vi "Q14070-Z060A.vi"() -> ()   [LabVIEW 2013]
uses:
  <vilib>/Utility/error.llb/whitespace.ctl
  <vilib>/Utility/file.llb/Read From Spreadsheet File (string).vi
  <vilib>/express/express arith-compare/Formula/XNode/ExpressFormulaBlockNode.xnode
  PCI8622_32.dll
  <vilib>/printing/EasyPrintingControls.llb/contents.ctl
  <vilib>/Utility/NIReport.llb/NI_ReportGenerationCore.lvlib
  <vilib>/printing/EasyPrintingControls.llb/report_type.ctl
  <vilib>/Utility/NIReport.llb/NI_report.lvclass
  <vilib>/printing/EasyPrinting.llb/Easy Print VI Panel or Documentation (path).vi
panel:
  in  "电动缸快速":dbl=15.0
  in  "电动缸慢速":dbl=1.0
  out "左轴向力数组大小":i32
  out "循环退出":bool
  in  "截取百分比":dbl=0.05
  in  "半行程":dbl=70.0
  in  "是否取消放行按钮":bool
  in  "齿条传动比":dbl=47.34 format="%#_13g"
  in  "机械间隙值":dbl=3.5
  out "最大轴向力标准(N)":dbl=200.0 caption="L+Lmax(mm)" format="%#.3f"
  out "右平均轴向力(N)":dbl caption="L+Lmax(mm)" format="%#.3f"
  out "左平均轴向力(N)":dbl caption="最大位移偏离Lmax(mm)" format="%#.3f"
  out "员工ID":string
  out "急停":bool
  out "报警":dbl
  out "报警提示":string
  out "DeviceHandle":u32
  in  "设定轴向力调整次数":dbl=6.0
  out "出支线工步号":u32
  in  "最小间隙(mm)":dbl=0.001 format="%#.3f"
  in  "测头气缸右移":bool
  in  "测头气缸左移":bool
  in  "轴向力已做次数":dbl
  out "全行程间隙及轴向力合格":bool
  out "轴向力启动":bool
  out "间隙启动":bool
  in  "夹头松开":bool
  in  "夹头夹紧":bool
  out "找帽扭矩":dbl=10.0 caption="压力传感器" format="%#.2f"
  out "error out":errorcluster
  out "型号数量":i32
  out "error out 4":errorcluster
  in  "设定间隙调整次数":dbl=6.0
  out "读取产品ID":string
  out "下工位备料":bool
  out "下工位测试":bool
  out "下工位自动":bool
  out "下工位备料H":bool
  out "下工位测试H":bool
  out "下工位自动H":bool
  out "FGCS":string
  out "KSJJ":string
  out "Z060ARFID":string
  out "轴向力Y":dbl[](array[numeric])
  out "轴向力X":dbl[](array[numeric])
  out "间隙X数组":dbl[](array[numeric])
  out "间隙Y数组":dbl[](array[numeric])
  out "error out 3":errorcluster caption="错误输出"
  out "rfid工步号":u32
  out "芯片ID":string="201209190001"
  out "rfid完成":bool
  out "rfid触发":bool
  out "本序已做":bool
  in  "回零完成":bool
  in  "电动缸回零":bool
  in  "已调试次数":dbl
  in  "需调整角度(度)":dbl
  in  "转向器中心":dbl
  out "扭矩到达":bool
  out "黄灯":bool
  out "红灯":bool
  in  "基准位移":dbl caption="压力传感器" format="%#.3f"
  out "上序不合格":bool
  out "单点间隙合格":bool
  out "上序合格":bool
  out "测头机构电机":u32
  out "复位":bool
  in  "型号选择":u16(ring)=1 items=["J709", "J728", "J706"]
  in  "联线按钮":bool
  in  "工步号":u32
  in  "产品ID":string="201209190001"
  out "间隙位移(mm)":dbl caption="压力传感器" format="%#.3f"
  out "齿条推拉力(N)":dbl format="%#.2f"
  out "齿条扭矩(Nm)":dbl format="%#.2f"
  out "通讯状态":bool
  out "员工姓名":string
  out "工步提示":string
  out "ADODB._Connection Out 2":refnum<k7>
  out "旋转齿条电机":u32
  out "电动缸电机":u32
  in  "停止":bool
  in  "参数加载":bool
  in  "选项卡控件":T1(tab)
  out "扭动曲线":cluster{"Y":dbl[], "Y":dbl[]}[](graph) caption="压球涨堵头1"
  out "中间位置间隙":dbl caption="间隙值L(mm)" format="%_2f"
  out "中间间隙标准(mm)":dbl=0.07 format="%#.3f"
  in  "找帽OK":bool
  out "全行程180°外间隙标准(mm)":dbl=0.1 format="%#.3f"
  out "右180°外全行程间隙":dbl caption="正向最大间隙L1(mm)" format="%_2f"
  out "左180°外全行程间隙":dbl caption="正向最大间隙L1(mm)" format="%_2f"
  out "右180°内全行程间隙":dbl caption="正向最大间隙L1(mm)" format="%_2f"
  out "左180°内全行程间隙":dbl caption="正向最大间隙L1(mm)" format="%_2f"
  out "全行程180°内间隙标准(mm)":dbl=0.07 format="%_1f"
  out "左全行程间隙":dbl caption="正向最大间隙L1(mm)" format="%#.3f"
  out "右全行程间隙":dbl caption="正向最大间隙L1(mm)" format="%#.3f"
  out "总圈数最大值":dbl format="%_3g"
  out "总圈数标准":dbl format="%_3g"
  out "总行程最大值":dbl
  out "总行程标准(mm)":dbl
  out "平均轴向力MAX(N)":dbl=200.0 caption="L+Lmax(mm)" format="%#.3f"
  out "力波动标准(N)":dbl=60.0 caption="L+Lmax(mm)" format="%#.3f"
  out "轴向力标准(N)":dbl=100.0 caption="L+Lmax(mm)" format="%#.3f"
  out "右最大轴向力(N)":dbl caption="L+Lmax(mm)" format="%#_5f"
  out "左轴向力波动(N)":dbl caption="最大位移偏离Lmax(mm)" format="%#_4f"
  out "左最大轴向力(N)":dbl caption="最大位移偏离Lmax(mm)" format="%#_5f"
  out "行程跳动曲线":cluster{"Y":dbl[], "Y":dbl[]}[](graph) caption="压球涨堵头1"
  out "右轴向力波动(N)":dbl format="%#_4f"
  out "总行程(mm)":dbl format="%#_5f"
  out "总圈数":dbl format="%.3g"
  in  "不合格品":bool
  in  "扭矩停止值":dbl=16.0
  in  "齿条右极限":dbl=-70.0 caption="压力传感器" format="%#.2f"
  in  "齿条左极限":dbl=-262.0 caption="压力传感器" format="%#.2f"
  in  "齿条移动速度":dbl=5.0 caption="压力传感器" format="%#.2f"
  in  "旋转伺服找帽转速":dbl=5.0 caption="压力传感器" format="%#.2f"
  in  "测量点扭矩":dbl=4.0 caption="压力传感器" format="%#.2f"
  in  "旋转伺服测量转速":dbl caption="压力传感器" format="%#.2f"
  in  "测头机构轴后退位":dbl=30.0 caption="压力传感器" format="%#.2f"
  in  "测头机构轴待检位":dbl caption="压力传感器" format="%#.2f"
  in  "测头机构轴检测位":dbl caption="压力传感器" format="%#.2f"
  in  "测头机构轴移动速度":dbl caption="压力传感器" format="%#.2f"
  out "点胶":bool
  in  "夹头松开":bool
  in  "夹头夹紧":bool
  in  "测头气缸右移":bool
  in  "测头气缸左移":bool
  in  "支线下降":bool
  in  "支线顶升":bool
  in  "出支线":bool
  in  "进支线":bool
  in  "主线下降":bool
  in  "主线顶升":bool
  in  "下阻挡器放行":bool
  in  "上阻挡器放行":bool
  out "夹头夹紧位":bool
  out "测头左位":bool
  out "测头右位":bool
  out "夹头松开":bool
  out "记号笔":bool
  in  "测头机构轴使能":bool
  in  "测头机构轴后退":bool
  in  "测头机构轴前进":bool
  in  "电动缸速度(mm/s)":dbl=10.0 format="%#.3f"
  out "电动缸位置(mm)":dbl=10000.0 format="%#.3f"
  in  "旋转伺服速度(°/s)":dbl=10.0 format="%#.3f"
  out "旋转伺服位置(°)":dbl=10000.0 format="%#.3f"
  in  "测头机构轴速度(mm/s)":dbl=10.0 format="%#.3f"
  out "测头机构轴位置(mm)":dbl=10000.0 format="%#.3f"
  in  "旋转齿条轴右转":bool
  in  "旋转齿条轴左转":bool
  in  "旋转齿条轴使能":bool
  in  "电动缸后退":bool
  in  "电动缸使能":bool
  in  "电动缸前进":bool
  in  "齿条扭矩比例偏移":dbl=1.0 format="%#.2f"
  in  "齿条扭矩零点偏移":dbl format="%#.2f"
  in  "齿条推拉力比例偏移":dbl=1.0 format="%#.2f"
  in  "齿条推拉力零点偏移":dbl format="%#.2f"
  in  "间隙位移比例偏移":dbl=1.0 format="%#.2f"
  in  "间隙位移零点偏移":dbl format="%#.2f"
  in  "传感器参数保存":bool
  in  "参数修改":bool
  in  "参数查询":bool
  in  "参数浏览表":string[][](table)
  # "芜湖机械转向器装配线"
  # "间隙及轴向力检测"
  # "Q14070机械转向器装配线"
  # "湖北唯思凌科装备制造有限公司 设计开发 (C)2015"
  # "≤"
  # "间隙测量判定值"
  # "间隙测量结果"
  # "≤"
  # "≤"
  # "≤"
  # "轴向力测量结果"
  # "轴向力测量标准"
  # "≤"
  # "≥"
  # "≤"
  # "≥"
  # "≤"
  # "≥"
  # "≤"
  # "不得大于20NM"
  # "传感器校验区"
  # "关于传感器校验：\n1、传感器校验需要由具备资质的单位或部门进行校验。\n2、具备权限的用户才能够修改传感器校验参数和试验参数。\n3、修改校验参数方法：先将比例偏移置为1，修改零点偏移，使零点值与校验的传感器一致；然后根据增幅调整比例偏移。"
  # "注意：\n具备权限的用户才能够修改传感器校验参数和试验参数！"
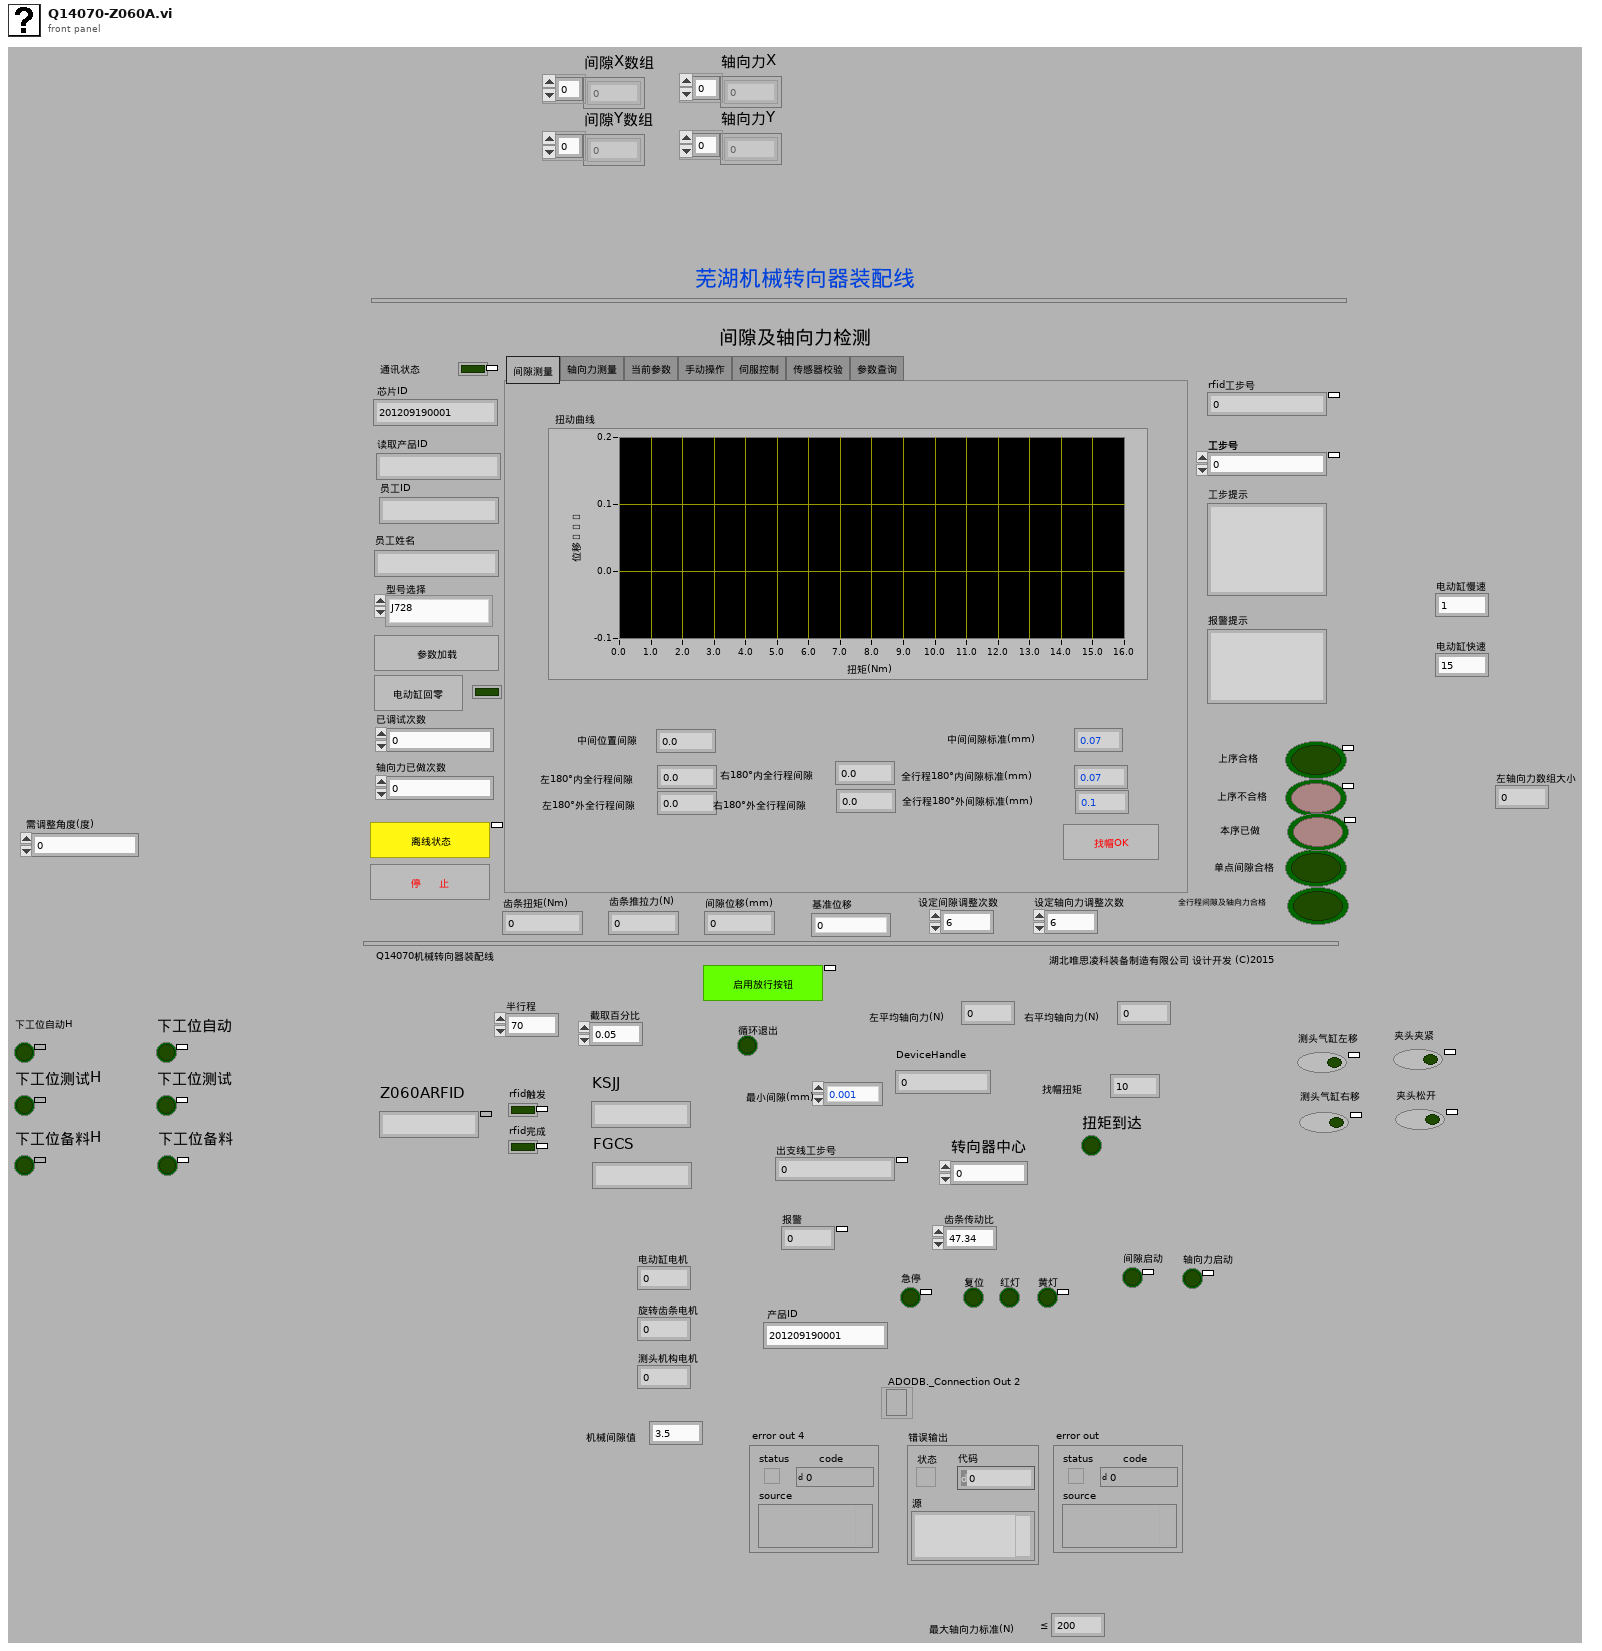
[diagram p1: front panel]
types:
  T1 = enum32{"间隙测量", "轴向力测量", "当前参数", "手动操作", "伺服控制", "传感器校验", "参数查询"}
  T2 = typedef "NI_ReportGenerationCore.lvlib/report_type.ctl" = u16
  T3 = typedef "NI_ReportGenerationCore.lvlib/contents.ctl" = u16
  T4 = typedef "imagedata.ctl" = cluster{"image type":i32, "image depth":i32, "image":u8[], "mask":u8[], "colors":u32[], "Rectangle":cluster{"left":i16, "top":i16, "right":i16, "bottom":i16}}
  T5 = enum8{"Enabled", "Disabled", "Disabled and Grayed Out"}
  T6 = typedef "whitespace.ctl" = u16
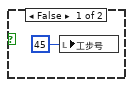
[diagram p2: hidden frame]
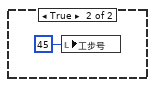
[diagram p3: hidden frame]
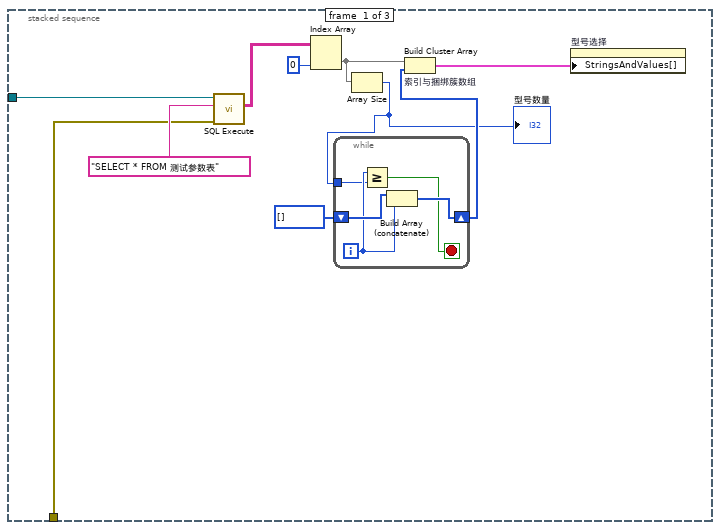
[diagram p6: hidden frame]
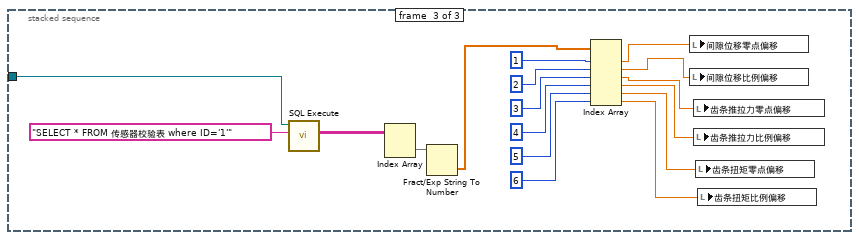
[diagram p7: hidden frame]
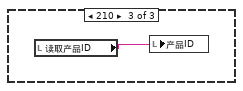
[diagram p9: hidden frame]
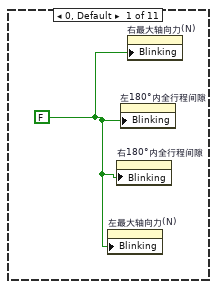
[diagram p10: hidden frame]
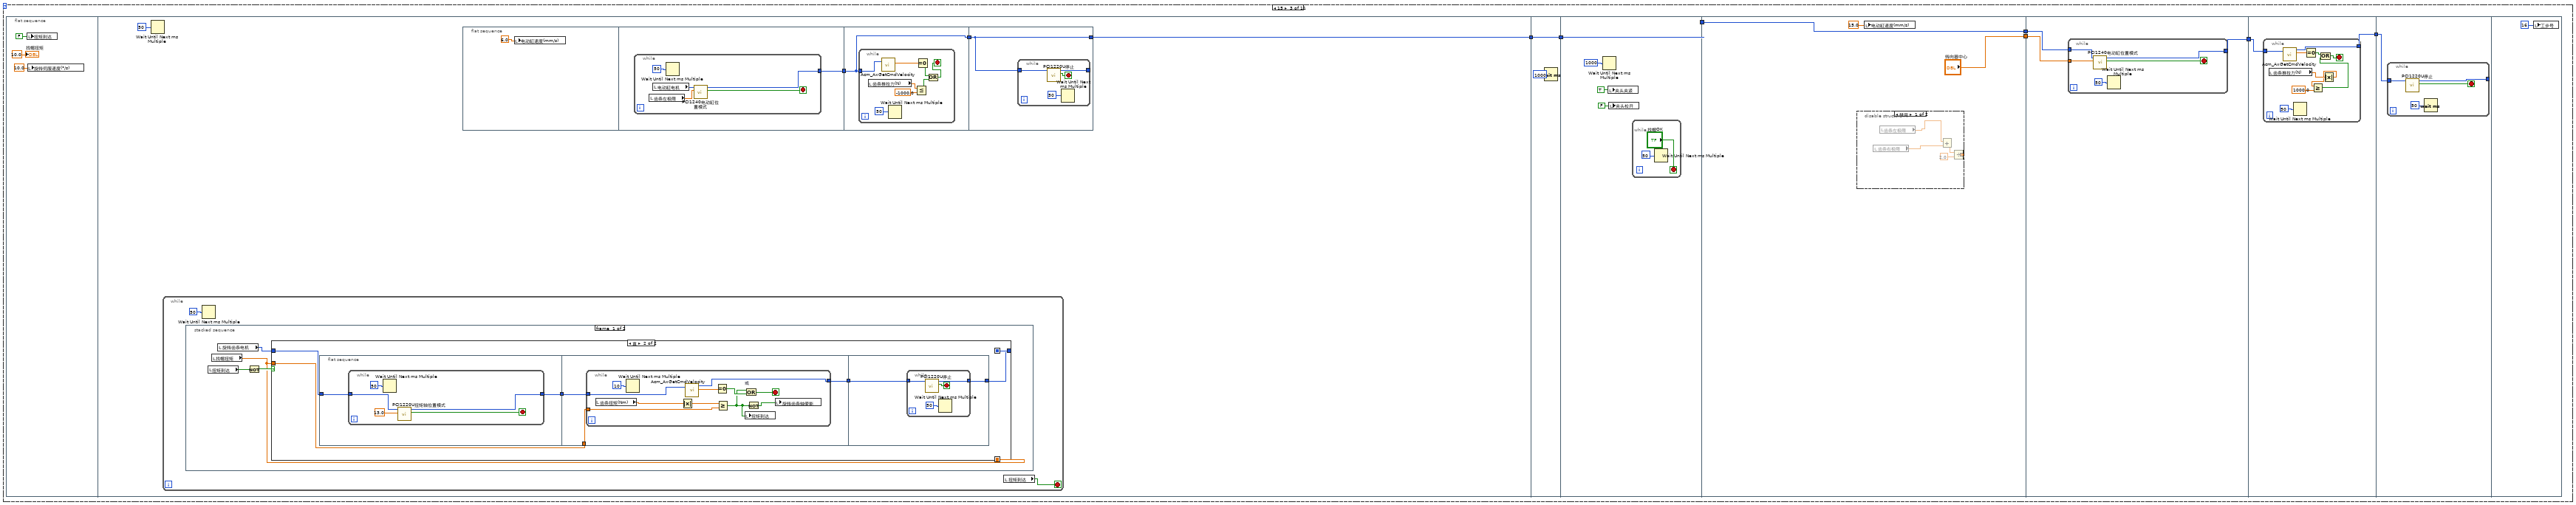
[diagram p11: hidden frame]
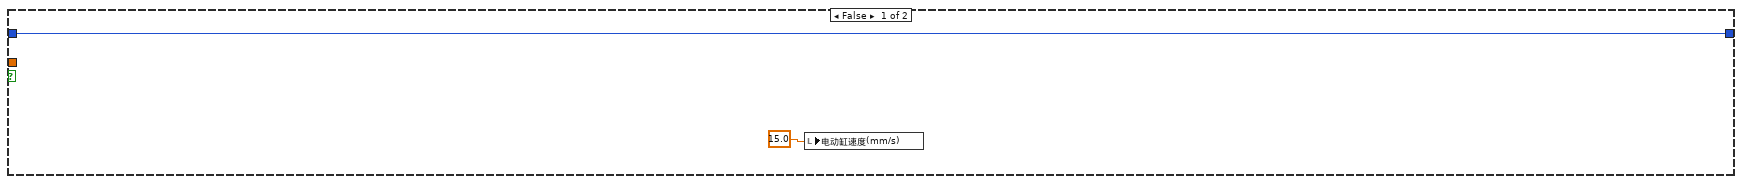
[diagram p12: hidden frame]
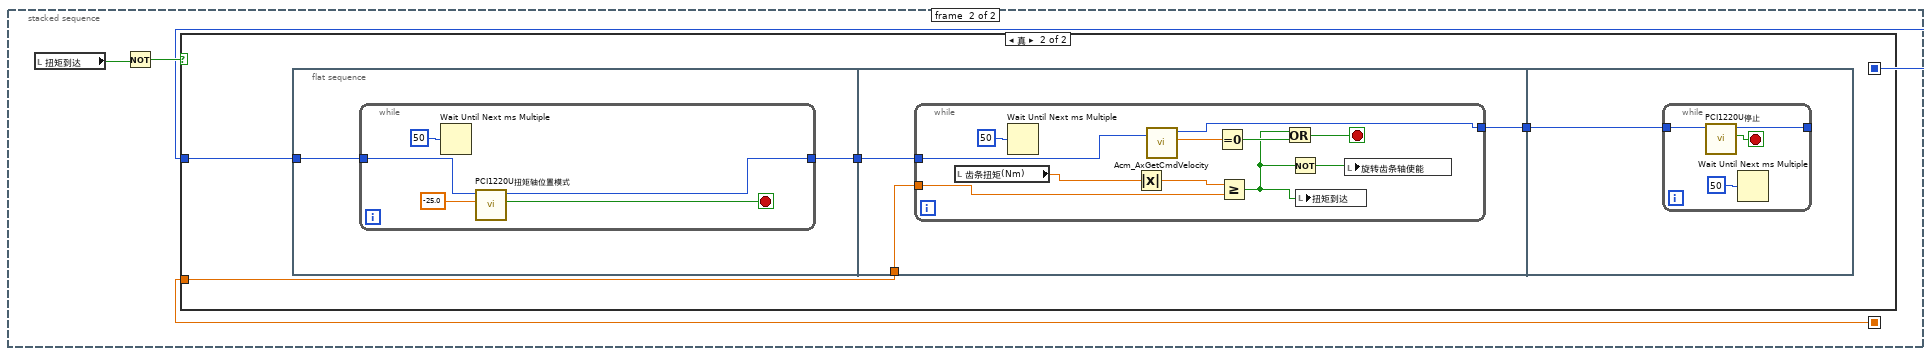
[diagram p13: hidden frame]
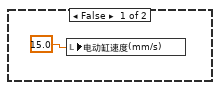
[diagram p14: hidden frame]
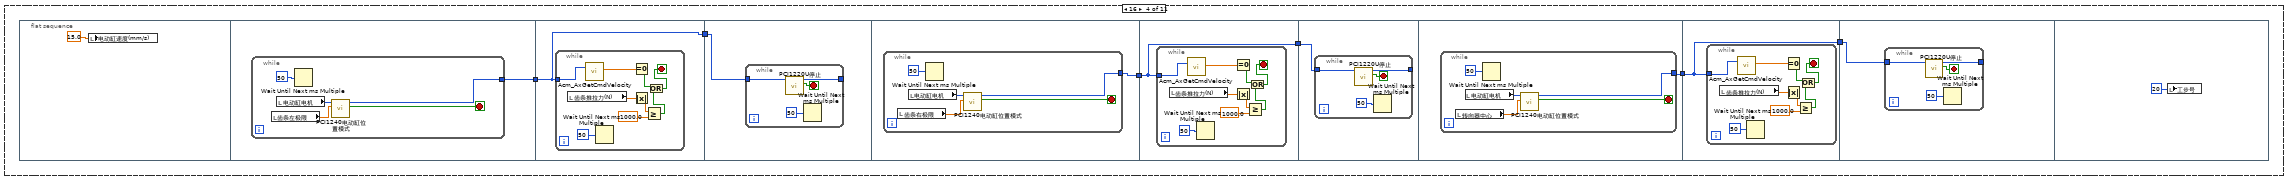
[diagram p16: hidden frame]
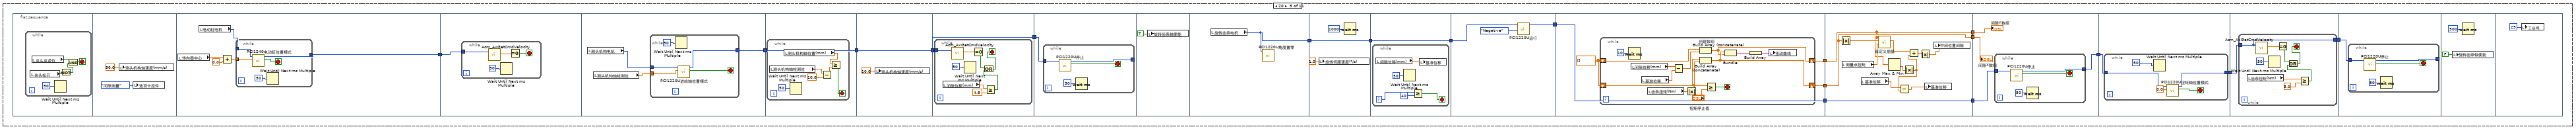
[diagram p17: hidden frame]
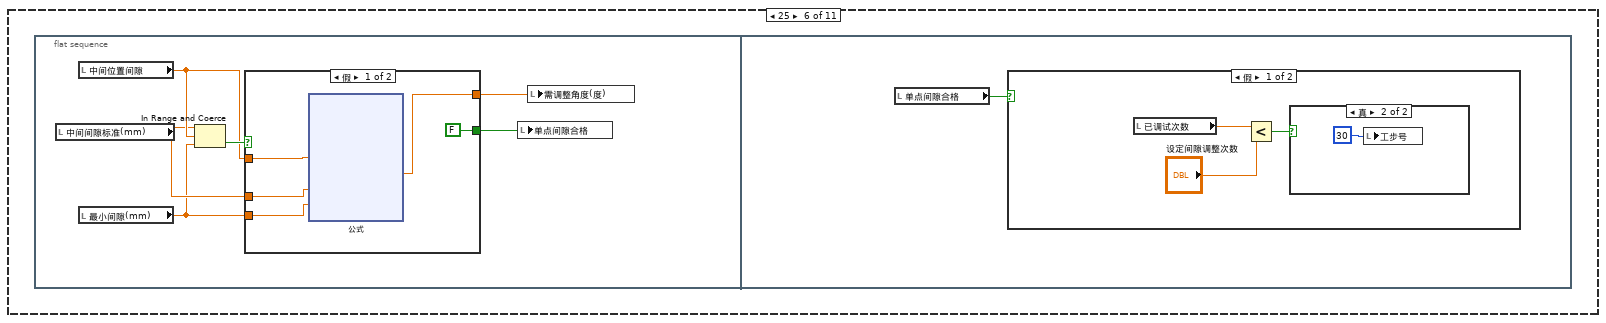
[diagram p18: hidden frame]
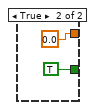
[diagram p19: hidden frame]
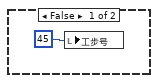
[diagram p20: hidden frame]
diagram:
  n1 = while {
    stop <- w133 stop-if-true
    n2 = local read "工步号"() -> (w131:u32)
    n3 = case shown="10" w131 {
      frame 0, Default {
        w134 = FALSE ("闪烁")
        n4 = property on="左最大轴向力(N)" class="DigNum (严格)"("Blinking"=w134) -> ()  [unwired: 2 in, 2 out]
        n5 = property on="右180°内全行程间隙" class="DigNum (严格)"("Blinking"=w134) -> ()  [unwired: 2 in, 2 out]
        n6 = property on="左180°内全行程间隙" class="DigNum (严格)"("Blinking"=w134) -> ()  [unwired: 2 in, 2 out]
        n7 = property on="右最大轴向力(N)" class="DigNum (严格)"("Blinking"=w134) -> ()  [unwired: 2 in, 2 out]
      }
      frame 10 {
        n8 = flat-sequence {
          frame #0 {
            w135 = FALSE ("单点间隙合格")
            w136 = 0.0 ("已调试次数")
            n9 = local write "电动缸速度(mm/s)"(10.0 ("电动缸速度(mm/s)")) -> ()
            n10 = local write "电动缸使能"(TRUE ("电动缸使能")) -> ()
            n11 = local write "旋转齿条轴使能"(TRUE ("旋转齿条轴使能")) -> ()
            n12 = local write "测头机构轴使能"(TRUE ("调整机构轴使能")) -> ()
            n13 = local write "旋转伺服速度(°/s)"(10.0 ("旋转齿条轴速度(°/s)")) -> ()
            n14 = local write "测头机构轴速度(mm/s)"(30.0 ("调整机构轴速度(mm/s)")) -> ()
            n15 = local write "已调试次数"(w136) -> ()
            n16 = local write "轴向力已做次数"(w136) -> ()
            n17 = property on="右180°外全行程间隙" class="DigNum (严格)"("Blinking"=w135) -> ()  [unwired: 2 in, 2 out]
            n18 = property on="左180°内全行程间隙" class="DigNum (严格)"("Blinking"=w135) -> ()  [unwired: 2 in, 2 out]
            n19 = property on="右180°内全行程间隙" class="DigNum (严格)"("Blinking"=w135) -> ()  [unwired: 2 in, 2 out]
            n20 = property on="左180°外全行程间隙" class="DigNum (严格)"("Blinking"=w135) -> ()  [unwired: 2 in, 2 out]
            n21 = property on="总行程(mm)" class="DigNum (严格)"("Blinking"=w135) -> ()  [unwired: 2 in, 2 out]
            n22 = local write "全行程间隙及轴向力合格"(w135) -> ()
            n23 = local write "单点间隙合格"(w135) -> ()
            n24 = local write "测头气缸右移"(TRUE ("测头气缸右移")) -> ()
            n25 = local write "测头气缸左移"(FALSE ("测头气缸左移")) -> ()
            n26 = property on="总圈数" class="DigNum (严格)"("Blinking"=w135) -> ()  [unwired: 2 in, 2 out]
            n27 = property on="左最大轴向力(N)" class="DigNum (严格)"("Blinking"=w135) -> ()  [unwired: 2 in, 2 out]
            n28 = property on="右最大轴向力(N)" class="DigNum (严格)"("Blinking"=w135) -> ()  [unwired: 2 in, 2 out]
            n29 = property on="右轴向力波动(N)" class="DigNum (严格)"("Blinking"=w135) -> ()  [unwired: 2 in, 2 out]
            n30 = property on="左轴向力波动(N)" class="DigNum (严格)"("Blinking"=w135) -> ()  [unwired: 2 in, 2 out]
          }
          frame #1 {
            n31 = while {
              stop <- w145 stop-if-true
              n32 = Wait Until Next ms Multiple(millisecond multiple=u32 50 ("毫秒倍数")) -> ()  [unwired: 1 out]
              n33 = local read "测头右位"() -> (w146:bool)
              n34 = local read "回零完成"() -> (w147:bool)
              n35 = And(x=w147, y=w146) -> (x .and. y?=w145:bool)
            }
          }
          frame #2 {
            n36 = Wait (ms)(milliseconds to wait=u32 1000 ("等待时间（毫秒）")) -> ()  [unwired: 1 out]
          }
          frame #3 {
            n37 = while {
              stop <- w153 stop-if-true
              n38 = local read "测头机构轴待检位"() -> (w150:dbl)
              n39 = local read "测头机构电机"() -> (w151:u32)
              n40 = call "PCI1220U进给轴位置模式.vi"("Distance"=w150, "AxisHandle IN"=w151) -> ("AbsSuccess"=w153:bool)  [unwired: 8 in, 1 out]
              n41 = Wait Until Next ms Multiple(millisecond multiple=u32 50 ("毫秒倍数")) -> ()  [unwired: 1 out]
            }
          }
          frame #4 {
            n42 = while {
              stop <- w156 stop-if-true
              n43 = local read "测头机构电机"() -> (w154:u32)
              n44 = Wait Until Next ms Multiple(millisecond multiple=u32 50 ("毫秒倍数")) -> ()  [unwired: 1 out]
              n45 = call <userlib>:"Acm_AxGetCmdVelocity.vi"("AxisHandle"=w154) -> ("Velocity"=w157:dbl)  [unwired: 1 in, 3 out]
              n46 = Equal To 0?(x=w157) -> (x = 0?=w156:bool)
            }
          }
          frame #5 {
            n47 = local write "工步号"(u32 15 ("工步号")) -> ()
          }
        }
      }
      frame 15 {
        n48 = flat-sequence {
          tunnel: [w170] -> w160
          tunnel: w160 -> [w271]
          tunnel: [w271] -> w159
          tunnel: w159 -> [w274]
          tunnel: [w274] -> w162
          tunnel: [w279] -> w165
          tunnel: ["转向器中心"] -> w164
          tunnel: w162 -> [w279]
          tunnel: w165 -> [w288]
          tunnel: w164 -> [w287]
          tunnel: [w286] -> w163
          tunnel: w163 -> [w295]
          tunnel: [w294] -> w161
          tunnel: w161 -> [w306]
          frame #0 {
            n49 = local write "扭矩到达"(FALSE ("扭矩到达")) -> ()
            n50 = local write "旋转伺服速度(°/s)"(10.0 ("旋转齿条轴速度(°/s)")) -> ()
            "找帽扭矩" <- 10.0 ("找帽扭矩")
          }
          frame #1 {
            n51 = Wait Until Next ms Multiple(millisecond multiple=u32 50 ("毫秒倍数")) -> ()  [unwired: 1 out]
            n52 = while {
              stop <- w173 stop-if-true
              n53 = stacked-sequence {
                seq-local: [w175 _] -> [_ w216]
                seq-local: [w179 _] -> [_ w215]
                frame #0 {
                  n54 = local read "扭矩到达"() -> (w177:bool)
                  n55 = local read "找帽扭矩"() -> (w175:dbl)
                  n56 = local read "旋转齿条电机"() -> (w176:u32)
                  n57 = Not(x=w177) -> (.not. x?=w178:bool)
                  n58 = case shown="真" w178 {
                    tunnel: [w181 w182] -> w179
                    tunnel: w176 -> [w181 w186]
                    tunnel: w175 -> [_ w184]
                    frame False {
                      n59 = local write "电动缸速度(mm/s)"(15.0 ("电动缸速度(mm/s)")) -> ()
                    }
                    frame True {
                      n60 = flat-sequence {
                        tunnel: w186 -> [w188]
                        tunnel: [w187] -> w185
                        tunnel: w185 -> [w196]
                        tunnel: w184 -> [w195]
                        tunnel: [w194] -> w183
                        tunnel: w183 -> [w209]
                        tunnel: [w208] -> w182
                        frame #0 {
                          n61 = while {
                            tunnel: [w192] -> w187
                            tunnel: w188 -> [w189]
                            stop <- w191 stop-if-true
                            n62 = Wait Until Next ms Multiple(millisecond multiple=u32 50 ("毫秒倍数")) -> ()  [unwired: 1 out]
                            n63 = call "PCI1220U扭矩轴位置模式.vi"("Distance"=13.0, "AxisHandle IN"=w189) -> ("AbsSuccess"=w191:bool, "AxisHandle OUT"=w192:u32)  [unwired: 8 in]
                          }
                        }
                        frame #1 {
                          n64 = while {
                            tunnel: w196 -> [w206]
                            tunnel: w195 -> [w201]
                            tunnel: [w200] -> w194
                            stop <- w202 stop-if-true
                            n65 = local read "齿条扭矩(Nm)"() -> (w199:dbl)
                            n66 = Wait Until Next ms Multiple(millisecond multiple=u32 10 ("毫秒倍数")) -> ()  [unwired: 1 out]
                            n67 = Absolute Value(x=w199) -> (abs(x)=w204:dbl)
                            n68 = call <userlib>:"Acm_AxGetCmdVelocity.vi"("AxisHandle"=w206) -> ("Velocity"=w205:dbl, "AxisHandle"=w200:u32)  [unwired: 1 in, 2 out]
                            n69 = Equal To 0?(x=w205) -> (x = 0?=w203:bool)
                            n70 = Greater Or Equal?(x=w204, y=w201) -> (x >= y?=w198:bool)
                            n71 = Or "或"(x=w198, y=w203) -> (x .or. y?=w202:bool)
                            n72 = local write "扭矩到达"(w198) -> ()
                            n73 = Not(x=w198) -> (.not. x?=w197:bool)
                            n74 = local write "旋转齿条轴使能"(w197) -> ()
                          }
                        }
                        frame #2 {
                          n75 = while {
                            tunnel: w209 -> [w213]
                            tunnel: [w210] -> w208
                            stop <- w212 stop-if-true
                            n76 = call "PCI1220U停止.vi"("AxisHandle IN"=w213) -> ("完成"=w212:bool, "AxisHandle OUT"=w210:u32)  [unwired: 9 in]
                            n77 = Wait Until Next ms Multiple(millisecond multiple=u32 50 ("毫秒倍数")) -> ()  [unwired: 1 out]
                          }
                        }
                      }
                    }
                  }
                }
                frame #1 {
                  n78 = local read "扭矩到达"() -> (w214:bool)
                  n79 = Not(x=w214) -> (.not. x?=w217:bool)
                  n80 = case shown="真" w217 {
                    tunnel: w215 -> [_ w222]
                    tunnel: w216 -> [_ w220]
                    frame False {
                      n81 = local write "电动缸速度(mm/s)"(15.0 ("电动缸速度(mm/s)")) -> ()
                    }
                    frame True {
                      n82 = flat-sequence {
                        tunnel: w222 -> [w223]
                        tunnel: [w224] -> w221
                        tunnel: w221 -> [w232]
                        tunnel: w220 -> [w231]
                        tunnel: [w230] -> w219
                        tunnel: w219 -> [w244]
                        frame #0 {
                          n83 = while {
                            tunnel: [w228] -> w224
                            tunnel: w223 -> [w225]
                            stop <- w227 stop-if-true
                            n84 = Wait Until Next ms Multiple(millisecond multiple=u32 50 ("毫秒倍数")) -> ()  [unwired: 1 out]
                            n85 = call "PCI1220U扭矩轴位置模式.vi"("Distance"=-25.0, "AxisHandle IN"=w225) -> ("AbsSuccess"=w227:bool, "AxisHandle OUT"=w228:u32)  [unwired: 8 in]
                          }
                        }
                        frame #1 {
                          n86 = while {
                            tunnel: w232 -> [w242]
                            tunnel: [w237] -> w230
                            tunnel: w231 -> [w236]
                            stop <- w238 stop-if-true
                            n87 = local read "齿条扭矩(Nm)"() -> (w235:dbl)
                            n88 = Wait Until Next ms Multiple(millisecond multiple=u32 50 ("毫秒倍数")) -> ()  [unwired: 1 out]
                            n89 = Absolute Value(x=w235) -> (abs(x)=w240:dbl)
                            n90 = call <userlib>:"Acm_AxGetCmdVelocity.vi"("AxisHandle"=w242) -> ("Velocity"=w241:dbl, "AxisHandle"=w237:u32)  [unwired: 1 in, 2 out]
                            n91 = Equal To 0?(x=w241) -> (x = 0?=w239:bool)
                            n92 = Greater Or Equal?(x=w240, y=w236) -> (x >= y?=w233:bool)
                            n93 = Or(x=w233, y=w239) -> (x .or. y?=w238:bool)
                            n94 = Not(x=w233) -> (.not. x?=w234:bool)
                            n95 = local write "扭矩到达"(w233) -> ()
                            n96 = local write "旋转齿条轴使能"(w234) -> ()
                          }
                        }
                        frame #2 {
                          n97 = while {
                            tunnel: w244 -> [w248]
                            tunnel: [w245] -> _
                            stop <- w247 stop-if-true
                            n98 = call "PCI1220U停止.vi"("AxisHandle IN"=w248) -> ("完成"=w247:bool, "AxisHandle OUT"=w245:u32)  [unwired: 9 in]
                            n99 = Wait Until Next ms Multiple(millisecond multiple=u32 50 ("毫秒倍数")) -> ()  [unwired: 1 out]
                          }
                        }
                      }
                    }
                  }
                }
              }
              n100 = Wait Until Next ms Multiple(millisecond multiple=u32 50 ("毫秒倍数")) -> ()  [unwired: 1 out]
              n101 = local read "扭矩到达"() -> (w173:bool)
            }
            n102 = flat-sequence {
              tunnel: [w250] -> w172
              tunnel: w172 -> [w256]
              tunnel: [w256] -> w169
              tunnel: [w265] -> w170
              tunnel: w169 -> [w265]
              frame #0 {
                n103 = local write "电动缸速度(mm/s)"(6.0 ("电动缸速度(mm/s)")) -> ()
              }
              frame #1 {
                n104 = while {
                  tunnel: [w254] -> w250
                  stop <- w253 stop-if-true
                  n105 = local read "齿条左极限"() -> (w251:dbl)
                  n106 = local read "电动缸电机"() -> (w255:u32)
                  n107 = Wait Until Next ms Multiple(millisecond multiple=u32 50 ("毫秒倍数")) -> ()  [unwired: 1 out]
                  n108 = call "PCI1240电动缸位置模式 .vi"("Distance"=w251, "AxisHandle IN"=w255) -> ("AbsSuccess"=w253:bool, "AxisHandle OUT"=w254:u32)  [unwired: 8 in]
                }
              }
              frame #2 {
                n109 = while {
                  tunnel: w256 -> [w263]
                  stop <- w260 stop-if-true
                  n110 = local read "齿条推拉力(N)"() -> (w259:dbl)
                  n111 = call <userlib>:"Acm_AxGetCmdVelocity.vi"("AxisHandle"=w263) -> ("Velocity"=w264:dbl)  [unwired: 1 in, 3 out]
                  n112 = Wait Until Next ms Multiple(millisecond multiple=u32 50 ("毫秒倍数")) -> ()  [unwired: 1 out]
                  n113 = Less Or Equal?(x=w259, y=-1000.0) -> (x <= y?=w257:bool)
                  n114 = Equal To 0?(x=w264) -> (x = 0?=w261:bool)
                  n115 = Or(x=w261, y=w257) -> (x .or. y?=w260:bool)
                }
              }
              frame #3 {
                n116 = while {
                  tunnel: w265 -> [w269]
                  tunnel: [w266] -> _
                  stop <- w268 stop-if-true
                  n117 = call "PCI1220U停止.vi"("AxisHandle IN"=w269) -> ("完成"=w268:bool, "AxisHandle OUT"=w266:u32)  [unwired: 9 in]
                  n118 = Wait Until Next ms Multiple(millisecond multiple=u32 50 ("毫秒倍数")) -> ()  [unwired: 1 out]
                }
              }
            }
          }
          frame #2 {
            n119 = Wait (ms)(milliseconds to wait=u32 1000 ("等待时间（毫秒）")) -> ()  [unwired: 1 out]
          }
          frame #3 {
            n120 = Wait Until Next ms Multiple(millisecond multiple=u32 1000 ("毫秒倍数")) -> ()  [unwired: 1 out]
            n121 = local write "夹头夹紧"(TRUE ("夹头夹紧")) -> ()
            n122 = local write "夹头松开"(FALSE ("夹头松开")) -> ()
            n123 = while {
              stop <- "找帽OK" stop-if-true
              n124 = Wait Until Next ms Multiple(millisecond multiple=u32 50 ("毫秒倍数")) -> ()  [unwired: 1 out]
            }
          }
          frame #4 {
            n125 = disable-structure shown="禁用" {
              disable-tunnel: [w283 _] -> _
              frame Disabled {
                n126 = local read "齿条右极限"() -> (w281:dbl)
                n127 = local read "齿条左极限"() -> (w282:dbl)
                n128 = Add(x=w282, y=w281) -> (x+y=w285:dbl)
                n129 = Divide(x=w285, y=2.0) -> (x/y=w283:dbl)
              }
              frame Enabled {
              }
            }
            n130 = local write "电动缸速度(mm/s)"(15.0 ("电动缸轴移动速度")) -> ()
          }
          frame #5 {
            n131 = while {
              tunnel: w288 -> [w293]
              tunnel: w287 -> [w292]
              tunnel: [w289] -> w286
              stop <- w291 stop-if-true
              n132 = call "PCI1240电动缸位置模式 .vi"("Distance"=w292, "AxisHandle IN"=w293) -> ("AbsSuccess"=w291:bool, "AxisHandle OUT"=w289:u32)  [unwired: 8 in]
              n133 = Wait Until Next ms Multiple(millisecond multiple=u32 50 ("毫秒倍数")) -> ()  [unwired: 1 out]
            }
          }
          frame #6 {
            n134 = while {
              tunnel: w295 -> [w305]
              tunnel: [w296] -> w294
              stop <- w297 stop-if-true
              n135 = local read "齿条推拉力(N)"() -> (w302:dbl)
              n136 = call <userlib>:"Acm_AxGetCmdVelocity.vi"("AxisHandle"=w305) -> ("Velocity"=w304:dbl, "AxisHandle"=w296:u32)  [unwired: 1 in, 2 out]
              n137 = Wait Until Next ms Multiple(millisecond multiple=u32 50 ("毫秒倍数")) -> ()  [unwired: 1 out]
              n138 = Equal To 0?(x=w304) -> (x = 0?=w299:bool)
              n139 = Absolute Value(x=w302) -> (abs(x)=w301:dbl)
              n140 = Greater Or Equal?(x=w301, y=1000.0) -> (x >= y?=w298:bool)
              n141 = Or(x=w299, y=w298) -> (x .or. y?=w297:bool)
            }
          }
          frame #7 {
            n142 = while {
              tunnel: w306 -> [w310]
              tunnel: [w309] -> _
              stop <- w308 stop-if-true
              n143 = call "PCI1220U停止.vi"("AxisHandle IN"=w310) -> ("完成"=w308:bool, "AxisHandle OUT"=w309:u32)  [unwired: 9 in]
              n144 = Wait (ms)(milliseconds to wait=u32 50 ("毫秒倍数")) -> ()  [unwired: 1 out]
            }
          }
          frame #8 {
            n145 = local write "工步号"(u32 16 ("工步号")) -> ()
          }
        }
      }
      frame 16 {
        n146 = flat-sequence {
          tunnel: [w319] -> w317
          tunnel: w317 -> [w325]
          tunnel: [w325] -> w316
          tunnel: w316 -> [w335]
          tunnel: [w340] -> w315
          tunnel: w315 -> [w346]
          tunnel: [w346] -> w314
          tunnel: w314 -> [w356]
          tunnel: [w361] -> w313
          tunnel: w313 -> [w367]
          tunnel: [w367] -> w312
          tunnel: w312 -> [w377]
          frame #0 {
            n147 = local write "电动缸速度(mm/s)"(15.0 ("电动缸速度(mm/s)")) -> ()
          }
          frame #1 {
            n148 = while {
              tunnel: [w323] -> w319
              stop <- w322 stop-if-true
              n149 = local read "齿条左极限"() -> (w320:dbl)
              n150 = local read "电动缸电机"() -> (w324:u32)
              n151 = Wait Until Next ms Multiple(millisecond multiple=u32 50 ("毫秒倍数")) -> ()  [unwired: 1 out]
              n152 = call "PCI1240电动缸位置模式 .vi"("Distance"=w320, "AxisHandle IN"=w324) -> ("AbsSuccess"=w322:bool, "AxisHandle OUT"=w323:u32)  [unwired: 8 in]
            }
          }
          frame #2 {
            n153 = while {
              tunnel: w325 -> [w333]
              stop <- w330 stop-if-true
              n154 = local read "齿条推拉力(N)"() -> (w329:dbl)
              n155 = call <userlib>:"Acm_AxGetCmdVelocity.vi"("AxisHandle"=w333) -> ("Velocity"=w334:dbl)  [unwired: 1 in, 3 out]
              n156 = Wait Until Next ms Multiple(millisecond multiple=u32 50 ("毫秒倍数")) -> ()  [unwired: 1 out]
              n157 = Equal To 0?(x=w334) -> (x = 0?=w331:bool)
              n158 = Absolute Value(x=w329) -> (abs(x)=w328:dbl)
              n159 = Greater Or Equal?(x=w328, y=1000.0) -> (x >= y?=w326:bool)
              n160 = Or(x=w331, y=w326) -> (x .or. y?=w330:bool)
            }
          }
          frame #3 {
            n161 = while {
              tunnel: w335 -> [w339]
              tunnel: [w336] -> _
              stop <- w338 stop-if-true
              n162 = call "PCI1220U停止.vi"("AxisHandle IN"=w339) -> ("完成"=w338:bool, "AxisHandle OUT"=w336:u32)  [unwired: 9 in]
              n163 = Wait Until Next ms Multiple(millisecond multiple=u32 50 ("毫秒倍数")) -> ()  [unwired: 1 out]
            }
          }
          frame #4 {
            n164 = while {
              tunnel: [w344] -> w340
              stop <- w343 stop-if-true
              n165 = local read "齿条右极限"() -> (w341:dbl)
              n166 = local read "电动缸电机"() -> (w345:u32)
              n167 = Wait Until Next ms Multiple(millisecond multiple=u32 50 ("毫秒倍数")) -> ()  [unwired: 1 out]
              n168 = call "PCI1240电动缸位置模式 .vi"("Distance"=w341, "AxisHandle IN"=w345) -> ("AbsSuccess"=w343:bool, "AxisHandle OUT"=w344:u32)  [unwired: 8 in]
            }
          }
          frame #5 {
            n169 = while {
              tunnel: w346 -> [w354]
              stop <- w351 stop-if-true
              n170 = local read "齿条推拉力(N)"() -> (w350:dbl)
              n171 = call <userlib>:"Acm_AxGetCmdVelocity.vi"("AxisHandle"=w354) -> ("Velocity"=w355:dbl)  [unwired: 1 in, 3 out]
              n172 = Wait Until Next ms Multiple(millisecond multiple=u32 50 ("毫秒倍数")) -> ()  [unwired: 1 out]
              n173 = Equal To 0?(x=w355) -> (x = 0?=w352:bool)
              n174 = Absolute Value(x=w350) -> (abs(x)=w349:dbl)
              n175 = Greater Or Equal?(x=w349, y=1000.0) -> (x >= y?=w347:bool)
              n176 = Or(x=w352, y=w347) -> (x .or. y?=w351:bool)
            }
          }
          frame #6 {
            n177 = while {
              tunnel: w356 -> [w360]
              tunnel: [w357] -> _
              stop <- w359 stop-if-true
              n178 = call "PCI1220U停止.vi"("AxisHandle IN"=w360) -> ("完成"=w359:bool, "AxisHandle OUT"=w357:u32)  [unwired: 9 in]
              n179 = Wait Until Next ms Multiple(millisecond multiple=u32 50 ("毫秒倍数")) -> ()  [unwired: 1 out]
            }
          }
          frame #7 {
            n180 = while {
              tunnel: [w365] -> w361
              stop <- w364 stop-if-true
              n181 = local read "转向器中心"() -> (w362:dbl)
              n182 = local read "电动缸电机"() -> (w366:u32)
              n183 = Wait Until Next ms Multiple(millisecond multiple=u32 50 ("毫秒倍数")) -> ()  [unwired: 1 out]
              n184 = call "PCI1240电动缸位置模式 .vi"("Distance"=w362, "AxisHandle IN"=w366) -> ("AbsSuccess"=w364:bool, "AxisHandle OUT"=w365:u32)  [unwired: 8 in]
            }
          }
          frame #8 {
            n185 = while {
              tunnel: w367 -> [w375]
              stop <- w372 stop-if-true
              n186 = local read "齿条推拉力(N)"() -> (w371:dbl)
              n187 = call <userlib>:"Acm_AxGetCmdVelocity.vi"("AxisHandle"=w375) -> ("Velocity"=w376:dbl)  [unwired: 1 in, 3 out]
              n188 = Wait Until Next ms Multiple(millisecond multiple=u32 50 ("毫秒倍数")) -> ()  [unwired: 1 out]
              n189 = Equal To 0?(x=w376) -> (x = 0?=w373:bool)
              n190 = Absolute Value(x=w371) -> (abs(x)=w370:dbl)
              n191 = Greater Or Equal?(x=w370, y=1000.0) -> (x >= y?=w368:bool)
              n192 = Or(x=w373, y=w368) -> (x .or. y?=w372:bool)
            }
          }
          frame #9 {
            n193 = while {
              tunnel: w377 -> [w381]
              tunnel: [w378] -> _
              stop <- w380 stop-if-true
              n194 = call "PCI1220U停止.vi"("AxisHandle IN"=w381) -> ("完成"=w380:bool, "AxisHandle OUT"=w378:u32)  [unwired: 9 in]
              n195 = Wait Until Next ms Multiple(millisecond multiple=u32 50 ("毫秒倍数")) -> ()  [unwired: 1 out]
            }
          }
          frame #10 {
            n196 = local write "工步号"(u32 20 ("工步号")) -> ()
          }
        }
      }
      frame 20 {
        n197 = flat-sequence {
          tunnel: [w412] -> w393
          tunnel: w393 -> [w418]
          tunnel: [w424] -> w385
          tunnel: w385 -> [w431]
          tunnel: [w431] -> w384
          tunnel: w384 -> [w439]
          tunnel: [w439] -> w383
          tunnel: w383 -> [w440]
          tunnel: [w440] -> w392
          tunnel: w392 -> [w449]
          tunnel: [w455] -> w390
          tunnel: [w457] -> w391
          tunnel: w390 -> [w457]
          tunnel: [w459] -> w386
          tunnel: w391 -> [w459]
          tunnel: w386 -> [w466]
          tunnel: [w465] -> w397
          tunnel: [w470] -> w396
          tunnel: [w469] -> w395
          tunnel: w397 -> [w468]
          tunnel: [w468] -> w394
          tunnel: [w497] -> w400
          tunnel: [w494] -> w399
          tunnel: w396 -> [w494]
          tunnel: [w493] -> w398
          tunnel: w395 -> [w493]
          tunnel: w394 -> [w497]
          tunnel: w400 -> [w501]
          tunnel: [w500] -> w389
          tunnel: w399 -> [w498]
          tunnel: w398 -> [w499]
          tunnel: w389 -> [w507]
          tunnel: [w506] -> w388
          tunnel: w388 -> [w514]
          tunnel: [w513] -> w387
          tunnel: w387 -> [w523]
          frame #0 {
            n198 = while {
              stop <- w403 stop-if-true
              n199 = local read "夹头松开"() -> (w404:bool)
              n200 = local read "夹头夹紧位"() -> (w402:bool)
              n201 = Wait Until Next ms Multiple(millisecond multiple=u32 50 ("毫秒倍数")) -> ()  [unwired: 1 out]
              n202 = Not(x=w404) -> (.not. x?=w401:bool)
              n203 = And(x=w402, y=w401) -> (x .and. y?=w403:bool)
            }
          }
          frame #1 {
            n204 = local write "测头机构轴速度(mm/s)"(30.0 ("测头机构轴速度(mm/s)")) -> ()
            n205 = local write "选项卡控件"(T1."间隙测量" ("选项卡控件")) -> ()
          }
          frame #2 {
            n206 = local read "转向器中心"() -> (w410:dbl)
            n207 = local read "电动缸电机"() -> (w411:u32)
            n208 = Add(x=w410, y=0.0) -> (x+y=w409:dbl)
            n209 = while {
              tunnel: w411 -> [w417]
              tunnel: w409 -> [w416]
              tunnel: [w413] -> w412
              stop <- w415 stop-if-true
              n210 = call "PCI1240电动缸位置模式 .vi"("Distance"=w416, "AxisHandle IN"=w417) -> ("AbsSuccess"=w415:bool, "AxisHandle OUT"=w413:u32)  [unwired: 8 in]
              n211 = Wait Until Next ms Multiple(millisecond multiple=u32 50 ("毫秒倍数")) -> ()  [unwired: 1 out]
            }
          }
          frame #3 {
            n212 = while {
              tunnel: w418 -> [w422]
              stop <- w420 stop-if-true
              n213 = call <userlib>:"Acm_AxGetCmdVelocity.vi"("AxisHandle"=w422) -> ("Velocity"=w421:dbl)  [unwired: 1 in, 3 out]
              n214 = Wait Until Next ms Multiple(millisecond multiple=u32 50 ("毫秒倍数")) -> ()  [unwired: 1 out]
              n215 = Equal To 0?(x=w421) -> (x = 0?=w420:bool)
            }
          }
          frame #4 {
            n216 = local read "测头机构电机"() -> (w425:u32)
            n217 = local read "测头机构轴检测位"() -> (w423:dbl)
            n218 = while {
              tunnel: w425 -> [w428]
              tunnel: w423 -> [w427]
              tunnel: [w426] -> w424
              stop <- w430 stop-if-true
              n219 = Wait Until Next ms Multiple(millisecond multiple=u32 50 ("毫秒倍数")) -> ()  [unwired: 1 out]
              n220 = call "PCI1220U进给轴位置模式.vi"("Distance"=w427, "AxisHandle IN"=w428) -> ("AbsSuccess"=w430:bool, "AxisHandle OUT"=w426:u32)  [unwired: 8 in]
            }
          }
          frame #5 {
            n221 = while {
              stop <- w432 stop-if-true
              n222 = local read "测头机构轴检测位"() -> (w436:dbl)
              n223 = local read "测头机构轴位置(mm)"() -> (w435:dbl)
              n224 = Wait Until Next ms Multiple(millisecond multiple=u32 50 ("毫秒倍数")) -> ()  [unwired: 1 out]
              n225 = Subtract(x=w436, y=10.0) -> (x-y=w433:dbl)
              n226 = Greater Or Equal?(x=w435, y=w433) -> (x >= y?=w432:bool)
            }
          }
          frame #6 {
            n227 = local write "测头机构轴速度(mm/s)"(10.0 ("测头机构轴速度(mm/s)")) -> ()
          }
          frame #7 {
            n228 = while {
              tunnel: w440 -> [w448]
              stop <- w442 stop-if-true
              n229 = local read "间隙位移(mm)"() -> (w445:dbl)
              n230 = call <userlib>:"Acm_AxGetCmdVelocity.vi"("AxisHandle"=w448) -> ("Velocity"=w447:dbl)  [unwired: 1 in, 3 out]
              n231 = Wait Until Next ms Multiple(millisecond multiple=u32 50 ("毫秒倍数")) -> ()  [unwired: 1 out]
              n232 = Equal To 0?(x=w447) -> (x = 0?=w443:bool)
              n233 = Greater Or Equal?(x=w445, y=4.5) -> (x >= y?=w441:bool)
              n234 = Or(x=w443, y=w441) -> (x .or. y?=w442:bool)
            }
          }
          frame #8 {
            n235 = while {
              tunnel: w449 -> [w453]
              tunnel: [w452] -> _
              stop <- w451 stop-if-true
              n236 = call "PCI1220U停止.vi"("AxisHandle IN"=w453) -> ("完成"=w451:bool, "AxisHandle OUT"=w452:u32)  [unwired: 9 in]
              n237 = Wait (ms)(milliseconds to wait=u32 50 ("毫秒倍数")) -> ()  [unwired: 1 out]
            }
          }
          frame #9 {
            n238 = local write "旋转齿条轴使能"(TRUE ("旋转齿条轴使能")) -> ()
          }
          frame #10 {
            n239 = local read "旋转齿条电机"() -> (w455:u32)
            n240 = call "PCI1220U角度置零.vi"("AxisHandle IN"=w455) -> ()  [unwired: 10 in, 1 out]
          }
          frame #11 {
            n241 = local write "旋转伺服速度(°/s)"(1.0 ("旋转齿条轴速度(°/s)")) -> ()
            n242 = Wait (ms)(milliseconds to wait=u32 1000 ("毫秒倍数")) -> ()  [unwired: 1 out]
          }
          frame #12 {
            n243 = while {
              i -> [w463]
              stop <- w460 stop-if-true
              n244 = local read "间隙位移(mm)"() -> (w464:dbl)
              n245 = Wait Until Next ms Multiple(millisecond multiple=u32 50 ("毫秒倍数")) -> ()  [unwired: 1 out]
              n246 = Greater Or Equal?(x=w463, y=40) -> (x >= y?=w460:bool)
              n247 = local write "基准位移"(w464) -> ()
            }
          }
          frame #13 {
            n248 = call "PCI1220U运行.vi"("方向"=enum32{"Negative", "Positive"}."Negative" ("Direction"), "AxisHandle IN"=w466) -> ("AxisHandle OUT"=w465:u32)  [unwired: 9 in]
          }
          frame #14 {
            w471 = dbl[] []
            n249 = while {
              shift-right: [w482] -> w470
              shift-left: w471 -> [w484]
              shift-right: [w481] -> w469
              shift-left: w471 -> [w483]
              stop <- w474 stop-if-true
              n250 = Wait (ms)(milliseconds to wait=u32 10 ("毫秒倍数")) -> ()  [unwired: 1 out]
              n251 = local read "间隙位移(mm)"() -> (w477:dbl)
              n252 = local read "基准位移"() -> (w475:dbl)
              n253 = local read "齿条扭矩(Nm)"() -> (w478:dbl)
              n254 = Subtract(x=w477, y=w475) -> (x-y=w476:dbl)
              n255 = Absolute Value(x=w478) -> (abs(x)=w473:dbl)
              n256 = Build Array (concatenate) "创建数组"(w483, w476) -> (w481:dbl[])
              n257 = Build Array (concatenate) ("创建数组")(w484, w473) -> (w482:dbl[])
              n258 = Greater Or Equal?(x=w473, y="扭矩停止值") -> (x >= y?=w474:bool)
              n259 = Bundle ("捆绑")(w482, w481) -> (w479:cluster{dbl[], dbl[]})  [unwired: 1 in]
              n260 = Build Array ("创建数组")(w479) -> (w480:cluster{dbl[], dbl[]}[])
              n261 = local write "扭动曲线"(w480) -> ()
            }
          }
          frame #15 {
            n262 = Absolute Value(x=w494) -> (abs(x)=w495:dbl[])
            n263 = local read "测量点扭矩"() -> (w496:dbl)
            n264 = local read "基准位移"() -> (w490:dbl)
            n265 = call "自定义插值.vi"("压力"=w496, "扭矩数组"=w495, "位移数组"=w493) -> ("扭矩值"=w491:dbl)  [unwired: 8 in]
            n266 = Array Max & Min(array=w493) -> (min value=w492:dbl)  [unwired: 3 out]
            n267 = Absolute Value(x=w492) -> (abs(x)=w489:dbl)
            n268 = Subtract(x=w490, y=w489) -> (x-y=w488:dbl)
            n269 = Add(x=w491, y=w489) -> (x+y=w487:dbl)
            n270 = Absolute Value(x=w487) -> (abs(x)=w486:dbl)
            n271 = local write "基准位移"(w488) -> ()
            n272 = local write "中间位置间隙"(w486) -> ()
          }
          frame #16 {
            n273 = while {
              tunnel: w501 -> [w505]
              tunnel: [w504] -> w500
              stop <- w503 stop-if-true
              n274 = call "PCI1220U停止.vi"("AxisHandle IN"=w505) -> ("完成"=w503:bool, "AxisHandle OUT"=w504:u32)  [unwired: 9 in]
              n275 = Wait (ms)(milliseconds to wait=u32 50 ("毫秒倍数")) -> ()  [unwired: 1 out]
            }
            "间隙Y数组" <- w499
            "间隙X数组" <- w498
          }
          frame #17 {
            n276 = while {
              tunnel: [w512] -> w506
              tunnel: w507 -> [w509]
              stop <- w511 stop-if-true
              n277 = Wait Until Next ms Multiple(millisecond multiple=u32 50 ("毫秒倍数")) -> ()  [unwired: 1 out]
              n278 = call "PCI1220U扭矩轴位置模式.vi"("Distance"=0.0, "AxisHandle IN"=w509) -> ("AbsSuccess"=w511:bool, "AxisHandle OUT"=w512:u32)  [unwired: 8 in]
            }
          }
          frame #18 {
            n279 = while {
              tunnel: w514 -> [w516]
              tunnel: [w516] -> w513
              stop <- w519 stop-if-true
              n280 = local read "齿条扭矩(Nm)"() -> (w515:dbl)
              n281 = call <userlib>:"Acm_AxGetCmdVelocity.vi"("AxisHandle"=w516) -> ("Velocity"=w522:dbl)  [unwired: 1 in, 3 out]
              n282 = Wait Until Next ms Multiple(millisecond multiple=u32 50 ("毫秒倍数")) -> ()  [unwired: 1 out]
              n283 = Equal To 0?(x=w522) -> (x = 0?=w520:bool)
              n284 = Greater Or Equal?(x=w515, y=3.0) -> (x >= y?=w517:bool)
              n285 = Or(x=w520, y=w517) -> (x .or. y?=w519:bool)
            }
          }
          frame #19 {
            n286 = while {
              tunnel: w523 -> [w527]
              tunnel: [w526] -> _
              stop <- w525 stop-if-true
              n287 = call "PCI1220U停止.vi"("AxisHandle IN"=w527) -> ("完成"=w525:bool, "AxisHandle OUT"=w526:u32)  [unwired: 9 in]
              n288 = Wait (ms)(milliseconds to wait=u32 50 ("毫秒倍数")) -> ()  [unwired: 1 out]
            }
          }
          frame #20 {
            n289 = local write "旋转齿条轴使能"(FALSE ("旋转齿条轴使能")) -> ()
            n290 = Wait (ms)(milliseconds to wait=u32 500 ("毫秒倍数")) -> ()  [unwired: 1 out]
          }
          frame #21 {
            n291 = local write "工步号"(u32 25 ("工步号")) -> ()
          }
        }
      }
      frame 25 {
        n292 = flat-sequence {
          frame #0 {
            n293 = local read "中间间隙标准(mm)"() -> (w532:dbl)
            n294 = local read "中间位置间隙"() -> (w533:dbl)
            n295 = local read "最小间隙(mm)"() -> (w531:dbl)
            n296 = In Range and Coerce(upper limit=w532, x=w533, lower limit=w531) -> (In Range?=w536:bool)  [unwired: 1 out]
            n297 = case shown="假" w536 {
              tunnel: [FALSE ("本序合格") TRUE ("本序合格")] -> w535
              tunnel: [w541 0.0 ("需调整角度(度)")] -> w534
              tunnel: w533 -> [w539 _]
              tunnel: w532 -> [w538 _]
              tunnel: w531 -> [w537 _]
              frame False {
                n298 = xnode "公式"("X"=w539, "Xmax"=w538, "Xmin"=w537) -> ("结果"=w541:dbl)  [unwired: 1 in, 1 out]
              }
              frame True {
              }
            }
            n299 = local write "单点间隙合格"(w535) -> ()
            n300 = local write "需调整角度(度)"(w534) -> ()
          }
          frame #1 {
            n301 = local read "单点间隙合格"() -> (w556:bool)
            n302 = case shown="假" w556 {
              frame False {
                n303 = local read "已调试次数"() -> (w559:dbl)
                n304 = Less?(x=w559, y="设定间隙调整次数") -> (x < y?=w558:bool)
                n305 = case shown="真" w558 {
                  frame False {
                    n306 = local write "工步号"(u32 45 ("变更工步号")) -> ()
                  }
                  frame True {
                    n307 = local write "工步号"(u32 30 ("变更工步号")) -> ()
                  }
                }
              }
              frame True {
                n308 = local write "工步号"(u32 40 ("变更工步号")) -> ()
              }
            }
          }
        }
      }
      frame 30 {
        # "人工调整"
        n309 = flat-sequence {
          tunnel: [w565] -> w563
          tunnel: w563 -> [w572]
          frame #0 {
            n310 = local write "测头机构轴速度(mm/s)"(30.0 ("测头机构轴速度(mm/s)")) -> ()
          }
          frame #1 {
            n311 = local read "测头机构电机"() -> (w566:u32)
            n312 = while {
              tunnel: w566 -> [w569]
              tunnel: [w568] -> w565
              stop <- w571 stop-if-true
              n313 = local read "测头机构轴待检位"() -> (w567:dbl)
              n314 = call "PCI1220U进给轴位置模式.vi"("Distance"=w567, "AxisHandle IN"=w569) -> ("AbsSuccess"=w571:bool, "AxisHandle OUT"=w568:u32)  [unwired: 8 in]
              n315 = Wait Until Next ms Multiple(millisecond multiple=u32 50 ("毫秒倍数")) -> ()  [unwired: 1 out]
            }
          }
          frame #2 {
            n316 = while {
              tunnel: w572 -> [w576]
              stop <- w574 stop-if-true
              n317 = call <userlib>:"Acm_AxGetCmdVelocity.vi"("AxisHandle"=w576) -> ("Velocity"=w575:dbl)  [unwired: 1 in, 3 out]
              n318 = Wait Until Next ms Multiple(millisecond multiple=u32 50 ("毫秒倍数")) -> ()  [unwired: 1 out]
              n319 = Equal To 0?(x=w575) -> (x = 0?=w574:bool)
            }
          }
          frame #3 {
            n320 = while {
              stop <- w578 stop-if-true
              n321 = local read "测头机构轴位置(mm)"() -> (w580:dbl)
              n322 = Wait Until Next ms Multiple(millisecond multiple=u32 50 ("毫秒倍数")) -> ()  [unwired: 1 out]
              n323 = Less Or Equal?(x=w580, y=35.0) -> (x <= y?=w578:bool)
            }
          }
          frame #4 {
            n324 = local write "测头气缸左移"(TRUE ("测头气缸左移")) -> ()
            n325 = local write "测头气缸右移"(FALSE ("测头气缸右移")) -> ()
          }
          frame #5 {
            n326 = while {
              stop <- w583 stop-if-true
              # "等待启动"
              n327 = local read "间隙启动"() -> (w583:bool)
              n328 = Wait Until Next ms Multiple(millisecond multiple=u32 50 ("毫秒倍数")) -> ()  [unwired: 1 out]
            }
          }
          frame #6 {
            n329 = local read "不合格品"() -> (w585:bool)
            n330 = case shown="假" w585 {
              frame False {
                n331 = flat-sequence {
                  frame #0 {
                    n332 = local read "已调试次数"() -> (w588:dbl)
                    n333 = local write "测头气缸左移"(FALSE ("测头气缸左移")) -> ()
                    n334 = local write "测头气缸右移"(TRUE ("测头气缸左移")) -> ()
                    n335 = Add(x=w588, y=1.0 ("已调试次数")) -> (x+y=w590:dbl)
                    n336 = local write "已调试次数"(w590) -> ()
                  }
                  frame #1 {
                    n337 = while {
                      stop <- w591 stop-if-true
                      n338 = Wait Until Next ms Multiple(millisecond multiple=u32 50 ("毫秒倍数")) -> ()  [unwired: 1 out]
                      n339 = local read "测头右位"() -> (w591:bool)
                    }
                  }
                  frame #2 {
                    n340 = local write "工步号"(u32 20 ("工步号")) -> ()
                  }
                }
              }
              frame True {
                n341 = local write "工步号"(u32 45 ("工步号")) -> ()
              }
            }
          }
        }
      }
      frame 40 {
      }
      frame 45 {
        # "测头退回"
        n342 = flat-sequence {
          tunnel: [w598] -> w595
          tunnel: w595 -> [w605]
          frame #0 {
            n343 = local write "测头机构轴速度(mm/s)"(30.0 ("测头机构轴速度(mm/s)")) -> ()
          }
          frame #1 {
            n344 = local read "测头机构轴后退位"() -> (w597:dbl)
            n345 = local read "测头机构电机"() -> (w599:u32)
            n346 = while {
              tunnel: w599 -> [w603]
              tunnel: w597 -> [w602]
              tunnel: [w601] -> w598
              stop <- w604 stop-if-true
              n347 = Wait Until Next ms Multiple(millisecond multiple=u32 50 ("毫秒倍数")) -> ()  [unwired: 1 out]
              n348 = call "PCI1220U进给轴位置模式.vi"("Distance"=w602, "AxisHandle IN"=w603) -> ("AbsSuccess"=w604:bool, "AxisHandle OUT"=w601:u32)  [unwired: 8 in]
            }
          }
          frame #2 {
            n349 = while {
              tunnel: w605 -> [w609]
              stop <- w607 stop-if-true
              n350 = call <userlib>:"Acm_AxGetCmdVelocity.vi"("AxisHandle"=w609) -> ("Velocity"=w608:dbl)  [unwired: 1 in, 3 out]
              n351 = Wait Until Next ms Multiple(millisecond multiple=u32 50 ("毫秒倍数")) -> ()  [unwired: 1 out]
              n352 = Equal To 0?(x=w608) -> (x = 0?=w607:bool)
            }
          }
          frame #3 {
            n353 = while {
              stop <- w610 stop-if-true
              n354 = local read "测头机构轴位置(mm)"() -> (w612:dbl)
              n355 = Wait Until Next ms Multiple(millisecond multiple=u32 50 ("毫秒倍数")) -> ()  [unwired: 1 out]
              n356 = Less Or Equal?(x=w612, y=35.0) -> (x <= y?=w610:bool)
            }
          }
          frame #4 {
            n357 = local write "测头气缸左移"(TRUE ("测头气缸左移")) -> ()
            n358 = local write "测头气缸右移"(FALSE ("测头气缸右移")) -> ()
          }
          frame #5 {
            n359 = Wait Until Next ms Multiple(millisecond multiple=u32 500 ("毫秒倍数")) -> ()  [unwired: 1 out]
          }
          frame #6 {
            n360 = local write "工步号"(u32 50 ("工步号")) -> ()
          }
        }
      }
      frame 50 {
        n361 = flat-sequence {
          tunnel: [w639] -> w628
          tunnel: w628 -> [w646]
          tunnel: [w645] -> w626
          tunnel: w626 -> [w657]
          tunnel: [w664] -> w620
          tunnel: [w668] -> w621
          tunnel: w620 -> [w668]
          tunnel: [w671] -> w623
          tunnel: w621 -> [w670]
          tunnel: w623 -> [w678]
          tunnel: [w677] -> w622
          tunnel: w622 -> [w680]
          tunnel: [w679] -> w618
          tunnel: [w685] -> w619
          tunnel: w618 -> [w685]
          tunnel: [w688] -> w627
          tunnel: w619 -> [w687]
          tunnel: w627 -> [w694]
          tunnel: [w695] -> w625
          tunnel: w625 -> [w704]
          tunnel: [w703] -> w624
          tunnel: w624 -> [w714]
          frame #0 {
            n362 = local write "旋转伺服速度(°/s)"(15.0 ("调整螺塞轴速度(°/s)")) -> ()
            n363 = local write "测头机构轴速度(mm/s)"(15.0 ("调整机构轴速度(mm/s)")) -> ()
            n364 = local write "电动缸速度(mm/s)"(15.0 ("电动缸速度(mm/s)")) -> ()
            n365 = local write "夹头松开"(TRUE ("夹头松开")) -> ()
            n366 = local write "夹头夹紧"(FALSE ("夹头夹紧")) -> ()
          }
          frame #1 {
            n367 = while {
              stop <- w634 stop-if-true
              n368 = local read "夹头夹紧位"() -> (w637:bool)
              n369 = local read "夹头松开"() -> (w635:bool)
              n370 = Wait Until Next ms Multiple(millisecond multiple=u32 50 ("毫秒倍数")) -> ()  [unwired: 1 out]
              n371 = Not(x=w637) -> (.not. x?=w636:bool)
              n372 = And(x=w636, y=w635) -> (x .and. y?=w634:bool)
            }
          }
          frame #2 {
            n373 = while {
              tunnel: [w642] -> w639
              stop <- w641 stop-if-true
              n374 = local read "电动缸电机"() -> (w643:u32)
              n375 = Wait Until Next ms Multiple(millisecond multiple=u32 50 ("毫秒倍数")) -> ()  [unwired: 1 out]
              n376 = local read "齿条右极限"() -> (w640:dbl)
              n377 = call "PCI1240电动缸位置模式 .vi"("Distance"=w640, "AxisHandle IN"=w643) -> ("AbsSuccess"=w641:bool, "AxisHandle OUT"=w642:u32)  [unwired: 8 in]
            }
          }
          frame #3 {
            n378 = while {
              tunnel: w646 -> [w655]
              tunnel: [w647] -> w645
              stop <- w648 stop-if-true
              n379 = local read "齿条推拉力(N)"() -> (w653:dbl)
              n380 = Wait Until Next ms Multiple(millisecond multiple=u32 50 ("毫秒倍数")) -> ()  [unwired: 1 out]
              n381 = call <userlib>:"Acm_AxGetCmdVelocity.vi"("AxisHandle"=w655) -> ("Velocity"=w656:dbl, "AxisHandle"=w647:u32)  [unwired: 1 in, 2 out]
              n382 = Equal To 0?(x=w656) -> (x = 0?=w650:bool)
              n383 = Absolute Value(x=w653) -> (abs(x)=w652:dbl)
              n384 = Greater Or Equal?(x=w652, y=1000.0) -> (x >= y?=w649:bool)
              n385 = Or(x=w650, y=w649) -> (x .or. y?=w648:bool)
            }
          }
          frame #4 {
            n386 = while {
              tunnel: w657 -> [w661]
              tunnel: [w660] -> _
              stop <- w659 stop-if-true
              n387 = call "PCI1220U停止.vi"("AxisHandle IN"=w661) -> ("完成"=w659:bool, "AxisHandle OUT"=w660:u32)  [unwired: 9 in]
              n388 = Wait (ms)(milliseconds to wait=u32 50 ("毫秒倍数")) -> ()  [unwired: 1 out]
            }
          }
          frame #5 {
            n389 = local write "旋转齿条轴使能"(TRUE ("旋转齿条轴使能")) -> ()
          }
          frame #6 {
            n390 = Wait Until Next ms Multiple(millisecond multiple=u32 500 ("毫秒倍数")) -> ()  [unwired: 1 out]
          }
          frame #7 {
            n391 = local read "旋转齿条电机"() -> (w665:u32)
            n392 = call <userlib>:"Acm_AxHome.vi"("DirMode"=u32 0, "HomeMode"=u32 11, "AxisHandle"=w665) -> ("AxisHandle"=w664:u32)  [unwired: 1 in, 2 out]
          }
          frame #8 {
            n393 = Wait Until Next ms Multiple(millisecond multiple=u32 100 ("毫秒倍数")) -> ()  [unwired: 1 out]
          }
          frame #9 {
            n394 = while {
              tunnel: w670 -> [w674]
              tunnel: [w673] -> w671
              stop <- w672 stop-if-true
              n395 = call <userlib>:"Acm_AxGetCmdVelocity.vi"("AxisHandle"=w674) -> ("Velocity"=w676:dbl, "AxisHandle"=w673:u32)  [unwired: 1 in, 2 out]
              n396 = Equal To 0?(x=w676) -> (x = 0?=w672:bool)
              n397 = Wait Until Next ms Multiple(millisecond multiple=u32 50 ("毫秒倍数")) -> ()  [unwired: 1 out]
            }
          }
          frame #10 {
            n398 = call "PCI1220U角度置零.vi"("AxisHandle IN"=w678) -> ("AxisHandle OUT"=w677:u32)  [unwired: 10 in]
          }
          frame #11 {
            n399 = while {
              tunnel: [w681] -> w679
              tunnel: w680 -> [w681]
              stop <- w684 stop-if-true
              n400 = Wait Until Next ms Multiple(millisecond multiple=u32 50 ("毫秒倍数")) -> ()  [unwired: 1 out]
              n401 = call "PCI1220U扭矩轴位置模式.vi"("Distance"=15.0, "AxisHandle IN"=w681) -> ("AbsSuccess"=w684:bool)  [unwired: 8 in, 1 out]
            }
          }
          frame #12 {
            n402 = Wait Until Next ms Multiple(millisecond multiple=u32 100 ("毫秒倍数")) -> ()  [unwired: 1 out]
          }
          frame #13 {
            n403 = while {
              tunnel: w687 -> [w691]
              tunnel: [w690] -> w688
              stop <- w689 stop-if-true
              n404 = call <userlib>:"Acm_AxGetCmdVelocity.vi"("AxisHandle"=w691) -> ("Velocity"=w693:dbl, "AxisHandle"=w690:u32)  [unwired: 1 in, 2 out]
              n405 = Equal To 0?(x=w693) -> (x = 0?=w689:bool)
              n406 = Wait Until Next ms Multiple(millisecond multiple=u32 50 ("毫秒倍数")) -> ()  [unwired: 1 out]
            }
          }
          frame #14 {
            n407 = call "PCI1220U角度置零.vi"("AxisHandle IN"=w694) -> ()  [unwired: 10 in, 1 out]
          }
          frame #15 {
            n408 = while {
              tunnel: [w700] -> w695
              stop <- w699 stop-if-true
              n409 = local read "电动缸电机"() -> (w701:u32)
              n410 = Wait Until Next ms Multiple(millisecond multiple=u32 50 ("毫秒倍数")) -> ()  [unwired: 1 out]
              n411 = local read "齿条右极限"() -> (w698:dbl)
              n412 = Add(x=w698, y=-10.0) -> (x+y=w696:dbl)
              n413 = call "PCI1240电动缸位置模式 .vi"("Distance"=w696, "AxisHandle IN"=w701) -> ("AbsSuccess"=w699:bool, "AxisHandle OUT"=w700:u32)  [unwired: 8 in]
            }
          }
          frame #16 {
            n414 = while {
              tunnel: w704 -> [w712]
              tunnel: [w710] -> w703
              stop <- w705 stop-if-true
              n415 = local read "齿条推拉力(N)"() -> (w709:dbl)
              n416 = Wait Until Next ms Multiple(millisecond multiple=u32 50 ("毫秒倍数")) -> ()  [unwired: 1 out]
              n417 = call <userlib>:"Acm_AxGetCmdVelocity.vi"("AxisHandle"=w712) -> ("Velocity"=w713:dbl, "AxisHandle"=w710:u32)  [unwired: 1 in, 2 out]
              n418 = Equal To 0?(x=w713) -> (x = 0?=w706:bool)
              n419 = Greater Or Equal?(x=w709, y=300.0) -> (x >= y?=w707:bool)
              n420 = Or(x=w706, y=w707) -> (x .or. y?=w705:bool)
            }
          }
          frame #17 {
            n421 = while {
              tunnel: w714 -> [w718]
              tunnel: [w717] -> _
              stop <- w716 stop-if-true
              n422 = call "PCI1220U停止.vi"("AxisHandle IN"=w718) -> ("完成"=w716:bool, "AxisHandle OUT"=w717:u32)  [unwired: 9 in]
              n423 = Wait (ms)(milliseconds to wait=u32 50 ("毫秒倍数")) -> ()  [unwired: 1 out]
            }
          }
          frame #18 {
            n424 = local write "工步号"(u32 100 ("工步号")) -> ()
          }
        }
      }
      frame 100 {
        n425 = flat-sequence {
          tunnel: [w753] -> w743
          tunnel: [w751] -> w742
          tunnel: [w745] -> w729
          tunnel: [w744] -> w727
          tunnel: w743 -> [w760]
          tunnel: w742 -> [w757]
          tunnel: ["F:\\报表存储\\" ("字符串")] -> w741
          tunnel: [w760] -> w730
          tunnel: w729 -> [w759]
          tunnel: [w759] -> w728
          tunnel: w727 -> [w758]
          tunnel: [w758] -> w726
          tunnel: [w757] -> w725
          tunnel: w741 -> [w771]
          tunnel: [w779] -> w740
          tunnel: [w776] -> w739
          tunnel: [w775] -> w738
          tunnel: [w774] -> w737
          tunnel: w730 -> [w770]
          tunnel: w728 -> [w769]
          tunnel: w726 -> [w768]
          tunnel: w725 -> [w762]
          tunnel: [w764] -> w724
          tunnel: w740 -> [w786]
          tunnel: [w787] -> w736
          tunnel: w739 -> [w787]
          tunnel: w738 -> [w785]
          tunnel: w737 -> [w784]
          tunnel: [w783] -> w735
          tunnel: [w782] -> w734
          tunnel: w724 -> [w781]
          tunnel: [w781] -> w723
          tunnel: [w794] -> w733
          tunnel: w736 -> [w794]
          tunnel: w735 -> [w793]
          tunnel: [w793] -> w732
          tunnel: [w792] -> w731
          tunnel: w734 -> [w792]
          tunnel: w723 -> [w790]
          tunnel: [w790] -> w722
          tunnel: w733 -> [w797]
          tunnel: w732 -> [w805]
          tunnel: w731 -> [w804]
          tunnel: w722 -> [w796]
          tunnel: [w796] -> w721
          tunnel: w721 -> [w813]
          tunnel: [w813] -> w720
          tunnel: w720 -> [w815]
          frame #0 {
            n426 = local read "产品ID"() -> (w752:string)
            n427 = Format Date/Time String(time format string (%c)="%Y%m%d" ("时间格式字符串(%c)")) -> (date/time string=w746:string)  [unwired: 2 in]
            n428 = String Subset(string=w746, offset (0)=4 ("偏移量(0)"), length (rest)=2 ("长度（剩余）")) -> (substring=w745:string)
            n429 = String Subset(string=w746, offset (0)=6 ("偏移量(0)"), length (rest)=2 ("长度（剩余）")) -> (substring=w744:string)
            n430 = call <vilib>:"Trim Whitespace.vi"("string"=w752) -> ("trimmed string"=w751:string)  [unwired: 1 in]
            n431 = String Subset(string=w746, offset (0)=0 ("偏移量(0)"), length (rest)=4 ("长度（剩余）")) -> (substring=w753:string)
          }
          frame #1 {
          }
          frame #2 {
            w763 = "\\" ("字符串")
            n432 = Concatenate Strings(w771, w770, w763, w769, w763, w768, w763, w762, w763) -> (w766:string)
            n433 = Concatenate Strings(w771, w770, w763, w769, w763, w768, w763, w762, w763) -> (w780:string)
            n434 = String To Path(string=w780) -> (path=w779:path)
            n435 = Concatenate Strings(w766, w762, "间隙曲线.JPG" ("字符串")) -> (w777:string)
            n436 = Concatenate Strings(w766, "轴向力曲线数组.txt" ("字符串")) -> (w774:string)
            n437 = Concatenate Strings(w766, "扭动曲线数组.txt" ("字符串")) -> (w775:string)
            n438 = Concatenate Strings(w766, w762, "轴向力曲线.JPG" ("字符串")) -> (w767:string)
            n439 = String To Path(string=w777) -> (path=w776:path)
            n440 = String To Path(string=w767) -> (path=w764:path)
          }
          frame #3 {
            n441 = call <vilib>:"Check if File or Folder Exists.vi"("path"=w786) -> ("file or folder exists?"=w788:bool)  [unwired: 8 in, 2 out]
            n442 = String To Path(string=w784) -> (path=w782:path)
            n443 = String To Path(string=w785) -> (path=w783:path)
            n444 = case shown="假" w788 {
              tunnel: w786 -> [w789 _]
              frame False {
                n445 = Create Folder(path (use dialog)=w789) -> ()  [unwired: 2 in, 3 out]
              }
              frame True {
              }
            }
          }
          frame #4 {
            n446 = local write "选项卡控件"(T1."间隙测量" ("选项卡控件")) -> ()
            n447 = Wait Until Next ms Multiple(millisecond multiple=u32 1000 ("毫秒倍数")) -> ()  [unwired: 1 out]
          }
          frame #5 {
            n448 = disable-structure shown="禁用" {
              disable-tunnel: w797 -> [w806 _]
              frame Disabled {
                w810 = T2 2 items=["快速打印", "标准报表", "HTML", "双字节", "Excel"] ("report type (Quick Print)")
                w809 = T3 1 items=["完整前面板", "前面板可见部分", "图标、说明、前面板和程序框图", "说明信息: 使用前面板", "说明信息: 作为子VI使用", "说明信息: 完整", "说明信息: 自定义"] ("contents (complete front panel)")
                n449 = Current VI's Path() -> (path=w808:path)
                n450 = call-poly <vilib>:"Easy Print VI Panel or Documentation.vi"("report type (Quick Print)"=w810, "contents (complete front panel)"=w809, "VI path"=w808) -> ("error out"=w812:errorcluster, "report out"=w811:refnum<class "NI_report.lvclass">)  [unwired: 1 in, 6 out]
                n451 = call-dynamic "Save Report to File.vi"("report in"=w811, "report file path"=w806, "error in (no error)"=w812) -> ("error out"=→"error out 3":errorcluster)  [unwired: 2 in, 10 out]
              }
              frame Enabled {
              }
            }
            n452 = local read "间隙Y数组"() -> (w802:dbl[])
            n453 = local read "间隙X数组"() -> (w803:dbl[])
            n454 = local read "轴向力Y"() -> (w800:dbl[])
            n455 = local read "轴向力X"() -> (w801:dbl[])
            n456 = call "导出曲线数组.vi"("file path (dialog if empty)"=w805, "数组 2"=w802, "数组"=w803) -> ()  [unwired: 9 in]
            n457 = call "导出曲线数组.vi"("file path (dialog if empty)"=w804, "数组 2"=w800, "数组"=w801) -> ()  [unwired: 9 in]
            n458 = control-ref of="本VI"() -> (w799:refnum<vi>)
            n459 = invoke class="VI" method="FP.Get Image"(reference=w799) -> ("image data"=w798:T4)  [unwired: 5 in, 5 out]
            n460 = call <vilib>:"Write JPEG File.vi"("image data"=w798, "path to JPEG file"=w797) -> ()  [unwired: 8 in, 2 out]
          }
          frame #6 {
            n461 = local write "选项卡控件"(T1."轴向力测量" ("选项卡控件")) -> ()
          }
          frame #7 {
            n462 = control-ref of="本VI"() -> (w816:refnum<vi>)
            n463 = invoke class="VI" method="FP.Get Image"(reference=w816) -> ("image data"=w817:T4)  [unwired: 5 in, 5 out]
            n464 = call <vilib>:"Write JPEG File.vi"("image data"=w817, "path to JPEG file"=w815) -> ()  [unwired: 8 in, 2 out]
          }
          frame #8 {
            n465 = local read "联线按钮"() -> (w818:bool)
            n466 = case shown="真" w818 {
              frame False {
              }
              frame True {
                n467 = flat-sequence {
                  tunnel: [w845] -> w819
                  tunnel: w819 -> [w860]
                  frame #0 {
                    w838 = i16 3 ("精度(6)")
                    n468 = local read "全行程间隙及轴向力合格"() -> (w840:bool)
                    n469 = local read "左180°外全行程间隙"() -> (w837:dbl)
                    n470 = local read "右180°内全行程间隙"() -> (w839:dbl)
                    n471 = local read "右180°外全行程间隙"() -> (w836:dbl)
                    n472 = local read "左最大轴向力(N)"() -> (w835:dbl)
                    n473 = local read "右最大轴向力(N)"() -> (w834:dbl)
                    n474 = local read "左轴向力波动(N)"() -> (w833:dbl)
                    n475 = local read "单点间隙合格"() -> (w841:bool)
                    n476 = local read "左180°内全行程间隙"() -> (w848:dbl)
                    n477 = local read "右轴向力波动(N)"() -> (w832:dbl)
                    n478 = local read "总行程(mm)"() -> (w831:dbl)
                    n479 = local read "总圈数"() -> (w830:dbl)
                    n480 = local read "员工ID"() -> (w820:string)
                    n481 = local read "中间位置间隙"() -> (w850:dbl)
                    n482 = local read "FGCS"() -> (w852:string)
                    n483 = And(x=w841, y=w840) -> (x .and. y?=w842:bool)
                    n484 = local read "KSJJ"() -> (w854:string)
                    n485 = local read "产品ID"() -> (w857:string)
                    n486 = Boolean To (0,1)(Boolean=w842) -> (0, 1=w856:i16)
                    n487 = Number To Fractional String(number=w831, precision (6)=w838) -> (F-format string=w822:string)  [unwired: 2 in]
                    n488 = Number To Fractional String(number=w833, precision (6)=w838) -> (F-format string=w824:string)  [unwired: 2 in]
                    n489 = Number To Fractional String(number=w832, precision (6)=w838) -> (F-format string=w823:string)  [unwired: 2 in]
                    n490 = Number To Fractional String(number=w839, precision (6)=w838) -> (F-format string=w829:string)  [unwired: 2 in]
                    n491 = Number To Fractional String(number=w837, precision (6)=w838) -> (F-format string=w828:string)  [unwired: 2 in]
                    n492 = Number To Fractional String(number=w830, precision (6)=w838) -> (F-format string=w821:string)  [unwired: 2 in]
                    n493 = Number To Fractional String(number=w848, precision (6)=w838) -> (F-format string=w846:string)  [unwired: 2 in]
                    n494 = Number To Fractional String(number=w834, precision (6)=w838) -> (F-format string=w825:string)  [unwired: 2 in]
                    n495 = Number To Fractional String(number=w836, precision (6)=w838) -> (F-format string=w827:string)  [unwired: 2 in]
                    n496 = Number To Fractional String(number=w835, precision (6)=w838) -> (F-format string=w826:string)  [unwired: 2 in]
                    n497 = Number To Fractional String(number=w850, precision (6)=i16 3 ("精度(6)")) -> (F-format string=w847:string)  [unwired: 2 in]
                    n498 = Format Date/Time String(time format string (%c)="%Y%m%d%H%M" ("时间格式字符串(%c)")) -> (date/time string=w853:string)  [unwired: 2 in]
                    n499 = Number To Decimal String(number=w856, width (-)=i16 1 ("宽度(-)")) -> (decimal integer string=w843:string)
                    n500 = Build Array(w857, w820, "1", w843, w854, w853, w852, "Q14070-Z060A", w847, w846, w829, w828, w827, w826, w825, w824, w823, w822, w821) -> (w845:string[])
                  }
                  frame #1 {
                    n501 = Wait (ms)(milliseconds to wait=u32 500 ("等待时间（毫秒）")) -> ()  [unwired: 1 out]
                    n502 = call "数据库更新.vi"("设备号"="06", "数据"=w860) -> ()  [unwired: 13 in, 1 out]
                  }
                  frame #2 {
                  }
                }
              }
            }
          }
          frame #9 {
            n503 = local write "产品ID"("") -> ()
            n504 = local write "工步号"(u32 0 ("工步号")) -> ()
          }
        }
      }
    }
    n505 = Wait (ms)(milliseconds to wait=u32 50 ("毫秒倍数")) -> ()  [unwired: 1 out]
    n506 = local read "停止"() -> (w133:bool)
  }
  n507 = flat-sequence {
    tunnel: [w867] -> w126
    tunnel: w126 -> [w869]
    tunnel: [w868] -> w125
    tunnel: w125 -> [w877]
    tunnel: [w877] -> w124
    tunnel: w124 -> [w889]
    tunnel: [w889] -> w123
    tunnel: w123 -> [w890]
    tunnel: [w891] -> w122
    tunnel: w122 -> [w899]
    tunnel: [w899] -> w121
    tunnel: w121 -> [w909]
    tunnel: [w909] -> w120
    tunnel: w120 -> [w917]
    tunnel: [w917] -> w119
    tunnel: w119 -> [w919]
    tunnel: [w920] -> w118
    tunnel: [w918] -> w117
    tunnel: w118 -> [w931]
    tunnel: w117 -> [w932]
    tunnel: [w932] -> w116
    tunnel: [w930] -> w115
    tunnel: [w929] -> w114
    tunnel: [w928] -> w113
    tunnel: w116 -> [w971]
    tunnel: [w971] -> w112
    tunnel: [w970] -> w111
    tunnel: w115 -> [w970]
    tunnel: [w969] -> w110
    tunnel: w114 -> [w969]
    tunnel: [w968] -> w109
    tunnel: w113 -> [w968]
    tunnel: w112 -> [w973]
    tunnel: [w972] -> w108
    tunnel: [w976] -> w107
    tunnel: w111 -> [w976]
    tunnel: [w975] -> w106
    tunnel: w110 -> [w975]
    tunnel: [w974] -> w105
    tunnel: w109 -> [w974]
    tunnel: [w991] -> w8
    tunnel: [w990] -> w7
    tunnel: [w989] -> w5
    tunnel: w108 -> [w984]
    tunnel: w107 -> [w988]
    tunnel: w106 -> [w987]
    tunnel: w105 -> [w986]
    tunnel: [w984] -> w6
    tunnel: [w1044] -> w104
    tunnel: [w1028] -> w103
    tunnel: [w1026] -> w102
    tunnel: [w1042] -> w101
    tunnel: [w1041] -> w100
    tunnel: [w1040] -> w99
    tunnel: [w1039] -> w98
    tunnel: [w1032] -> w97
    tunnel: [w1031] -> w96
    tunnel: w5 -> [w1042]
    tunnel: w6 -> [w1043]
    tunnel: w7 -> [w1028]
    tunnel: w8 -> [w1044]
    tunnel: w104 -> [w1067]
    tunnel: [w1067] -> w95
    tunnel: w103 -> [w1066]
    tunnel: [w1066] -> w94
    tunnel: w102 -> [w1065]
    tunnel: [w1065] -> w93
    tunnel: [w1051] -> w92
    tunnel: [w1064] -> w91
    tunnel: w101 -> [w1064]
    tunnel: w100 -> [w1061]
    tunnel: w99 -> [w1063]
    tunnel: w98 -> [w1062]
    tunnel: [w1055] -> w90
    tunnel: [w1054] -> w89
    tunnel: w97 -> [w1053]
    tunnel: [w1053] -> w88
    tunnel: [w1052] -> w87
    tunnel: w96 -> [w1052]
    tunnel: w95 -> [w1083]
    tunnel: w94 -> [w1082]
    tunnel: w93 -> [w1074]
    tunnel: w92 -> [w1078]
    tunnel: w91 -> [w1081]
    tunnel: w90 -> [w1085]
    tunnel: [w1085] -> w86
    tunnel: w89 -> [w1084]
    tunnel: [w1084] -> w85
    tunnel: [w1080] -> w84
    tunnel: [w1079] -> w83
    tunnel: [w1077] -> w82
    tunnel: w88 -> [w1076]
    tunnel: [w1076] -> w81
    tunnel: [w1075] -> w80
    tunnel: w87 -> [w1075]
    tunnel: [w1074] -> w2
    tunnel: w86 -> [w1129]
    tunnel: [w1129] -> w79
    tunnel: w85 -> [w1128]
    tunnel: [w1128] -> w78
    tunnel: [w1122] -> w77
    tunnel: [w1127] -> w76
    tunnel: w84 -> [w1127]
    tunnel: [w1126] -> w75
    tunnel: w83 -> [w1126]
    tunnel: [w1125] -> w74
    tunnel: w82 -> [w1125]
    tunnel: w81 -> [w1124]
    tunnel: [w1124] -> w73
    tunnel: [w1123] -> w72
    tunnel: w80 -> [w1123]
    tunnel: w2 -> [w1122]
    tunnel: w79 -> [w1138]
    tunnel: [w1138] -> w71
    tunnel: w78 -> [w1137]
    tunnel: [w1137] -> w70
    tunnel: w77 -> [w1130]
    tunnel: [w1136] -> w69
    tunnel: w76 -> [w1136]
    tunnel: [w1135] -> w68
    tunnel: w75 -> [w1135]
    tunnel: [w1130] -> w67
    tunnel: [w1131] -> w66
    tunnel: [w1134] -> w65
    tunnel: w74 -> [w1134]
    tunnel: w73 -> [w1133]
    tunnel: [w1133] -> w64
    tunnel: [w1132] -> w63
    tunnel: w72 -> [w1132]
    tunnel: [w1156] -> w62
    tunnel: [w1155] -> w61
    tunnel: [w1154] -> w60
    tunnel: w71 -> [w1153]
    tunnel: w70 -> [w1152]
    tunnel: [w1153] -> w59
    tunnel: [w1152] -> w58
    tunnel: w69 -> [w1151]
    tunnel: w68 -> [w1150]
    tunnel: w67 -> [w1145]
    tunnel: w66 -> [w1149]
    tunnel: w65 -> [w1148]
    tunnel: w64 -> [w1147]
    tunnel: [w1147] -> w57
    tunnel: [w1146] -> w56
    tunnel: w63 -> [w1146]
    tunnel: [w1145] -> w1
    tunnel: w62 -> [w1198]
    tunnel: w61 -> [w1204]
    tunnel: [w1204] -> w55
    tunnel: [w1192] -> w54
    tunnel: w60 -> [w1203]
    tunnel: [w1203] -> w53
    tunnel: [w1200] -> w52
    tunnel: [w1199] -> w51
    tunnel: [w1198] -> w50
    tunnel: w59 -> [w1197]
    tunnel: w58 -> [w1196]
    tunnel: [w1197] -> w49
    tunnel: [w1196] -> w48
    tunnel: w57 -> [w1195]
    tunnel: [w1195] -> w47
    tunnel: [w1194] -> w46
    tunnel: w56 -> [w1194]
    tunnel: [w1193] -> w3
    tunnel: w1 -> [w1192]
    tunnel: w55 -> [w1213]
    tunnel: [w1256] -> w45
    tunnel: w54 -> [w1256]
    tunnel: w53 -> [w1255]
    tunnel: [w1254] -> w44
    tunnel: w52 -> [w1253]
    tunnel: w51 -> [w1252]
    tunnel: w50 -> [w1236]
    tunnel: [w1244] -> w43
    tunnel: [w1243] -> w42
    tunnel: [w1242] -> w41
    tunnel: w49 -> [w1242]
    tunnel: [w1241] -> w40
    tunnel: w48 -> [w1241]
    tunnel: [w1240] -> w39
    tunnel: [w1239] -> w38
    tunnel: [w1223] -> w37
    tunnel: [w1224] -> w36
    tunnel: [w1222] -> w35
    tunnel: [w1221] -> w34
    tunnel: w47 -> [w1219]
    tunnel: [w1219] -> w33
    tunnel: [w1218] -> w32
    tunnel: w46 -> [w1218]
    tunnel: [w1212] -> w4
    tunnel: w3 -> [w1211]
    tunnel: w45 -> [w1281]
    tunnel: [w1281] -> w31
    tunnel: [w1278] -> w30
    tunnel: w44 -> [w1280]
    tunnel: [w1277] -> w29
    tunnel: w43 -> [w1276]
    tunnel: [w1265] -> w28
    tunnel: [w1274] -> w27
    tunnel: w42 -> [w1273]
    tunnel: [w1269] -> w26
    tunnel: w41 -> [w1269]
    tunnel: [w1268] -> w25
    tunnel: w40 -> [w1268]
    tunnel: [w1267] -> w24
    tunnel: w39 -> [w1267]
    tunnel: [w1266] -> w23
    tunnel: w38 -> [w1266]
    tunnel: [w1264] -> w22
    tunnel: w37 -> [w1264]
    tunnel: [w1263] -> w21
    tunnel: w36 -> [w1263]
    tunnel: w35 -> [w1262]
    tunnel: [w1262] -> w20
    tunnel: w34 -> [w1261]
    tunnel: [w1261] -> w19
    tunnel: w33 -> [w1260]
    tunnel: [w1260] -> w18
    tunnel: [w1259] -> w17
    tunnel: w32 -> [w1259]
    tunnel: w4 -> [w1258]
    tunnel: w31 -> [w1298]
    tunnel: [w1298] -> w16
    tunnel: w30 -> [w1297]
    tunnel: [w1297] -> w15
    tunnel: w29 -> [w1296]
    tunnel: [w1296] -> w14
    tunnel: w28 -> [w1292]
    tunnel: w27 -> [w1288]
    tunnel: w26 -> [w1291]
    tunnel: w25 -> [w1290]
    tunnel: w24 -> [w1294]
    tunnel: w23 -> [w1293]
    tunnel: w22 -> [w1287]
    tunnel: w21 -> [w1286]
    tunnel: w20 -> [w1285]
    tunnel: w19 -> [w1284]
    tunnel: w18 -> [w1283]
    tunnel: w17 -> [w1282]
    tunnel: w16 -> [w1302]
    tunnel: [w1301] -> w13
    tunnel: w15 -> [w1300]
    tunnel: [w1299] -> w12
    tunnel: w14 -> [w1299]
    tunnel: w13 -> [w1309]
    tunnel: [w1309] -> w11
    tunnel: [w1308] -> w10
    tunnel: w12 -> [w1308]
    tunnel: w11 -> [w1316]
    tunnel: [w1315] -> w9
    tunnel: w10 -> [w1314]
    tunnel: w9 -> [w1322]
    frame #0 {
      n508 = local write "电动缸速度(mm/s)"("电动缸快速") -> ()
      n509 = local write "已调试次数"(0.0 ("已调试次数")) -> ()
      n510 = local write "选项卡控件"(T1."轴向力测量" ("选项卡控件")) -> ()
      n511 = local read "电动缸电机"() -> (w867:u32)
    }
    frame #1 {
      n512 = while {
        tunnel: [w870] -> _
        tunnel: [w876] -> w868
        tunnel: w869 -> [w870]
        stop <- w871 stop-if-true
        n513 = local read "齿条左极限"() -> (w874:dbl)
        n514 = Wait (ms)(milliseconds to wait=u32 50 ("毫秒倍数")) -> ()  [unwired: 1 out]
        n515 = local read "循环退出"() -> (w873:bool)
        n516 = call "PCI1240电动缸位置模式 .vi"("Distance"=w874, "AxisHandle IN"=w870) -> ("AbsSuccess"=w872:bool, "AxisHandle OUT"=w876:u32)  [unwired: 8 in]
        n517 = Compound Arithmetic op=OR(w872, w873) -> (w871:bool)
      }
    }
    frame #2 {
      n518 = while {
        tunnel: w877 -> [w886]
        stop <- w879 stop-if-true
        n519 = local read "齿条推拉力(N)"() -> (w883:dbl)
        n520 = Wait (ms)(milliseconds to wait=u32 50 ("毫秒倍数")) -> ()  [unwired: 1 out]
        n521 = call <userlib>:"Acm_AxGetCmdVelocity.vi"("AxisHandle"=w886) -> ("Velocity"=w885:dbl)  [unwired: 1 in, 3 out]
        n522 = local read "循环退出"() -> (w878:bool)
        n523 = Less Or Equal?(x=w883, y=-500.0) -> (x <= y?=w880:bool)
        n524 = Equal To 0?(x=w885) -> (x = 0?=w881:bool)
        n525 = Compound Arithmetic op=OR(w881, w880, w878) -> (w879:bool)
      }
    }
    frame #3 {
      n526 = local read "电动缸慢速"() -> (w887:dbl)
      n527 = local write "电动缸速度(mm/s)"(w887) -> ()
      n528 = Wait (ms)(milliseconds to wait=100 ("毫秒倍数")) -> ()  [unwired: 1 out]
    }
    frame #4 {
      n529 = while {
        tunnel: [w898] -> w891
        tunnel: w890 -> [w897]
        stop <- w892 stop-if-true
        n530 = Wait (ms)(milliseconds to wait=u32 50 ("毫秒倍数")) -> ()  [unwired: 1 out]
        n531 = local read "循环退出"() -> (w894:bool)
        n532 = call "PCI1240电动缸位置模式 .vi"("Distance"=118.0, "AxisHandle IN"=w897) -> ("AbsSuccess"=w893:bool, "AxisHandle OUT"=w898:u32)  [unwired: 8 in]
        n533 = Compound Arithmetic op=OR(w893, w894) -> (w892:bool)
      }
    }
    frame #5 {
      n534 = while {
        tunnel: w899 -> [w908]
        stop <- w901 stop-if-true
        n535 = local read "齿条推拉力(N)"() -> (w905:dbl)
        n536 = Wait (ms)(milliseconds to wait=u32 50 ("毫秒倍数")) -> ()  [unwired: 1 out]
        n537 = call <userlib>:"Acm_AxGetCmdVelocity.vi"("AxisHandle"=w908) -> ("Velocity"=w907:dbl)  [unwired: 1 in, 3 out]
        n538 = local read "循环退出"() -> (w900:bool)
        n539 = Less Or Equal?(x=w905, y=-500.0) -> (x <= y?=w902:bool)
        n540 = Equal To 0?(x=w907) -> (x = 0?=w903:bool)
        n541 = Compound Arithmetic op=OR(w903, w902, w900) -> (w901:bool)
      }
    }
    frame #6 {
      n542 = while {
        tunnel: w909 -> [w914]
        stop <- w910 stop-if-true
        n543 = call "PCI1220U停止.vi"("AxisHandle IN"=w914) -> ("完成"=w911:bool)  [unwired: 9 in, 1 out]
        n544 = local read "循环退出"() -> (w912:bool)
        n545 = Wait (ms)(milliseconds to wait=u32 50 ("毫秒倍数")) -> ()  [unwired: 1 out]
        n546 = Compound Arithmetic op=OR(w911, w912) -> (w910:bool)
      }
    }
    frame #7 {
      n547 = local read "电动缸快速"() -> (w915:dbl)
      n548 = Wait (ms)(milliseconds to wait=u32 100 ("毫秒倍数")) -> ()  [unwired: 1 out]
      n549 = local write "电动缸速度(mm/s)"(w915) -> ()
    }
    frame #8 {
      n550 = while {
        tunnel: w919 -> [w927]
        tunnel: [w925] -> w918
        stop <- w921 stop-if-true
        n551 = local read "齿条右极限"() -> (w924:dbl)
        n552 = Wait (ms)(milliseconds to wait=u32 50 ("毫秒倍数")) -> ()  [unwired: 1 out]
        n553 = local read "循环退出"() -> (w923:bool)
        n554 = call "PCI1240电动缸位置模式 .vi"("Distance"=w924, "AxisHandle IN"=w927) -> ("AbsSuccess"=w922:bool, "AxisHandle OUT"=w925:u32)  [unwired: 8 in]
        n555 = Compound Arithmetic op=OR(w922, w923) -> (w921:bool)
      }
      n556 = local read "转向器中心"() -> (w920:dbl)
    }
    frame #9 {
      w933 = dbl[] []
      n557 = while {
        shift-right: [w956] -> w929
        shift-left: w933 -> [w965]
        shift-right: [w963] -> w930
        shift-left: w933 -> [w964]
        tunnel: w932 -> [w960]
        tunnel: w931 -> [w959]
        shift-right: [w955] -> w928
        shift-left: w933 -> [w957]
        stop <- w949 stop-if-true
        n558 = local read "中间位置间隙"() -> (w946:dbl)
        n559 = local read "基准位移"() -> (w961:dbl)
        n560 = local read "间隙位移(mm)"() -> (w945:dbl)
        n561 = local read "电动缸位置(mm)"() -> (w935:dbl)
        n562 = call <userlib>:"Acm_AxGetCmdVelocity.vi"("AxisHandle"=w960) -> ("Velocity"=w954:dbl)  [unwired: 1 in, 3 out]
        n563 = local read "齿条推拉力(N)"() -> (w952:dbl)
        n564 = Subtract(x=w945, y=w961) -> (x-y=w948:dbl)
        n565 = Less Or Equal?(x=w945, y=0.0) -> (x <= y?=w944:bool)
        n566 = Greater Or Equal?(x=w945, y=4.0) -> (x >= y?=w943:bool)
        n567 = Subtract(x=w935, y=w959) -> (x-y=w939:dbl)
        n568 = Add(x=w948, y=w946) -> (x+y=w947:dbl)
        n569 = Multiply(x=w939, y=1.0) -> (x*y=w937:dbl)
        n570 = Build Array (concatenate) ("创建数组")(w964, w947) -> (w963:dbl[])
        n571 = Build Array (concatenate) ("创建数组")(w965, w937) -> (w956:dbl[])
        n572 = Or(x=w943, y=w944) -> (x .or. y?=w942:bool)
        n573 = Build Array (concatenate) ("创建数组")(w957, w952) -> (w955:dbl[])
        n574 = Greater Or Equal?(x=w952, y=500.0) -> (x >= y?=w950:bool)
        n575 = Equal To 0?(x=w954) -> (x = 0?=w951:bool)
        n576 = local read "循环退出"() -> (w934:bool)
        n577 = property on="间隙位移(mm)" class="DigNum (严格)"("Blinking"=w942) -> ()  [unwired: 2 in, 2 out]
        n578 = Bundle ("捆绑")(w956, w963) -> (w936:cluster{dbl[], dbl[]})  [unwired: 1 in]
        n579 = Compound Arithmetic op=OR(w951, w950, w934) -> (w949:bool)
        n580 = Bundle ("捆绑")(w956, w955) -> (w958:cluster{dbl[], dbl[]})  [unwired: 1 in]
        n581 = Build Array ("创建数组")(w936, w958) -> (w962:cluster{dbl[], dbl[]}[])
        n582 = local write "行程跳动曲线"(w962) -> ()
        n583 = Wait (ms)(milliseconds to wait=u32 50 ("毫秒倍数")) -> ()  [unwired: 1 out]
      }
    }
    frame #10 {
      n584 = local read "电动缸慢速"() -> (w967:dbl)
      n585 = local write "电动缸速度(mm/s)"(w967) -> ()
    }
    frame #11 {
      n586 = while {
        tunnel: w973 -> [w982]
        tunnel: [w981] -> w972
        stop <- w977 stop-if-true
        n587 = Wait Until Next ms Multiple(millisecond multiple=u32 50 ("毫秒倍数")) -> ()  [unwired: 1 out]
        n588 = local read "循环退出"() -> (w979:bool)
        n589 = call "PCI1240电动缸位置模式 .vi"("Distance"=-50.0, "AxisHandle IN"=w982) -> ("AbsSuccess"=w978:bool, "AxisHandle OUT"=w981:u32)  [unwired: 8 in]
        n590 = Compound Arithmetic op=OR(w978, w979) -> (w977:bool)
      }
    }
    frame #12 {
      n591 = local read "转向器中心"() -> (w985:dbl)
      n592 = while {
        shift-right: [w1014] -> w990
        shift-left: w987 -> [w1023]
        shift-right: [w1021] -> w991
        shift-left: w988 -> [w1022]
        tunnel: w984 -> [w1018]
        tunnel: w985 -> [w1017]
        shift-right: [w1013] -> w989
        shift-left: w986 -> [w1015]
        stop <- w1007 stop-if-true
        n593 = local read "中间位置间隙"() -> (w1004:dbl)
        n594 = local read "基准位移"() -> (w1019:dbl)
        n595 = local read "间隙位移(mm)"() -> (w1003:dbl)
        n596 = call <userlib>:"Acm_AxGetCmdVelocity.vi"("AxisHandle"=w1018) -> ("Velocity"=w1012:dbl)  [unwired: 1 in, 3 out]
        n597 = local read "电动缸位置(mm)"() -> (w993:dbl)
        n598 = Wait (ms)(milliseconds to wait=u32 50 ("毫秒倍数")) -> ()  [unwired: 1 out]
        n599 = local read "齿条推拉力(N)"() -> (w1010:dbl)
        n600 = Subtract(x=w1003, y=w1019) -> (x-y=w1006:dbl)
        n601 = Less Or Equal?(x=w1003, y=0.0) -> (x <= y?=w1002:bool)
        n602 = Greater Or Equal?(x=w1003, y=4.0) -> (x >= y?=w1001:bool)
        n603 = Subtract(x=w993, y=w1017) -> (x-y=w997:dbl)
        n604 = Add(x=w1006, y=w1004) -> (x+y=w1005:dbl)
        n605 = Multiply(x=w997, y=1.0) -> (x*y=w995:dbl)
        n606 = Build Array (concatenate) ("创建数组")(w1022, w1005) -> (w1021:dbl[])
        n607 = Build Array (concatenate) ("创建数组")(w1023, w995) -> (w1014:dbl[])
        n608 = Build Array (concatenate) ("创建数组")(w1015, w1010) -> (w1013:dbl[])
        n609 = Greater Or Equal?(x=w1010, y=500.0) -> (x >= y?=w1008:bool)
        n610 = local read "循环退出"() -> (w992:bool)
        n611 = Or(x=w1001, y=w1002) -> (x .or. y?=w1000:bool)
        n612 = Equal To 0?(x=w1012) -> (x = 0?=w1009:bool)
        n613 = property on="间隙位移(mm)" class="DigNum (严格)"("Blinking"=w1000) -> ()  [unwired: 2 in, 2 out]
        n614 = Bundle ("捆绑")(w1014, w1021) -> (w994:cluster{dbl[], dbl[]})  [unwired: 1 in]
        n615 = Compound Arithmetic op=OR(w1009, w1008, w992) -> (w1007:bool)
        n616 = Bundle ("捆绑")(w1014, w1013) -> (w1016:cluster{dbl[], dbl[]})  [unwired: 1 in]
        n617 = Build Array ("创建数组")(w994, w1016) -> (w1020:cluster{dbl[], dbl[]}[])
        n618 = local write "行程跳动曲线"(w1020) -> ()
      }
    }
    frame #13 {
      n619 = call "间隙计算.vi"("扭矩数组"=w1044) -> ("峰值间隙1"=w1036:dbl, "峰值间隙2"=w1035:dbl)  [unwired: 6 in, 3 out]
      n620 = call "功能计算_何 截取位移左.vi"("位移数组"=w1028, "拉压力数组"=w1042, "半行程"="半行程", "截取百分比"="截取百分比") -> ("峰值扭矩"=w1041:dbl, "平均扭矩"=w1040:dbl, "扭差"=w1039:dbl)  [unwired: 12 in, 1 out]
      "左最大轴向力(N)" <- w1041
      "左轴向力波动(N)" <- w1039
      "左平均轴向力(N)" <- w1040
      n621 = while {
        tunnel: w1043 -> [w1050]
        tunnel: [w1049] -> w1026
        stop <- w1045 stop-if-true
        n622 = local read "循环退出"() -> (w1047:bool)
        n623 = call "PCI1220U停止.vi"("AxisHandle IN"=w1050) -> ("完成"=w1046:bool, "AxisHandle OUT"=w1049:u32)  [unwired: 9 in]
        n624 = Wait (ms)(milliseconds to wait=u32 50 ("毫秒倍数")) -> ()  [unwired: 1 out]
        n625 = Compound Arithmetic op=OR(w1046, w1047) -> (w1045:bool)
      }
      n626 = Array Size(array=w1028) -> (size(s)=→"左轴向力数组大小":i32)
      n627 = local read "全行程180°外间隙标准(mm)"() -> (w1033:dbl)
      n628 = local read "全行程180°内间隙标准(mm)"() -> (w1034:dbl)
      n629 = local write "左180°内全行程间隙"(w1036) -> ()
      n630 = local write "左180°外全行程间隙"(w1035) -> ()
      n631 = local read "电动缸快速"() -> (w1025:dbl)
      n632 = Less?(x=w1035, y=w1033) -> (x < y?=w1037:bool)
      n633 = Less?(x=w1036, y=w1034) -> (x < y?=w1038:bool)
      n634 = Not(x=w1037) -> (.not. x?=w1031:bool)
      n635 = local write "电动缸速度(mm/s)"(w1025) -> ()
      n636 = Not(x=w1038) -> (.not. x?=w1032:bool)
      n637 = property on="左180°外全行程间隙" class="DigNum (严格)"("Blinking"=w1031) -> ()  [unwired: 2 in, 2 out]
      n638 = property on="左180°内全行程间隙" class="DigNum (严格)"("Blinking"=w1032) -> ()  [unwired: 2 in, 2 out]
    }
    frame #14 {
      n639 = local read "最大轴向力标准(N)"() -> (w1059:dbl)
      n640 = while {
        tunnel: w1065 -> [w1073]
        stop <- w1068 stop-if-true
        n641 = local read "齿条左极限"() -> (w1071:dbl)
        n642 = Wait Until Next ms Multiple(millisecond multiple=u32 50 ("毫秒倍数")) -> ()  [unwired: 1 out]
        n643 = local read "循环退出"() -> (w1070:bool)
        n644 = call "PCI1240电动缸位置模式 .vi"("Distance"=w1071, "AxisHandle IN"=w1073) -> ("AbsSuccess"=w1069:bool)  [unwired: 8 in, 1 out]
        n645 = Compound Arithmetic op=OR(w1069, w1070) -> (w1068:bool)
      }
      n646 = local read "轴向力标准(N)"() -> (w1058:dbl)
      n647 = local read "平均轴向力MAX(N)"() -> (w1057:dbl)
      n648 = local read "力波动标准(N)"() -> (w1056:dbl)
      n649 = call "判断.vi"("y 3"=w1056, "y 2-2"=w1057, "y 2-1"=w1058, "y"=w1059, "x 3"=w1062, "x 2"=w1063, "x"=w1061) -> ("非x? 3"=w1054:bool, "非x? 2"=w1060:bool, "非x?"=w1055:bool)  [unwired: 2 in]
      n650 = property on="左最大轴向力(N)" class="DigNum (严格)"("Blinking"=w1055) -> ()  [unwired: 2 in, 2 out]
      n651 = property on="左轴向力波动(N)" class="DigNum (严格)"("Blinking"=w1054) -> ()  [unwired: 2 in, 2 out]
      n652 = property on="左平均轴向力(N)" class="DigNum (严格)"("Blinking"=w1060) -> ()  [unwired: 2 in, 2 out]
      n653 = local read "转向器中心"() -> (w1051:dbl)
    }
    frame #15 {
      n654 = while {
        shift-right: [w1091] -> w1079
        shift-left: w1082 -> [w1119]
        shift-right: [w1117] -> w1080
        shift-left: w1083 -> [w1118]
        tunnel: w1074 -> [w1114]
        tunnel: w1078 -> [w1113]
        shift-right: [w1110] -> w1077
        shift-left: w1081 -> [w1111]
        stop <- w1105 stop-if-true
        n655 = local read "电动缸位置(mm)"() -> (w1087:dbl)
        n656 = call <userlib>:"Acm_AxGetCmdVelocity.vi"("AxisHandle"=w1114) -> ("Velocity"=w1103:dbl)  [unwired: 1 in, 3 out]
        n657 = local read "间隙位移(mm)"() -> (w1097:dbl)
        n658 = local read "基准位移"() -> (w1115:dbl)
        n659 = Wait (ms)(milliseconds to wait=u32 50 ("毫秒倍数")) -> ()  [unwired: 1 out]
        n660 = local read "中间位置间隙"() -> (w1102:dbl)
        n661 = local read "齿条推拉力(N)"() -> (w1109:dbl)
        n662 = Subtract(x=w1097, y=w1115) -> (x-y=w1116:dbl)
        n663 = local read "循环退出"() -> (w1086:bool)
        n664 = Subtract(x=w1087, y=2.7) -> (x-y=w1088:dbl)
        n665 = Subtract(x=w1088, y=w1113) -> (x-y=w1095:dbl)
        n666 = Add(x=w1116, y=w1102) -> (x+y=w1104:dbl)
        n667 = Less Or Equal?(x=w1109, y=-500.0) -> (x <= y?=w1106:bool)
        n668 = Equal To 0?(x=w1103) -> (x = 0?=w1107:bool)
        n669 = Multiply(x=w1095, y=1.0) -> (x*y=w1093:dbl)
        n670 = Build Array (concatenate) ("创建数组")(w1119, w1093) -> (w1091:dbl[])
        n671 = Build Array (concatenate) ("创建数组")(w1111, w1109) -> (w1110:dbl[])
        n672 = Build Array (concatenate) ("创建数组")(w1118, w1104) -> (w1117:dbl[])
        n673 = Compound Arithmetic op=OR(w1107, w1106, w1086) -> (w1105:bool)
        n674 = Bundle ("捆绑")(w1091, w1117) -> (w1092:cluster{dbl[], dbl[]})  [unwired: 1 in]
        n675 = Bundle ("捆绑")(w1091, w1110) -> (w1112:cluster{dbl[], dbl[]})  [unwired: 1 in]
        n676 = Build Array ("创建数组")(w1092, w1112) -> (w1090:cluster{dbl[], dbl[]}[])
        n677 = Less Or Equal?(x=w1097, y=0.0) -> (x <= y?=w1101:bool)
        n678 = Greater Or Equal?(x=w1097, y=4.0) -> (x >= y?=w1100:bool)
        n679 = Or(x=w1100, y=w1101) -> (x .or. y?=w1096:bool)
        n680 = local write "行程跳动曲线"(w1090) -> ()
        n681 = property on="间隙位移(mm)" class="DigNum (严格)"("Blinking"=w1096) -> ()  [unwired: 2 in, 2 out]
      }
    }
    frame #16 {
      n682 = local read "电动缸慢速"() -> (w1121:dbl)
      n683 = local write "电动缸速度(mm/s)"(w1121) -> ()
    }
    frame #17 {
      n684 = while {
        tunnel: w1130 -> [w1144]
        stop <- w1139 stop-if-true
        n685 = Wait Until Next ms Multiple(millisecond multiple=u32 50 ("毫秒倍数")) -> ()  [unwired: 1 out]
        n686 = call "PCI1240电动缸位置模式 .vi"("Distance"=130.0, "AxisHandle IN"=w1144) -> ("AbsSuccess"=w1140:bool)  [unwired: 8 in, 1 out]
        n687 = local read "循环退出"() -> (w1141:bool)
        n688 = Compound Arithmetic op=OR(w1140, w1141) -> (w1139:bool)
      }
      n689 = local read "转向器中心"() -> (w1131:dbl)
    }
    frame #18 {
      n690 = while {
        shift-right: [w1162] -> w1155
        shift-left: w1150 -> [w1190]
        shift-right: [w1188] -> w1156
        shift-left: w1151 -> [w1189]
        tunnel: w1145 -> [w1185]
        tunnel: w1149 -> [w1184]
        shift-right: [w1181] -> w1154
        shift-left: w1148 -> [w1182]
        stop <- w1176 stop-if-true
        n691 = local read "电动缸位置(mm)"() -> (w1158:dbl)
        n692 = call <userlib>:"Acm_AxGetCmdVelocity.vi"("AxisHandle"=w1185) -> ("Velocity"=w1174:dbl)  [unwired: 1 in, 3 out]
        n693 = local read "间隙位移(mm)"() -> (w1168:dbl)
        n694 = local read "基准位移"() -> (w1186:dbl)
        n695 = Wait (ms)(milliseconds to wait=u32 50 ("毫秒倍数")) -> ()  [unwired: 1 out]
        n696 = local read "中间位置间隙"() -> (w1173:dbl)
        n697 = local read "齿条推拉力(N)"() -> (w1180:dbl)
        n698 = local read "循环退出"() -> (w1157:bool)
        n699 = Subtract(x=w1168, y=w1186) -> (x-y=w1187:dbl)
        n700 = Subtract(x=w1158, y=2.7) -> (x-y=w1159:dbl)
        n701 = Subtract(x=w1159, y=w1184) -> (x-y=w1166:dbl)
        n702 = Add(x=w1187, y=w1173) -> (x+y=w1175:dbl)
        n703 = Multiply(x=w1166, y=1.0) -> (x*y=w1164:dbl)
        n704 = Less Or Equal?(x=w1180, y=-500.0) -> (x <= y?=w1177:bool)
        n705 = Build Array (concatenate) ("创建数组")(w1190, w1164) -> (w1162:dbl[])
        n706 = Build Array (concatenate) ("创建数组")(w1182, w1180) -> (w1181:dbl[])
        n707 = Equal To 0?(x=w1174) -> (x = 0?=w1178:bool)
        n708 = Build Array (concatenate) ("创建数组")(w1189, w1175) -> (w1188:dbl[])
        n709 = Bundle ("捆绑")(w1162, w1181) -> (w1183:cluster{dbl[], dbl[]})  [unwired: 1 in]
        n710 = Compound Arithmetic op=OR(w1178, w1177, w1157) -> (w1176:bool)
        n711 = Bundle ("捆绑")(w1162, w1188) -> (w1163:cluster{dbl[], dbl[]})  [unwired: 1 in]
        n712 = Build Array ("创建数组")(w1163, w1183) -> (w1161:cluster{dbl[], dbl[]}[])
        n713 = Less Or Equal?(x=w1168, y=0.0) -> (x <= y?=w1172:bool)
        n714 = Greater Or Equal?(x=w1168, y=4.0) -> (x >= y?=w1171:bool)
        n715 = Or(x=w1171, y=w1172) -> (x .or. y?=w1167:bool)
        n716 = local write "行程跳动曲线"(w1161) -> ()
        n717 = property on="间隙位移(mm)" class="DigNum (严格)"("Blinking"=w1167) -> ()  [unwired: 2 in, 2 out]
      }
    }
    frame #19 {
      n718 = while {
        tunnel: w1192 -> [w1210]
        tunnel: [w1209] -> _
        stop <- w1205 stop-if-true
        n719 = call "PCI1220U停止.vi"("AxisHandle IN"=w1210) -> ("完成"=w1206:bool, "AxisHandle OUT"=w1209:u32)  [unwired: 9 in]
        n720 = Wait (ms)(milliseconds to wait=u32 50 ("毫秒倍数")) -> ()  [unwired: 1 out]
        n721 = local read "循环退出"() -> (w1207:bool)
        n722 = Compound Arithmetic op=OR(w1206, w1207) -> (w1205:bool)
      }
      n723 = Array Max & Min(array=w1198) -> (max value=w1202:dbl, min value=w1201:dbl)  [unwired: 2 out]
      n724 = local read "左轴向力数组大小"() -> (w1193:i32)
      n725 = Absolute Value(x=w1202) -> (abs(x)=w1200:dbl)
      n726 = Absolute Value(x=w1201) -> (abs(x)=w1199:dbl)
      n727 = local write "右全行程间隙"(w1199) -> ()
      n728 = local write "左全行程间隙"(w1200) -> ()
    }
    frame #20 {
      (unwired) 46.996 ("y")
      n729 = local read "半行程"() -> (w1216:dbl)
      n730 = local read "全行程180°外间隙标准(mm)"() -> (w1251:dbl)
      n731 = Split 1D Array(array=w1213, index=w1211) -> (second subarray=w1214:dbl[])  [unwired: 1 out]
      n732 = local read "截取百分比"() -> (w1215:dbl)
      n733 = Split 1D Array(array=w1255, index=w1211) -> (second subarray=w1217:dbl[])  [unwired: 1 out]
      n734 = local read "全行程180°外间隙标准(mm)"() -> (w1233:dbl)
      n735 = local read "全行程180°内间隙标准(mm)"() -> (w1234:dbl)
      n736 = Array Max & Min(array=w1213) -> (max value=w1247:dbl, min value=w1246:dbl)  [unwired: 2 out]
      n737 = local read "总行程标准(mm)"() -> (w1228:dbl)
      n738 = call "功能计算_何 截取位移右.vi"("位移数组"=w1214, "拉压力数组"=w1217, "半行程"=w1216, "截取百分比"=w1215) -> ("峰值扭矩"=w1244:dbl, "平均扭矩"=w1254:dbl, "扭差"=w1243:dbl)  [unwired: 12 in, 1 out]
      n739 = Split 1D Array(array=w1236, index=w1211) -> (second subarray=w1235:dbl[])  [unwired: 1 out]
      n740 = Subtract(x=w1247, y=w1246) -> (x-y=w1238:dbl)
      n741 = Subtract(x=w1238, y="机械间隙值") -> (x-y=w1220:dbl)
      n742 = local write "总行程(mm)"(w1220) -> ()
      n743 = local write "右最大轴向力(N)"(w1244) -> ()
      n744 = Greater?(x=w1253, y=w1251) -> (0:w1240:bool)
      n745 = call "间隙计算.vi"("扭矩数组"=w1235) -> ("峰值间隙1"=w1250:dbl, "峰值间隙2"=w1249:dbl)  [unwired: 6 in, 3 out]
      n746 = Greater?(x=w1252, y=w1251) -> (0:w1239:bool)
      n747 = local write "右轴向力波动(N)"(w1243) -> ()
      n748 = local write "右平均轴向力(N)"(w1254) -> ()
      n749 = local read "总行程最大值"() -> (w1229:dbl)
      n750 = In Range and Coerce "判定范围并强制转换"(upper limit=w1229, x=w1220, lower limit=w1228) -> (In Range?=w1226:bool)  [unwired: 1 out]
      n751 = Less?(x=w1249, y=w1233) -> (x < y?=w1227:bool)
      n752 = Less?(x=w1250, y=w1234) -> (x < y?=w1248:bool)
      n753 = local write "右180°外全行程间隙"(w1249) -> ()
      n754 = local read "总圈数最大值"() -> (w1230:dbl)
      n755 = local write "右180°内全行程间隙"(w1250) -> ()
      n756 = property on="左全行程间隙" class="DigNum (严格)"("Blinking"=w1240) -> ()  [unwired: 2 in, 2 out]
      n757 = property on="右全行程间隙" class="DigNum (严格)"("Blinking"=w1239) -> ()  [unwired: 2 in, 2 out]
      n758 = Divide(x=w1220, y="齿条传动比") -> (x/y=w1232:dbl)
      n759 = Not(x=w1248) -> (.not. x?=w1222:bool)
      n760 = Not(x=w1227) -> (.not. x?=w1221:bool)
      n761 = property on="右180°外全行程间隙" class="DigNum (严格)"("Blinking"=w1221) -> ()  [unwired: 2 in, 2 out]
      n762 = local read "总圈数标准"() -> (w1231:dbl)
      n763 = In Range and Coerce(upper limit=w1230, x=w1232, lower limit=w1231) -> (In Range?=w1225:bool)  [unwired: 1 out]
      n764 = Not(x=w1226) -> (.not. x?=w1224:bool)
      n765 = local read "最大轴向力标准(N)"() -> (w1212:dbl)
      n766 = local write "总圈数"(w1232) -> ()
      n767 = Not(x=w1225) -> (.not. x?=w1223:bool)
      n768 = property on="总行程(mm)" class="DigNum (严格)"("Blinking"=w1224) -> ()  [unwired: 2 in, 2 out]
      n769 = property on="右180°内全行程间隙" class="DigNum (严格)"("Blinking"=w1222) -> ()  [unwired: 2 in, 2 out]
      n770 = property on="总圈数" class="DigNum (严格)"("Blinking"=w1223) -> ()  [unwired: 2 in, 2 out]
      "轴向力X" <- w1213
      "轴向力Y" <- w1255
    }
    frame #21 {
      n771 = local read "电动缸快速"() -> (w1257:dbl)
      n772 = local read "转向器中心"() -> (w1277:dbl)
      n773 = local read "平均轴向力MAX(N)"() -> (w1271:dbl)
      n774 = local read "轴向力标准(N)"() -> (w1272:dbl)
      n775 = local read "力波动标准(N)"() -> (w1270:dbl)
      n776 = call "判断.vi"("y 3"=w1270, "y 2-2"=w1271, "y 2-1"=w1272, "y"=w1258, "x 3"=w1273, "x 2"=w1280, "x"=w1276) -> ("非x? 3"=w1274:bool, "非x? 2"=w1275:bool, "非x?"=w1265:bool)  [unwired: 2 in]
      n777 = local write "电动缸速度(mm/s)"(w1257) -> ()
      n778 = property on="右最大轴向力(N)" class="DigNum (严格)"("Blinking"=w1265) -> ()  [unwired: 2 in, 2 out]
      n779 = property on="右平均轴向力(N)" class="DigNum (严格)"("Blinking"=w1275) -> ()  [unwired: 2 in, 2 out]
      n780 = Add(x=w1277, y=-10.0) -> (x+y=w1278:dbl)
    }
    frame #22 {
      n781 = Compound Arithmetic op=OR(w1287, w1294, w1293, w1292, w1285, w1284, w1288, w1291, w1290, w1286, w1283, w1282) -> (w1289:bool)
      n782 = property on="右轴向力波动(N)" class="DigNum (严格)"("Blinking"=w1288) -> ()  [unwired: 2 in, 2 out]
      n783 = Not(x=w1289) -> (.not. x?=w1295:bool)
      n784 = local write "全行程间隙及轴向力合格"(w1295) -> ()
    }
    frame #23 {
      n785 = while {
        tunnel: w1302 -> [w1306]
        tunnel: [w1304] -> w1301
        tunnel: w1300 -> [w1303]
        stop <- w1305 stop-if-true
        n786 = call "PCI1240电动缸位置模式 .vi"("Distance"=w1303, "AxisHandle IN"=w1306) -> ("AbsSuccess"=w1305:bool, "AxisHandle OUT"=w1304:u32)  [unwired: 8 in]
        n787 = Wait (ms)(milliseconds to wait=u32 50 ("毫秒倍数")) -> ()  [unwired: 1 out]
      }
    }
    frame #24 {
      n788 = while {
        tunnel: w1309 -> [w1313]
        stop <- w1311 stop-if-true
        n789 = call <userlib>:"Acm_AxGetCmdVelocity.vi"("AxisHandle"=w1313) -> ("Velocity"=w1312:dbl)  [unwired: 1 in, 3 out]
        n790 = Wait Until Next ms Multiple(millisecond multiple=u32 50 ("毫秒倍数")) -> ()  [unwired: 1 out]
        n791 = Equal To 0?(x=w1312) -> (x = 0?=w1311:bool)
      }
    }
    frame #25 {
      n792 = while {
        tunnel: w1316 -> [w1320]
        tunnel: [w1318] -> w1315
        tunnel: w1314 -> [w1317]
        stop <- w1319 stop-if-true
        n793 = call "PCI1240电动缸位置模式 .vi"("Distance"=w1317, "AxisHandle IN"=w1320) -> ("AbsSuccess"=w1319:bool, "AxisHandle OUT"=w1318:u32)  [unwired: 8 in]
        n794 = Wait (ms)(milliseconds to wait=u32 50 ("毫秒倍数")) -> ()  [unwired: 1 out]
      }
    }
    frame #26 {
      n795 = while {
        tunnel: w1322 -> [w1326]
        stop <- w1324 stop-if-true
        n796 = call <userlib>:"Acm_AxGetCmdVelocity.vi"("AxisHandle"=w1326) -> ("Velocity"=w1325:dbl)  [unwired: 1 in, 3 out]
        n797 = Wait Until Next ms Multiple(millisecond multiple=u32 50 ("毫秒倍数")) -> ()  [unwired: 1 out]
        n798 = Equal To 0?(x=w1325) -> (x = 0?=w1324:bool)
      }
    }
    frame #27 {
      n799 = local read "轴向力已做次数"() -> (w1329:dbl)
      n800 = Add(x=w1329, y=1.0) -> (x+y=w1327:dbl)
      n801 = local write "轴向力已做次数"(w1327) -> ()
    }
    frame #28 {
      n802 = local read "全行程间隙及轴向力合格"() -> (w1330:bool)
      n803 = case shown="假" w1330 {
        frame False {
          n804 = Less?(x="轴向力已做次数", y="设定轴向力调整次数") -> (x < y?=w1332:bool)
          n805 = case shown="真" w1332 {
            frame False {
              n806 = local write "工步号"(u32 45 ("工步号")) -> ()
            }
            frame True {
              n807 = local write "工步号"(u32 30 ("工步号")) -> ()
            }
          }
        }
        frame True {
          n808 = local write "工步号"(u32 45 ("工步号")) -> ()
        }
      }
    }
  }
  n809 = while {
    stop <- w1337 stop-if-true
    n810 = event shown="[3] \"参数查询\": 值改变" {
      selector: _ -> [_ _ _ _ _ _ _]
      dyn-events: _ -> [_ _ _ _ _ _ _]
      timeout: 500 -> [_ _ _ _ _ _ _]
      event Timeout {
        n811 = event-data() -> ()  [unwired: 3 out]
      }
      event "停止": Value Change {
        n812 = event-data() -> ()  [unwired: 6 out]
        n813 = flat-sequence {
          frame #0 {
            n814 = Wait (ms)(milliseconds to wait=u32 1000 ("毫秒倍数")) -> ()  [unwired: 1 out]
          }
          frame #1 {
            n815 = Quit LabVIEW(quit? (T)=TRUE ("停止？(T)")) -> ()
          }
        }
      }
      event "参数修改": Value Change {
        n816 = event-data() -> ()  [unwired: 6 out]
        n817 = while {
          i -> [w1389]
          stop <- w1388 stop-if-true
          n818 = local read "型号数量"() -> (w1390:i32)
          n819 = local read "参数浏览表"() -> (w1391:string[][])
          n820 = Greater Or Equal?(x=w1389, y=w1390) -> (x >= y?=w1388:bool)
          n821 = Wait Until Next ms Multiple(millisecond multiple=u32 50 ("毫秒倍数")) -> ()  [unwired: 1 out]
          n822 = Index Array(array=w1391, index (col)=w1389) -> (element=w1376:string[])  [unwired: 1 in]
          n823 = Index Array(array=w1376, index #1=0 ("索引"), index #2=2 ("索引"), index #3=3 ("索引"), index #4=4 ("索引"), index #5=5 ("索引"), index #6=6 ("索引"), index #7=7 ("索引"), index #8=8 ("索引"), index #9=9 ("索引"), index #10=10 ("索引"), index #11=11 ("索引"), index #12=12 ("索引"), index #13=13 ("索引"), index #14=14 ("索引"), index #15=15 ("索引"), index #16=16 ("索引"), index #17=17 ("索引"), index #18=18 ("索引"), index #19=19 ("索引"), index #20=20 ("索引")) -> (element #1=w1343:string, element #2=w1372:string, element #3=w1371:string, element #4=w1370:string, element #5=w1369:string, element #6=w1368:string, element #7=w1367:string, element #8=w1366:string, element #9=w1365:string, element #10=w1364:string, element #11=w1363:string, element #12=w1358:string, element #13=w1357:string, element #14=w1356:string, element #15=w1355:string, element #16=w1354:string, element #17=w1349:string, element #18=w1348:string, element #19=w1347:string, element #20=w1342:string)
          n824 = call "创建文本"("测头机构轴移动速度"=w1372, "测头机构轴检测位"=w1371, "测头机构轴待检位"=w1370, "测头机构轴后退位"=w1369, "齿条移动速度"=w1368, "齿条左极限"=w1367, "齿条右极限"=w1366, "旋转齿条轴找帽转速"=w1365, "旋转齿条轴测量转速"=w1364, "测量点扭矩"=w1363, "总行程最大值"=w1357, "总行程最小值"=w1358, "最大轴向力"=w1356, "轴向力波动"=w1355, "平均轴向力最小值"=w1354, "平均轴向力最大值"=w1349, "总圈数最小值"=w1348, "总圈数最大值"=w1347, "中间位置"=w1342, "产品型号"=w1343) -> ("Result"=w1362:string)  [unwired: 6 in, 1 out]
          n825 = local read "ADODB._Connection Out 2"() -> (w1361:refnum<k7>)
          n826 = call "SQL Execute.vi"("Command Text"=w1362, "ADODB._Connection In"=w1361) -> ("error out"=w1374:errorcluster, "ADODB._Connection Out"=w1375:refnum<k7>)  [unwired: 6 in, 2 out]
          n827 = call "ADO Connection Close.vi"("error in (no error)"=w1374, "ADODB._Connection In"=w1375) -> ("error out"=→"error out":errorcluster)  [unwired: 8 in, 1 out]
        }
      }
      event "参数查询": Value Change {
        n828 = event-data() -> ()  [unwired: 6 out]
        n829 = flat-sequence {
          tunnel: [w1404] -> w1397
          tunnel: [w1403] -> w1396
          tunnel: [w1402] -> w1393
          tunnel: w1397 -> [w1408]
          tunnel: w1396 -> [w1410]
          tunnel: [w1410] -> w1395
          tunnel: [w1409] -> w1394
          tunnel: w1393 -> [w1409]
          tunnel: w1395 -> [_]
          tunnel: w1394 -> [_]
          frame #0 {
            n830 = call-poly <vilib>:"Read From Spreadsheet File.vi"("file path (dialog if empty)"=path "D:/Q14070-Z060人机界面/参数/参数项.txt") -> ("first row"=w1398:string[])  [unwired: 6 in, 4 out]
            n831 = property on="参数浏览表" class="Tbl (严格)"("Row Headers[]"=w1398) -> ()  [unwired: 2 in, 2 out]
          }
          frame #1 {
            n832 = local read "ADODB._Connection Out 2"() -> (w1401:refnum<k7>)
            n833 = call "SQL Execute.vi"("Command Text"="SELECT * FROM 测试参数表;", "ADODB._Connection In"=w1401) -> ("error out"=w1402:errorcluster, "Data"=w1406:string[][], "ADODB._Connection Out"=w1403:refnum<k7>)  [unwired: 6 in, 1 out]
            n834 = Transpose 2D Array(2D array=w1406) -> (transposed array=w1404:string[][])
            n835 = Index Array(array=w1404, index (row)=0 ("索引 (行)")) -> (element=w1405:string[])  [unwired: 1 in]
            n836 = property on="参数浏览表" class="Tbl (严格)"("Column Headers[]"=w1405) -> ()  [unwired: 2 in, 2 out]
          }
          frame #2 {
            n837 = local write "参数浏览表"(w1408) -> ()
          }
          frame #3 {
          }
        }
      }
      event "传感器参数保存": Value Change {
        n838 = event-data() -> ()  [unwired: 6 out]
        n839 = flat-sequence {
          tunnel: [w1436] -> w1433
          tunnel: [w1435] -> w1432
          tunnel: [w1434] -> w1431
          tunnel: [w1442] -> w1430
          tunnel: w1433 -> [w1442]
          tunnel: [w1441] -> w1429
          tunnel: w1432 -> [w1441]
          tunnel: [w1440] -> w1428
          tunnel: w1431 -> [w1440]
          tunnel: [w1439] -> w1427
          tunnel: [w1438] -> w1426
          tunnel: [w1437] -> w1425
          tunnel: [w1443] -> w1424
          tunnel: [w1449] -> w1423
          tunnel: w1430 -> [w1449]
          tunnel: [w1448] -> w1422
          tunnel: w1429 -> [w1448]
          tunnel: w1428 -> [w1447]
          tunnel: [w1447] -> w1421
          tunnel: [w1446] -> w1420
          tunnel: w1427 -> [w1446]
          tunnel: [w1445] -> w1419
          tunnel: w1426 -> [w1445]
          tunnel: [w1444] -> w1418
          tunnel: w1425 -> [w1444]
          tunnel: w1424 -> [w1468]
          tunnel: [w1468] -> w1417
          tunnel: w1423 -> [w1467]
          tunnel: w1422 -> [w1460]
          tunnel: w1421 -> [w1459]
          tunnel: w1420 -> [w1453]
          tunnel: w1419 -> [w1452]
          tunnel: w1418 -> [w1458]
          tunnel: [w1457] -> w1416
          tunnel: [w1456] -> w1415
          tunnel: [w1455] -> w1414
          tunnel: [w1451] -> w1413
          tunnel: [w1450] -> w1412
          tunnel: [w1454] -> w1411
          tunnel: w1417 -> [w1476]
          tunnel: w1416 -> [w1475]
          tunnel: w1415 -> [w1474]
          tunnel: w1414 -> [w1473]
          tunnel: w1413 -> [w1472]
          tunnel: w1412 -> [w1471]
          tunnel: w1411 -> [w1470]
          frame #0 {
            n840 = local read "齿条推拉力零点偏移"() -> (w1435:dbl)
            n841 = local read "间隙位移零点偏移"() -> (w1436:dbl)
            n842 = local read "齿条扭矩零点偏移"() -> (w1434:dbl)
          }
          frame #1 {
            n843 = local read "齿条推拉力比例偏移"() -> (w1438:dbl)
            n844 = local read "间隙位移比例偏移"() -> (w1439:dbl)
            n845 = local read "齿条扭矩比例偏移"() -> (w1437:dbl)
          }
          frame #2 {
            n846 = local read "ADODB._Connection Out 2"() -> (w1443:refnum<k7>)
          }
          frame #3 {
            n847 = Number To Fractional String(number=w1467, precision (6)=i16 2 ("精度(6)")) -> (F-format string=w1457:string)  [unwired: 2 in]
            n848 = Number To Fractional String(number=w1459, precision (6)=i16 2 ("精度(6)")) -> (F-format string=w1455:string)  [unwired: 2 in]
            n849 = Number To Fractional String(number=w1458, precision (6)=i16 2 ("精度(6)")) -> (F-format string=w1454:string)  [unwired: 2 in]
            n850 = Number To Fractional String(number=w1460, precision (6)=i16 2 ("精度(6)")) -> (F-format string=w1456:string)  [unwired: 2 in]
            n851 = Number To Fractional String(number=w1453, precision (6)=i16 2 ("精度(6)")) -> (F-format string=w1451:string)  [unwired: 2 in]
            n852 = Number To Fractional String(number=w1452, precision (6)=i16 2 ("精度(6)")) -> (F-format string=w1450:string)  [unwired: 2 in]
          }
          frame #4 {
            n853 = call "创建文本3"("4"=w1472, "6"=w1470, "1"=w1475, "2"=w1474, "3"=w1473, "5"=w1471) -> ("Result"=w1477:string)  [unwired: 8 in, 1 out]
            n854 = call "SQL Execute.vi"("Command Text"=w1477, "ADODB._Connection In"=w1476) -> ("error out"=→"error out 4":errorcluster)  [unwired: 6 in, 3 out]
          }
        }
      }
      event "产品ID": Value Change {
        n855 = event-data() -> ()  [unwired: 7 out]
        n856 = Format Date/Time String(time format string (%c)="%Y%m%d%H%M" ("时间格式字符串(%c)")) -> (date/time string=w1478:string)  [unwired: 2 in]
        n857 = local write "KSJJ"(w1478) -> ()
      }
      event "电动缸回零": Mouse Down {
        n858 = event-data() -> ()  [unwired: 6 out]
        n859 = stacked-sequence {
          frame #0 {
            n860 = flat-sequence {
              tunnel: [w1498] -> w1487
              tunnel: [w1491] -> w1484
              tunnel: w1487 -> [w1501]
              tunnel: [w1501] -> w1486
              tunnel: [w1499] -> w1485
              tunnel: w1484 -> [w1499]
              tunnel: w1486 -> [w1503]
              tunnel: [w1503] -> w1488
              tunnel: w1485 -> [w1502]
              tunnel: [w1502] -> w1483
              tunnel: w1488 -> [w1514]
              tunnel: w1483 -> [w1513]
              tunnel: [w1512] -> w1482
              tunnel: w1482 -> [w1516]
              tunnel: [w1515] -> w1481
              tunnel: w1481 -> [w1524]
              frame #0 {
                n861 = local write "电动缸速度(mm/s)"(15.0 ("电动缸速度(mm/s)")) -> ()
                n862 = local write "测头机构轴速度(mm/s)"(10.0 ("电动缸速度(mm/s)")) -> ()
              }
              frame #1 {
                n863 = local read "测头机构电机"() -> (w1495:u32)
                n864 = local read "电动缸电机"() -> (w1492:u32)
                n865 = call <userlib>:"Acm_AxHome.vi"("DirMode"=u32 0, "HomeMode"=u32 11, "AxisHandle"=w1495) -> ("AxisHandle"=w1498:u32)  [unwired: 1 in, 2 out]
                n866 = call <userlib>:"Acm_AxHome.vi"("DirMode"=u32 1, "HomeMode"=u32 11, "AxisHandle"=w1492) -> ("AxisHandle"=w1491:u32)  [unwired: 1 in, 2 out]
              }
              frame #2 {
                n867 = Wait Until Next ms Multiple(millisecond multiple=u32 100 ("毫秒倍数")) -> ()  [unwired: 1 out]
              }
              frame #3 {
                n868 = while {
                  tunnel: w1503 -> [w1511]
                  stop <- w1509 stop-if-true
                  n869 = call <userlib>:"Acm_AxGetCmdVelocity.vi"("AxisHandle"=w1511) -> ("Velocity"=w1510:dbl)  [unwired: 1 in, 3 out]
                  n870 = Wait Until Next ms Multiple(millisecond multiple=u32 50 ("毫秒倍数")) -> ()  [unwired: 1 out]
                  n871 = Equal To 0?(x=w1510) -> (x = 0?=w1509:bool)
                }
                n872 = while {
                  tunnel: w1502 -> [w1507]
                  stop <- w1505 stop-if-true
                  n873 = call <userlib>:"Acm_AxGetCmdVelocity.vi"("AxisHandle"=w1507) -> ("Velocity"=w1506:dbl)  [unwired: 1 in, 3 out]
                  n874 = Wait Until Next ms Multiple(millisecond multiple=u32 50 ("毫秒倍数")) -> ()  [unwired: 1 out]
                  n875 = Equal To 0?(x=w1506) -> (x = 0?=w1505:bool)
                }
              }
              frame #4 {
                n876 = call "PCI1220U角度置零.vi"("AxisHandle IN"=w1514) -> ()  [unwired: 10 in, 1 out]
                n877 = call "PCI1220U角度置零.vi"("AxisHandle IN"=w1513) -> ("AxisHandle OUT"=w1512:u32)  [unwired: 10 in]
              }
              frame #5 {
                n878 = while {
                  tunnel: [w1522] -> w1515
                  tunnel: w1516 -> [w1517]
                  stop <- w1521 stop-if-true
                  n879 = Wait Until Next ms Multiple(millisecond multiple=u32 50 ("毫秒倍数")) -> ()  [unwired: 1 out]
                  n880 = local read "齿条右极限"() -> (w1520:dbl)
                  n881 = Add(x=w1520, y=-10.0) -> (x+y=w1518:dbl)
                  n882 = call "PCI1240电动缸位置模式 .vi"("Distance"=w1518, "AxisHandle IN"=w1517) -> ("AbsSuccess"=w1521:bool, "AxisHandle OUT"=w1522:u32)  [unwired: 8 in]
                }
              }
              frame #6 {
                n883 = while {
                  tunnel: w1524 -> [w1528]
                  stop <- w1526 stop-if-true
                  n884 = call <userlib>:"Acm_AxGetCmdVelocity.vi"("AxisHandle"=w1528) -> ("Velocity"=w1527:dbl)  [unwired: 1 in, 3 out]
                  n885 = Wait Until Next ms Multiple(millisecond multiple=u32 50 ("毫秒倍数")) -> ()  [unwired: 1 out]
                  n886 = Equal To 0?(x=w1527) -> (x = 0?=w1526:bool)
                }
              }
            }
          }
          frame #1 {
            n887 = flat-sequence {
              tunnel: [w1540] -> w1535
              tunnel: w1535 -> [w1542]
              tunnel: [w1542] -> w1534
              tunnel: w1534 -> [w1543]
              tunnel: [w1543] -> w1533
              tunnel: w1533 -> [w1549]
              tunnel: [w1548] -> w1530
              tunnel: w1530 -> [w1551]
              tunnel: [w1551] -> w1529
              tunnel: w1529 -> [w1553]
              tunnel: [w1552] -> w1532
              tunnel: w1532 -> [w1559]
              tunnel: [w1559] -> w1531
              tunnel: w1531 -> [w1564]
              frame #0 {
                n888 = local write "旋转伺服速度(°/s)"(5.0 ("电动缸速度(mm/s)")) -> ()
              }
              frame #1 {
                n889 = local read "旋转齿条电机"() -> (w1537:u32)
                n890 = call <userlib>:"Acm_AxHome.vi"("DirMode"=u32 0, "HomeMode"=u32 11, "AxisHandle"=w1537) -> ("AxisHandle"=w1540:u32)  [unwired: 1 in, 2 out]
              }
              frame #2 {
                n891 = Wait Until Next ms Multiple(millisecond multiple=u32 100 ("毫秒倍数")) -> ()  [unwired: 1 out]
              }
              frame #3 {
                n892 = while {
                  tunnel: w1543 -> [w1547]
                  stop <- w1545 stop-if-true
                  n893 = call <userlib>:"Acm_AxGetCmdVelocity.vi"("AxisHandle"=w1547) -> ("Velocity"=w1546:dbl)  [unwired: 1 in, 3 out]
                  n894 = Wait Until Next ms Multiple(millisecond multiple=u32 50 ("毫秒倍数")) -> ()  [unwired: 1 out]
                  n895 = Equal To 0?(x=w1546) -> (x = 0?=w1545:bool)
                }
              }
              frame #4 {
                n896 = call "PCI1220U角度置零.vi"("AxisHandle IN"=w1549) -> ("AxisHandle OUT"=w1548:u32)  [unwired: 10 in]
              }
              frame #5 {
                n897 = Wait (ms)(milliseconds to wait=u32 100 ("等待时间（毫秒）")) -> ()  [unwired: 1 out]
              }
              frame #6 {
                n898 = while {
                  tunnel: [w1557] -> w1552
                  tunnel: w1553 -> [w1554]
                  stop <- w1556 stop-if-true
                  n899 = Wait Until Next ms Multiple(millisecond multiple=u32 50 ("毫秒倍数")) -> ()  [unwired: 1 out]
                  n900 = call "PCI1220U扭矩轴位置模式.vi"("Distance"=15.0, "AxisHandle IN"=w1554) -> ("AbsSuccess"=w1556:bool, "AxisHandle OUT"=w1557:u32)  [unwired: 8 in]
                }
              }
              frame #7 {
                n901 = while {
                  tunnel: w1559 -> [w1562]
                  stop <- w1560 stop-if-true
                  n902 = call <userlib>:"Acm_AxGetCmdVelocity.vi"("AxisHandle"=w1562) -> ("Velocity"=w1563:dbl)  [unwired: 1 in, 3 out]
                  n903 = Wait Until Next ms Multiple(millisecond multiple=u32 50 ("毫秒倍数")) -> ()  [unwired: 1 out]
                  n904 = Equal To 0?(x=w1563) -> (x = 0?=w1560:bool)
                }
              }
              frame #8 {
                n905 = call "PCI1220U角度置零.vi"("AxisHandle IN"=w1564) -> ()  [unwired: 10 in, 1 out]
              }
            }
          }
          frame #2 {
            n906 = flat-sequence {
              frame #0 {
                n907 = while {
                  stop <- w1568 stop-if-true
                  n908 = local read "电动缸回零"() -> (w1569:bool)
                  n909 = local write "回零完成"(TRUE ("回零完成")) -> ()
                  n910 = local write "电动缸回零"(FALSE ("电动缸回零")) -> ()
                  n911 = Wait Until Next ms Multiple(millisecond multiple=u32 50 ("毫秒倍数")) -> ()  [unwired: 1 out]
                  n912 = Not(x=w1569) -> (.not. x?=w1568:bool)
                }
              }
            }
          }
        }
        n913 = Wait Until Next ms Multiple(millisecond multiple=u32 50 ("毫秒倍数")) -> ()  [unwired: 1 out]
      }
    }
    n914 = Wait (ms)(milliseconds to wait=u32 50 ("毫秒倍数")) -> ()  [unwired: 1 out]
    n915 = local read "停止"() -> (w1337:bool)
  }
  n916 = call "PCI1240电动缸位置模式 .vi"() -> ()  [unwired: 10 in, 2 out]
  n917 = while {
    stop <- w1571 stop-if-true
    n918 = stacked-sequence {
      frame #0 {
        n919 = flat-sequence {
          frame #0 {
          }
          frame #1 {
            n920 = First Call?() -> (First Call?: T/F=w1572:bool)
            n921 = case shown="真" w1572 {
              frame False {
              }
              frame True {
                n922 = call "员工管理测试程序.vi"() -> ("员工姓名"=w1574:string, "员工ID"=w1573:string)  [unwired: 10 in]
                n923 = local write "员工ID"(w1573) -> ()
                n924 = local write "员工姓名"(w1574) -> ()
              }
            }
          }
          frame #2 {
          }
          frame #3 {
          }
          frame #4 {
          }
          frame #5 {
          }
          frame #6 {
          }
        }
      }
      frame #1 {
        n925 = flat-sequence {
          frame #0 {
            n926 = property on="型号选择" class="Ring (严格)"() -> ("RingText.Text"=w1578:string)  [unwired: 2 in, 2 out]
            n927 = case shown="\"J706\"" w1578 {
              frame "J706" {
                w1579 = FALSE ("可见")
                w1580 = TRUE ("可见")
                n928 = property on="左180°内全行程间隙" class="DigNum (严格)"("Visible"=w1580) -> ()  [unwired: 2 in, 2 out]
                n929 = property on="左180°外全行程间隙" class="DigNum (严格)"("Visible"=w1580) -> ()  [unwired: 2 in, 2 out]
                n930 = property on="右180°外全行程间隙" class="DigNum (严格)"("Visible"=w1580) -> ()  [unwired: 2 in, 2 out]
                n931 = property on="右180°内全行程间隙" class="DigNum (严格)"("Visible"=w1580) -> ()  [unwired: 2 in, 2 out]
                n932 = property on="左全行程间隙" class="DigNum (严格)"("Visible"=w1579) -> ()  [unwired: 2 in, 2 out]
                n933 = property on="右全行程间隙" class="DigNum (严格)"("Visible"=w1579) -> ()  [unwired: 2 in, 2 out]
              }
              frame "J728" {
                w1581 = FALSE ("可见")
                w1582 = TRUE ("可见")
                n934 = property on="左180°内全行程间隙" class="DigNum (严格)"("Visible"=w1582) -> ()  [unwired: 2 in, 2 out]
                n935 = property on="左180°外全行程间隙" class="DigNum (严格)"("Visible"=w1582) -> ()  [unwired: 2 in, 2 out]
                n936 = property on="右180°外全行程间隙" class="DigNum (严格)"("Visible"=w1582) -> ()  [unwired: 2 in, 2 out]
                n937 = property on="右180°内全行程间隙" class="DigNum (严格)"("Visible"=w1582) -> ()  [unwired: 2 in, 2 out]
                n938 = property on="左全行程间隙" class="DigNum (严格)"("Visible"=w1581) -> ()  [unwired: 2 in, 2 out]
                n939 = property on="右全行程间隙" class="DigNum (严格)"("Visible"=w1581) -> ()  [unwired: 2 in, 2 out]
              }
              frame "J709", Default {
                w1583 = TRUE ("可见")
                w1584 = FALSE ("可见")
                n940 = property on="左180°内全行程间隙" class="DigNum (严格)"("Visible"=w1584) -> ()  [unwired: 2 in, 2 out]
                n941 = property on="左180°外全行程间隙" class="DigNum (严格)"("Visible"=w1584) -> ()  [unwired: 2 in, 2 out]
                n942 = property on="右180°外全行程间隙" class="DigNum (严格)"("Visible"=w1584) -> ()  [unwired: 2 in, 2 out]
                n943 = property on="右180°内全行程间隙" class="DigNum (严格)"("Visible"=w1584) -> ()  [unwired: 2 in, 2 out]
                n944 = property on="左全行程间隙" class="DigNum (严格)"("Visible"=w1583) -> ()  [unwired: 2 in, 2 out]
                n945 = property on="右全行程间隙" class="DigNum (严格)"("Visible"=w1583) -> ()  [unwired: 2 in, 2 out]
              }
            }
          }
          frame #1 {
            (unwired) string[] ["I急停按钮", "I自动旋钮", "I启动按钮", "I备用按钮", "I复位按钮", "I上阻挡器放行", "I下阻挡器放行", "I进支线按钮"] ("I0说明")
            (unwired) string[] ["I出支线按钮", "I主线顶升按钮", "I主线下降按钮", "I支线顶升按钮", "I支线下降按钮", "I气压报警", "未使用", "未使用"] ("I0说明")
            n946 = local read "间隙位移(mm)"() -> (w1587:dbl)
            n947 = Greater Or Equal?(x=w1587, y=7.0) -> (x >= y?=w1585:bool)
            n948 = case shown="真" w1585 {
              frame False {
              }
              frame True {
                n949 = local write "测头机构轴使能"(FALSE ("测头机构轴使能")) -> ()
              }
            }
          }
          frame #2 {
            (unwired) string[] ["I电动缸SRDY", "I电动缸ZSPD", "I电动缸ALRM", "I间隙进给SRDY", "I间隙进给ZSPD", "I间隙进给ALRM", "I间隙旋转SRPD", "I间隙旋转ZSPD"] ("I0说明")
            n950 = local read "测头机构轴位置(mm)"() -> (w1591:dbl)
            n951 = Greater Or Equal?(x=w1591, y=90.0) -> (x >= y?=w1589:bool)
            n952 = case shown="假" w1589 {
              frame False {
                w1592 = T5."Enabled" ("禁用")
                n953 = property on="测头气缸左移" class="Bool (严格)"("DisabledEnum"=w1592) -> ()  [unwired: 2 in, 2 out]
                n954 = property on="测头气缸右移" class="Bool (严格)"("DisabledEnum"=w1592) -> ()  [unwired: 2 in, 2 out]
                n955 = property on="测头气缸左移" class="Bool"("DisabledEnum"=w1592) -> ()  [unwired: 2 in, 2 out]
                n956 = property on="测头气缸右移" class="Bool"("DisabledEnum"=w1592) -> ()  [unwired: 2 in, 2 out]
              }
              frame True {
                w1593 = T5."Disabled" ("禁用")
                w1594 = FALSE ("测头气缸右移")
                n957 = local write "测头气缸右移"(w1594) -> ()
                n958 = local write "测头气缸左移"(w1594) -> ()
                n959 = property on="测头气缸左移" class="Bool (严格)"("DisabledEnum"=w1593) -> ()  [unwired: 2 in, 2 out]
                n960 = property on="测头气缸右移" class="Bool (严格)"("DisabledEnum"=w1593) -> ()  [unwired: 2 in, 2 out]
                n961 = property on="测头气缸左移" class="Bool"("DisabledEnum"=w1593) -> ()  [unwired: 2 in, 2 out]
                n962 = property on="测头气缸右移" class="Bool"("DisabledEnum"=w1593) -> ()  [unwired: 2 in, 2 out]
              }
            }
          }
          frame #3 {
            (unwired) string[] ["I间隙旋转ALRM", "I扭矩旋转SRPD", "I扭矩旋转ZSPD", "I扭矩旋转ALRM", "I拧紧机合格", "I拧紧机不合格", "I拧紧机报警", "未使用"] ("I0说明")
          }
        }
        n963 = local read "急停"() -> (w1577:bool)
        n964 = local read "复位"() -> (w1576:bool)
        n965 = Compound Arithmetic op=OR(invert w1577, w1576) -> (→"循环退出":bool)
      }
      frame #2 {
        n966 = flat-sequence {
          frame #0 {
            (unwired) string[] ["I自制气缸进位", "I自制气缸原位", "I上工位检测", "I本工位检测", "I下工位检测", "I主线顶升上位", "I主线顶升下位", "I支线顶升上位"] ("I0说明")
          }
          frame #1 {
            (unwired) string[] ["I支线顶升下位", "I支线进到位", "I支线退到位", "I位移气缸原位", "I位移气缸进位", "I拧紧机在位", "I电动缸原位", "I电动缸进位"] ("I0说明")
          }
          frame #2 {
            (unwired) string[] ["未使用", "未使用", "未使用", "未使用", "未使用", "未使用", "未使用", "未使用"] ("I0说明")
          }
          frame #3 {
            (unwired) string[] ["未使用", "未使用", "未使用", "未使用", "未使用", "未使用", "未使用", "未使用"] ("I0说明")
          }
        }
        n967 = local read "下工位测试H"() -> (w1596:bool)
        n968 = local read "下工位备料H"() -> (w1595:bool)
        n969 = local read "下工位自动H"() -> (w1597:bool)
        n970 = local write "下工位备料"(w1595) -> ()
        n971 = local write "下工位测试"(w1596) -> ()
        n972 = local write "下工位自动"(w1597) -> ()
      }
      frame #3 {
        n973 = local read "工步号"() -> (w1601:u32)
        n974 = local read "报警"() -> (w1599:dbl)
        n975 = case shown="50" w1601 {
          tunnel: [w1612 "请取胶瓶" ("工步描述") "请取扳手加力" ("工步描述") "灵敏度测试中" ("工步描述") "有油刚度测试中" ("工步描述") "点击启动按钮进行测试" ("工步描述") "电动缸前进找中" ("工步描述") "气缸右移" ("工步描述") "电动缸前进找中" ("工步描述") "找中结束开始测间隙" ("工步描述") "力特性试验中" ("工步描述") "轴向力测试中" ("工步描述") "探头气缸左移，电动缸后退" ("工步描述") "等待放行" ("工步描述") "电动缸回零" ("工步描述") "力特性试验完成" ("工步描述") "套好输出轴把手，按启动按钮，做回正力试验" ("工步描述") "回正力试验中" ("工步描述") "试验完成，将把手拉回，取下油管，按顶升按钮" ("工步描述") "拆下锁紧螺母和输入轴万向节，按顶升按钮" ("工步描述")] -> w1600
          frame 0, Default {
            n976 = local read "联线按钮"() -> (w1611:bool)
            n977 = case shown="假" w1611 {
              tunnel: ["等待工件" ("工步描述") "等待扫描条码" ("工步描述")] -> w1612
              frame False {
              }
              frame True {
              }
            }
          }
          frame 1 {
          }
          frame 2 {
          }
          frame 3 {
          }
          frame 4 {
          }
          frame 6 {
          }
          frame 7 {
          }
          frame 10 {
          }
          frame 15 {
          }
          frame 20 {
          }
          frame 30 {
          }
          frame 40 {
          }
          frame 45 {
          }
          frame 100 {
          }
          frame 50 {
          }
          frame 55 {
          }
          frame 60 {
          }
          frame 70 {
          }
          frame 80 {
          }
          frame 56 {
          }
        }
        "工步提示" <- w1600
        n978 = case shown="9" w1599 {
          tunnel: [_ "探头气缸不在原位" "操作步骤错误请取胶瓶" "操作步骤错误请加力" "急停被按下" "气压报警" "电动缸伺服报警" "旋转伺服报警" "测头伺服报警" "操作步骤错误请点标后放行"] -> w1598
          frame 0, Default {
          }
          frame 1 {
          }
          frame 2 {
          }
          frame 3 {
          }
          frame 4 {
          }
          frame 5 {
          }
          frame 6 {
          }
          frame 7 {
          }
          frame 8 {
          }
          frame 9 {
          }
        }
        n979 = local write "报警提示"(w1598) -> ()
      }
      frame #4 {
        n980 = local read "急停"() -> (w1634:bool)
        n981 = local read "红灯"() -> (w1636:bool)
        n982 = local read "复位"() -> (w1637:bool)
        n983 = local read "复位"() -> (w1639:bool)
        n984 = local read "红灯"() -> (w1638:bool)
        n985 = case shown="真" w1634 {
          frame False {
            "红灯" <- TRUE ("红灯")
          }
          frame True {
            n986 = local write "红灯"(FALSE ("红灯")) -> ()
          }
        }
        n987 = Or(x=w1636, y=w1637) -> (x .or. y?=w1635:bool)
        n988 = case shown="真" w1635 {
          frame False {
          }
          frame True {
            n989 = local write "回零完成"(FALSE ("夹头夹紧控制")) -> ()
          }
        }
        n990 = local read "停止"() -> (w1641:bool)
        n991 = Compound Arithmetic op=OR(w1639, w1641, w1638) -> (w1640:bool)
        n992 = case shown="真" w1640 {
          frame False {
          }
          frame True {
            n993 = local read "测头机构电机"() -> (w1645:u32)
            n994 = local read "旋转齿条电机"() -> (w1646:u32)
            n995 = local read "电动缸电机"() -> (w1647:u32)
            n996 = call "PCI1220U停止.vi"("AxisHandle IN"=w1646) -> ()  [unwired: 9 in, 2 out]
            n997 = call "PCI1220U停止.vi"("AxisHandle IN"=w1647) -> ()  [unwired: 9 in, 2 out]
            n998 = call "PCI1220U停止.vi"("AxisHandle IN"=w1645) -> ()  [unwired: 9 in, 2 out]
          }
        }
      }
      frame #5 {
        n999 = local read "齿条扭矩(Nm)"() -> (w1650:dbl)
        n1000 = local read "黄灯"() -> (w1648:bool)
        n1001 = local read "旋转齿条轴左转"() -> (w1656:bool)
        n1002 = Absolute Value(x=w1650) -> (abs(x)=w1655:dbl)
        n1003 = local read "旋转齿条轴右转"() -> (w1651:bool)
        n1004 = Not(x=w1656) -> (.not. x?=w1652:bool)
        n1005 = Less?(x=w1655, y=20.0) -> (x < y?=w1653:bool)
        n1006 = Compound Arithmetic op=AND(w1651, w1652, w1653, w1648) -> (w1649:bool)
        n1007 = case shown="真" w1649 {
          frame False {
          }
          frame True {
            n1008 = flat-sequence {
              tunnel: [w1660] -> w1658
              tunnel: w1658 -> [w1662]
              tunnel: [w1662] -> w1657
              tunnel: w1657 -> [w1673]
              frame #0 {
                n1009 = local read "旋转齿条电机"() -> (w1659:u32)
                n1010 = call "PCI1220U运行.vi"("方向"=enum32{"Negative", "Positive"}."Negative" ("Direction"), "AxisHandle IN"=w1659) -> ("AxisHandle OUT"=w1660:u32)  [unwired: 9 in]
              }
              frame #1 {
                n1011 = while {
                  stop <- w1666 stop-if-true
                  n1012 = Wait (ms)(milliseconds to wait=u32 50 ("毫秒倍数")) -> ()  [unwired: 1 out]
                  n1013 = local read "齿条扭矩(Nm)"() -> (w1671:dbl)
                  n1014 = local read "旋转齿条轴右转"() -> (w1668:bool)
                  n1015 = local read "红灯"() -> (w1663:bool)
                  n1016 = local read "复位"() -> (w1664:bool)
                  n1017 = Absolute Value(x=w1671) -> (abs(x)=w1670:dbl)
                  n1018 = Not(x=w1668) -> (.not. x?=w1665:bool)
                  n1019 = Greater?(x=w1670, y=10.0) -> (0:w1667:bool)
                  n1020 = Compound Arithmetic op=OR(w1667, w1665, w1664, w1663) -> (w1666:bool)
                }
              }
              frame #2 {
                n1021 = call "PCI1220U停止.vi"("AxisHandle IN"=w1673) -> ()  [unwired: 9 in, 2 out]
              }
            }
          }
        }
      }
      frame #6 {
        n1022 = local read "齿条扭矩(Nm)"() -> (w1678:dbl)
        n1023 = local read "旋转齿条轴右转"() -> (w1682:bool)
        n1024 = Absolute Value(x=w1678) -> (abs(x)=w1677:dbl)
        n1025 = local read "旋转齿条轴左转"() -> (w1680:bool)
        n1026 = local read "黄灯"() -> (w1674:bool)
        n1027 = Not(x=w1682) -> (.not. x?=w1679:bool)
        n1028 = Less?(x=w1677, y=20.0) -> (x < y?=w1675:bool)
        n1029 = Compound Arithmetic op=AND(w1680, w1679, w1675, w1674) -> (w1681:bool)
        n1030 = case shown="真" w1681 {
          frame False {
          }
          frame True {
            n1031 = flat-sequence {
              tunnel: [w1686] -> w1684
              tunnel: w1684 -> [w1688]
              tunnel: [w1688] -> w1683
              tunnel: w1683 -> [w1699]
              frame #0 {
                n1032 = local read "旋转齿条电机"() -> (w1685:u32)
                n1033 = call "PCI1220U运行.vi"("方向"=enum32{"Negative", "Positive"}."Positive" ("Direction"), "AxisHandle IN"=w1685) -> ("AxisHandle OUT"=w1686:u32)  [unwired: 9 in]
              }
              frame #1 {
                n1034 = while {
                  stop <- w1691 stop-if-true
                  n1035 = Wait (ms)(milliseconds to wait=u32 50 ("毫秒倍数")) -> ()  [unwired: 1 out]
                  n1036 = local read "齿条扭矩(Nm)"() -> (w1697:dbl)
                  n1037 = local read "旋转齿条轴左转"() -> (w1694:bool)
                  n1038 = local read "红灯"() -> (w1689:bool)
                  n1039 = local read "复位"() -> (w1690:bool)
                  n1040 = Absolute Value(x=w1697) -> (abs(x)=w1696:dbl)
                  n1041 = Not(x=w1694) -> (.not. x?=w1692:bool)
                  n1042 = Greater?(x=w1696, y=10.0) -> (0:w1693:bool)
                  n1043 = Compound Arithmetic op=OR(w1690, w1689, w1693, w1692) -> (w1691:bool)
                }
              }
              frame #2 {
                n1044 = call "PCI1220U停止.vi"("AxisHandle IN"=w1699) -> ()  [unwired: 9 in, 2 out]
              }
            }
          }
        }
      }
      frame #7 {
        n1045 = local read "齿条推拉力(N)"() -> (w1704:dbl)
        n1046 = local read "电动缸前进"() -> (w1701:bool)
        n1047 = local read "电动缸后退"() -> (w1700:bool)
        n1048 = Absolute Value(x=w1704) -> (abs(x)=w1708:dbl)
        n1049 = local read "黄灯"() -> (w1702:bool)
        n1050 = Not(x=w1700) -> (.not. x?=w1705:bool)
        n1051 = Less?(x=w1708, y=1000.0) -> (x < y?=w1706:bool)
        n1052 = Compound Arithmetic op=AND(w1701, w1705, w1702, w1706) -> (w1703:bool)
        n1053 = case shown="真" w1703 {
          frame False {
          }
          frame True {
            n1054 = flat-sequence {
              tunnel: [w1712] -> w1710
              tunnel: w1710 -> [w1714]
              tunnel: [w1714] -> w1709
              tunnel: w1709 -> [w1725]
              frame #0 {
                n1055 = local read "电动缸电机"() -> (w1711:u32)
                n1056 = call "PCI1220U运行.vi"("方向"=enum32{"Negative", "Positive"}."Positive" ("Direction"), "AxisHandle IN"=w1711) -> ("AxisHandle OUT"=w1712:u32)  [unwired: 9 in]
              }
              frame #1 {
                n1057 = while {
                  stop <- w1722 stop-if-true
                  n1058 = local read "电动缸前进"() -> (w1719:bool)
                  n1059 = local read "齿条推拉力(N)"() -> (w1716:dbl)
                  n1060 = Wait (ms)(milliseconds to wait=u32 50 ("毫秒倍数")) -> ()  [unwired: 1 out]
                  n1061 = Absolute Value(x=w1716) -> (abs(x)=w1718:dbl)
                  n1062 = local read "红灯"() -> (w1720:bool)
                  n1063 = local read "复位"() -> (w1721:bool)
                  n1064 = Greater?(x=w1718, y=1000.0) -> (0:w1715:bool)
                  n1065 = Not(x=w1719) -> (.not. x?=w1723:bool)
                  n1066 = Compound Arithmetic op=OR(w1721, w1720, w1723, w1715) -> (w1722:bool)
                }
              }
              frame #2 {
                n1067 = call "PCI1220U停止.vi"("AxisHandle IN"=w1725) -> ()  [unwired: 9 in, 2 out]
              }
            }
          }
        }
      }
      frame #8 {
        n1068 = local read "电动缸前进"() -> (w1726:bool)
        n1069 = local read "齿条推拉力(N)"() -> (w1730:dbl)
        n1070 = local read "电动缸后退"() -> (w1727:bool)
        n1071 = Absolute Value(x=w1730) -> (abs(x)=w1734:dbl)
        n1072 = local read "黄灯"() -> (w1728:bool)
        n1073 = Not(x=w1726) -> (.not. x?=w1731:bool)
        n1074 = Less?(x=w1734, y=1000.0) -> (x < y?=w1732:bool)
        n1075 = Compound Arithmetic op=AND(w1727, w1731, w1728, w1732) -> (w1729:bool)
        n1076 = case shown="真" w1729 {
          frame False {
          }
          frame True {
            n1077 = flat-sequence {
              tunnel: [w1738] -> w1736
              tunnel: w1736 -> [w1740]
              tunnel: [w1740] -> w1735
              tunnel: w1735 -> [w1751]
              frame #0 {
                n1078 = local read "电动缸电机"() -> (w1737:u32)
                n1079 = call "PCI1220U运行.vi"("方向"=enum32{"Negative", "Positive"}."Negative" ("Direction"), "AxisHandle IN"=w1737) -> ("AxisHandle OUT"=w1738:u32)  [unwired: 9 in]
              }
              frame #1 {
                n1080 = while {
                  stop <- w1748 stop-if-true
                  n1081 = local read "电动缸后退"() -> (w1745:bool)
                  n1082 = local read "齿条推拉力(N)"() -> (w1744:dbl)
                  n1083 = Wait (ms)(milliseconds to wait=u32 50 ("毫秒倍数")) -> ()  [unwired: 1 out]
                  n1084 = Absolute Value(x=w1744) -> (abs(x)=w1742:dbl)
                  n1085 = local read "红灯"() -> (w1747:bool)
                  n1086 = local read "复位"() -> (w1746:bool)
                  n1087 = Greater?(x=w1742, y=1000.0) -> (0:w1741:bool)
                  n1088 = Not(x=w1745) -> (.not. x?=w1749:bool)
                  n1089 = Compound Arithmetic op=OR(w1746, w1747, w1749, w1741) -> (w1748:bool)
                }
              }
              frame #2 {
                n1090 = call "PCI1220U停止.vi"("AxisHandle IN"=w1751) -> ()  [unwired: 9 in, 2 out]
              }
            }
          }
        }
      }
      frame #9 {
        n1091 = local read "测头机构轴后退"() -> (w1752:bool)
        n1092 = local read "测头机构轴前进"() -> (w1753:bool)
        n1093 = local read "黄灯"() -> (w1754:bool)
        n1094 = Not(x=w1752) -> (.not. x?=w1756:bool)
        n1095 = Compound Arithmetic op=AND(w1753, w1756, w1754) -> (w1755:bool)
        n1096 = case shown="真" w1755 {
          frame False {
          }
          frame True {
            n1097 = flat-sequence {
              tunnel: [w1760] -> w1758
              tunnel: w1758 -> [w1762]
              tunnel: [w1762] -> w1757
              tunnel: w1757 -> [w1769]
              frame #0 {
                n1098 = local read "测头机构电机"() -> (w1759:u32)
                n1099 = call "PCI1220U运行.vi"("方向"=enum32{"Negative", "Positive"}."Positive" ("Direction"), "AxisHandle IN"=w1759) -> ("AxisHandle OUT"=w1760:u32)  [unwired: 9 in]
              }
              frame #1 {
                n1100 = while {
                  stop <- w1766 stop-if-true
                  n1101 = local read "测头机构轴前进"() -> (w1763:bool)
                  n1102 = Wait (ms)(milliseconds to wait=u32 50 ("毫秒倍数")) -> ()  [unwired: 1 out]
                  n1103 = local read "红灯"() -> (w1764:bool)
                  n1104 = local read "复位"() -> (w1765:bool)
                  n1105 = Not(x=w1763) -> (.not. x?=w1767:bool)
                  n1106 = Compound Arithmetic op=OR(w1765, w1764, w1767) -> (w1766:bool)
                }
              }
              frame #2 {
                n1107 = call "PCI1220U停止.vi"("AxisHandle IN"=w1769) -> ()  [unwired: 9 in, 2 out]
              }
            }
          }
        }
      }
      frame #10 {
        n1108 = local read "测头机构轴前进"() -> (w1770:bool)
        n1109 = local read "测头机构轴后退"() -> (w1771:bool)
        n1110 = local read "黄灯"() -> (w1772:bool)
        n1111 = Not(x=w1770) -> (.not. x?=w1774:bool)
        n1112 = Compound Arithmetic op=AND(w1771, w1774, w1772) -> (w1773:bool)
        n1113 = case shown="真" w1773 {
          frame False {
          }
          frame True {
            n1114 = flat-sequence {
              tunnel: [w1778] -> w1776
              tunnel: w1776 -> [w1780]
              tunnel: [w1780] -> w1775
              tunnel: w1775 -> [w1787]
              frame #0 {
                n1115 = local read "测头机构电机"() -> (w1777:u32)
                n1116 = call "PCI1220U运行.vi"("方向"=enum32{"Negative", "Positive"}."Negative" ("Direction"), "AxisHandle IN"=w1777) -> ("AxisHandle OUT"=w1778:u32)  [unwired: 9 in]
              }
              frame #1 {
                n1117 = while {
                  stop <- w1784 stop-if-true
                  n1118 = local read "测头机构轴后退"() -> (w1781:bool)
                  n1119 = Wait (ms)(milliseconds to wait=u32 50 ("毫秒倍数")) -> ()  [unwired: 1 out]
                  n1120 = local read "红灯"() -> (w1783:bool)
                  n1121 = local read "复位"() -> (w1782:bool)
                  n1122 = Not(x=w1781) -> (.not. x?=w1785:bool)
                  n1123 = Compound Arithmetic op=OR(w1782, w1783, w1785) -> (w1784:bool)
                }
              }
              frame #2 {
                n1124 = call "PCI1220U停止.vi"("AxisHandle IN"=w1787) -> ()  [unwired: 9 in, 2 out]
              }
            }
          }
        }
      }
    }
    n1125 = Wait (ms)(milliseconds to wait=u32 50 ("毫秒倍数")) -> ()  [unwired: 1 out]
    n1126 = local read "停止"() -> (w1571:bool)
  }
  n1127 = flat-sequence {
    tunnel: [w1791] -> w128
    tunnel: [w1789] -> w127
    tunnel: w128 -> [w1801]
    tunnel: w127 -> [w1800]
    frame #0 {
      n1128 = First Call?() -> (First Call?: T/F=w1788:bool)
      n1129 = case shown="真" w1788 {
        frame False {
        }
        frame True {
          n1130 = while {
            i -> [w1795]
            stop <- w1796 stop-if-true
            w1799 = TRUE ("电动缸使能")
            n1131 = Wait Until Next ms Multiple(millisecond multiple=u32 50 ("毫秒倍数")) -> ()  [unwired: 1 out]
            n1132 = local write "回零完成"(FALSE ("回零完成")) -> ()
            n1133 = local write "测头机构轴使能"(w1799) -> ()
            n1134 = local write "旋转齿条轴使能"(w1799) -> ()
            n1135 = local write "电动缸使能"(w1799) -> ()
            n1136 = Greater Or Equal?(x=w1795, y=u32 30) -> (x >= y?=w1796:bool)
          }
        }
      }
      n1137 = call "ADO Connection Create.vi"() -> ("error out"=w1792:errorcluster, "ADODB._Connection Out"=w1793:refnum<k7>)  [unwired: 10 in]
      n1138 = call "ADO Connection Open.vi"("error in (no error)"=w1792, "ConnectionString"="Provider=Microsoft.Jet.OLEDB.4.0;Data Source=D:\\Q14070-Z060人机界面\\参数\\参数Z060.mdb;Persist Security Info=False;Jet OLEDB:Database Password=123;", "ADODB._Connection In"=w1793) -> ("error out"=w1789:errorcluster, "ADODB._Connection Out"=w1791:refnum<k7>)  [unwired: 7 in]
    }
    frame #1 {
      n1139 = while {
        tunnel: w1801 -> [w1803]
        tunnel: w1800 -> [w1802]
        stop <- w1807 stop-if-true
        n1140 = Wait (ms)(milliseconds to wait=u32 50 ("等待时间（毫秒）")) -> ()  [unwired: 1 out]
        n1141 = First Call?() -> (First Call?: T/F=w1806:bool)
        n1142 = Or(x=w1806, y="参数加载") -> (x .or. y?=w1805:bool)
        n1143 = case shown="真" w1805 {
          tunnel: w1803 -> [_ w1810]
          tunnel: w1802 -> [_ w1809]
          frame False {
          }
          frame True {
            n1144 = stacked-sequence {
              tunnel: w1810 -> [w1816 w1865 w1884]
              tunnel: w1809 -> [w1811 _ _]
              frame #0 {
                n1145 = call "SQL Execute.vi"("error in (no error)"=w1811, "Command Text"="SELECT * FROM 测试参数表", "ADODB._Connection In"=w1816) -> ("Data"=w1814:string[][])  [unwired: 5 in, 3 out]
                n1146 = Index Array(array=w1814, index (col)=0 ("索引 (行)")) -> (element=w1818:string[])  [unwired: 1 in]
                n1147 = Array Size(array=w1818) -> (size(s)=w1813:i32)
                "型号数量" <- w1813
                n1148 = while {
                  shift-right: [w1825] -> w1817
                  shift-left: i32[] [] -> [w1824]
                  tunnel: w1813 -> [w1822]
                  i -> [w1823]
                  stop <- w1821 stop-if-true
                  n1149 = Greater Or Equal?(x=w1823, y=w1822) -> (x >= y?=w1821:bool)
                  n1150 = Build Array (concatenate)(w1824, w1823) -> (w1825:i32[])
                }
                n1151 = Build Cluster Array "索引与捆绑簇数组"(w1818, w1817) -> (w1812:cluster{"String":string, i32}[])
                n1152 = property on="型号选择" class="Ring (严格)"("StringsAndValues[]"=w1812) -> ()  [unwired: 2 in, 2 out]
              }
              frame #1 {
                n1153 = property on="型号选择" class="Ring (严格)"() -> ("RingText.Text"=w1866:string)  [unwired: 2 in, 2 out]
                n1154 = call "创建文本2"("型号选择"=w1866) -> ("Result"=w1870:string)  [unwired: 13 in, 1 out]
                n1155 = call "SQL Execute.vi"("Command Text"=w1870, "ADODB._Connection In"=w1865) -> ("Data"=w1869:string[][])  [unwired: 6 in, 3 out]
                n1156 = Index Array(array=w1869, index (row)=0 ("索引 (行)")) -> (element=w1867:string[])  [unwired: 1 in]
                n1157 = Fract/Exp String To Number ("分数/指数字符串至数值转换")(string=w1867) -> (number=w1854:dbl[])  [unwired: 3 in, 1 out]
                n1158 = Index Array ("索引数组")(array=w1854, index #1=2 ("索引"), index #2=3 ("索引"), index #3=4 ("索引"), index #4=5 ("索引"), index #5=6 ("索引"), index #6=7 ("索引"), index #7=8 ("索引"), index #8=9 ("索引"), index #9=10 ("索引"), index #10=11 ("索引"), index #11=12 ("索引"), index #12=13 ("索引"), index #13=14 ("索引"), index #14=15 ("索引"), index #15=16 ("索引"), index #16=17 ("索引"), index #17=18 ("索引"), index #18=19 ("索引"), index #19=20 ("索引")) -> (element #1=w1853:dbl, element #2=w1852:dbl, element #3=w1851:dbl, element #4=w1850:dbl, element #5=w1849:dbl, element #6=w1848:dbl, element #7=w1847:dbl, element #8=w1846:dbl, element #9=w1845:dbl, element #10=w1844:dbl, element #11=w1843:dbl, element #12=w1842:dbl, element #13=w1826:dbl, element #14=w1836:dbl, element #15=w1835:dbl, element #16=w1834:dbl, element #17=w1830:dbl, element #18=w1829:dbl, element #19=w1827:dbl)
                n1159 = local write "测头机构轴移动速度"(w1853) -> ()
                n1160 = local write "测头机构轴检测位"(w1852) -> ()
                n1161 = local write "测头机构轴后退位"(w1850) -> ()
                n1162 = local write "测头机构轴待检位"(w1851) -> ()
                n1163 = local write "旋转伺服找帽转速"(w1846) -> ()
                n1164 = local write "旋转伺服测量转速"(w1845) -> ()
                n1165 = local write "齿条移动速度"(w1849) -> ()
                n1166 = local write "总行程标准(mm)"(w1843) -> ()
                n1167 = local write "齿条左极限"(w1848) -> ()
                n1168 = local write "总行程最大值"(w1842) -> ()
                n1169 = local write "齿条右极限"(w1847) -> ()
                n1170 = local write "平均轴向力MAX(N)"(w1834) -> ()
                n1171 = local write "转向器中心"(w1827) -> ()
                n1172 = local write "总圈数标准"(w1830) -> ()
                n1173 = local write "总圈数最大值"(w1829) -> ()
                n1174 = local write "测量点扭矩"(w1844) -> ()
                n1175 = local write "力波动标准(N)"(w1836) -> ()
                n1176 = local write "轴向力标准(N)"(w1835) -> ()
                n1177 = local write "齿条传动比"(w1826) -> ()
              }
              frame #2 {
                n1178 = call "SQL Execute.vi"("Command Text"="SELECT * FROM 传感器校验表 where ID='1'", "ADODB._Connection In"=w1884) -> ("Data"=w1886:string[][])  [unwired: 6 in, 3 out]
                n1179 = Index Array(array=w1886) -> (element=w1887:string[])  [unwired: 2 in]
                n1180 = Fract/Exp String To Number ("分数/指数字符串至数值转换")(string=w1887) -> (number=w1877:dbl[])  [unwired: 3 in, 1 out]
                n1181 = Index Array(array=w1877, index #1=1 ("索引"), index #2=2 ("索引"), index #3=3 ("索引"), index #4=4 ("索引"), index #5=5 ("索引"), index #6=6 ("索引")) -> (element #1=w1876:dbl, element #2=w1875:dbl, element #3=w1874:dbl, element #4=w1873:dbl, element #5=w1872:dbl, element #6=w1871:dbl)
                n1182 = local write "间隙位移零点偏移"(w1876) -> ()
                n1183 = local write "间隙位移比例偏移"(w1875) -> ()
                n1184 = local write "齿条推拉力零点偏移"(w1874) -> ()
                n1185 = local write "齿条推拉力比例偏移"(w1873) -> ()
                n1186 = local write "齿条扭矩零点偏移"(w1872) -> ()
                n1187 = local write "齿条扭矩比例偏移"(w1871) -> ()
              }
            }
          }
        }
        n1188 = local read "停止"() -> (w1807:bool)
        "ADODB._Connection Out 2" <- w1803
      }
    }
  }
  n1189 = while {
    stop <- w1889 stop-if-true
    n1190 = local read "rfid工步号"() -> (w1888:u32)
    n1191 = case shown="10" w1888 {
      frame 0, Default {
      }
      frame 10 {
        n1192 = flat-sequence {
          tunnel: [w1899] -> w1893
          tunnel: w1893 -> [w1903]
          tunnel: [w1900] -> w1892
          tunnel: w1892 -> [w1905]
          tunnel: [w1905] -> w1891
          tunnel: w1891 -> [w1908]
          frame #0 {
            n1193 = while {
              stop <- w1894 stop-if-true
              n1194 = local read "rfid触发"() -> (w1894:bool)
              n1195 = Wait Until Next ms Multiple(millisecond multiple=u32 50 ("毫秒倍数")) -> ()  [unwired: 1 out]
            }
          }
          frame #1 {
            n1196 = local write "芯片ID"("" ("随行板ID")) -> ()
            n1197 = local write "rfid完成"(FALSE ("RFID完成")) -> ()
            n1198 = local write "rfid触发"(FALSE ("RFID读取触发")) -> ()
          }
          frame #2 {
            n1199 = local read "Z060ARFID"() -> (w1899:string)
            n1200 = local write "芯片ID"(w1899) -> ()
          }
          frame #3 {
            w1901 = T6 0 items=["两端", "字符串首端", "字符串末端"] ("location (both)")
            n1201 = call "查询产品ID.vi"("芯片编码"=w1903) -> ("产品ID"=w1902:string)  [unwired: 8 in, 2 out]
            "读取产品ID" <- w1902
            n1202 = call <vilib>:"Trim Whitespace.vi"("string"=w1902, "location (both)"=w1901) -> ("trimmed string"=w1900:string)
          }
          frame #4 {
            n1203 = Wait Until Next ms Multiple(millisecond multiple=u32 500 ("毫秒倍数")) -> ()  [unwired: 1 out]
          }
          frame #5 {
            n1204 = call "查询上序合格.vi"("产品ID"=w1908) -> ("本序已做"=w1906:bool, "上序合格"=w1907:bool)  [unwired: 8 in, 1 out]
            n1205 = Not(x=w1907) -> (.not. x?=w1909:bool)
            n1206 = local write "上序不合格"(w1909) -> ()
            n1207 = local write "上序合格"(w1907) -> ()
            n1208 = local write "本序已做"(w1906) -> ()
          }
          frame #6 {
            n1209 = local write "rfid完成"(TRUE ("RFID读取完成")) -> ()
            n1210 = Wait Until Next ms Multiple(millisecond multiple=u32 500 ("毫秒倍数")) -> ()  [unwired: 1 out]
          }
          frame #7 {
            "rfid工步号" <- 15.0 ("工步号")
          }
        }
      }
      frame 210 {
        n1211 = local read "读取产品ID"() -> (w1913:string)
        n1212 = local write "产品ID"(w1913) -> ()
      }
    }
    n1213 = Wait Until Next ms Multiple(millisecond multiple=u32 50 ("毫秒倍数")) -> ()  [unwired: 1 out]
    n1214 = local read "停止"() -> (w1889:bool)
  }
  n1215 = flat-sequence {
    tunnel: [w1914] -> w130
    tunnel: w130 -> [w1924]
    tunnel: [w1923] -> w129
    tunnel: w129 -> [w1994]
    frame #0 {
      n1216 = disable-structure shown="禁用" {
        disable-tunnel: [w1922 _] -> w1918
        disable-tunnel: [w1921 _] -> w1917
        disable-tunnel: [w1920 _] -> w1916
        disable-tunnel: [w1919 _] -> w1915
        frame Disabled {
          n1217 = call "PCI1240U初始化.vi"() -> ("旋转电机"=w1920:u32, "电动缸电机"=w1919:u32, "DeviceHandle"=w1922:u32, "进给电机"=w1921:u32)  [unwired: 6 in, 2 out]
        }
        frame Enabled {
        }
      }
      "DeviceHandle" <- w1918
      "电动缸电机" <- w1915
      "旋转齿条电机" <- w1916
      "测头机构电机" <- w1917
      n1218 = call "PCI8622配置.vi"() -> ("DeviceID"=w1914:i32)  [unwired: 11 in]
    }
    frame #1 {
      n1219 = while {
        tunnel: w1924 -> [w1926]
        tunnel: [w1925] -> w1923
        stop <- "停止" stop-if-true
        n1220 = stacked-sequence {
          tunnel: w1926 -> [_ _ w1970]
          tunnel: [_ _ w1970] -> w1925
          frame #0 {
            n1221 = local read "测头机构电机"() -> (w1935:u32)
            n1222 = Boolean To (0,1)(Boolean="测头机构轴使能") -> (0, 1=w1933:i16)
            n1223 = call <userlib>:"Acm_AxSetSvOn.vi"("OnOff"=w1933, "AxisHandle"=w1935) -> ("AxisHandle"=w1932:u32)  [unwired: 1 in, 2 out]
            n1224 = call "PCI1220U进给轴速度设置.vi"("Change Velocity"="测头机构轴速度(mm/s)", "AxisHandle IN"=w1932) -> ("AxisHandle OUT"=w1930:u32)  [unwired: 9 in]
            n1225 = call "PCI1220U进给轴读取位置.vi"("AxisHandle IN"=w1930) -> ("位置"=→"测头机构轴位置(mm)":dbl)  [unwired: 9 in, 1 out]
          }
          frame #1 {
            n1226 = local read "电动缸电机"() -> (w1945:u32)
            n1227 = local read "旋转齿条电机"() -> (w1944:u32)
            n1228 = Boolean To (0,1)(Boolean="电动缸使能") -> (0, 1=w1949:i16)
            n1229 = Boolean To (0,1)(Boolean="旋转齿条轴使能") -> (0, 1=w1943:i16)
            n1230 = call <userlib>:"Acm_AxSetSvOn.vi"("OnOff"=w1943, "AxisHandle"=w1944) -> ("AxisHandle"=w1946:u32)  [unwired: 1 in, 2 out]
            n1231 = call <userlib>:"Acm_AxSetSvOn.vi"("OnOff"=w1949, "AxisHandle"=w1945) -> ("AxisHandle"=w1948:u32)  [unwired: 1 in, 2 out]
            n1232 = call "PCI1220U扭矩轴速度设置.vi"("Change Velocity"="旋转伺服速度(°/s)", "AxisHandle IN"=w1946) -> ("AxisHandle OUT"=w1947:u32)  [unwired: 9 in]
            n1233 = call "PCI1240电动缸速度设置.vi"("Change Velocity"="电动缸速度(mm/s)", "AxisHandle IN"=w1948) -> ("AxisHandle OUT"=w1936:u32)  [unwired: 9 in]
            n1234 = call "PCI1220U扭矩轴读取位置.vi"("AxisHandle IN"=w1947) -> ("位置"=→"旋转伺服位置(°)":dbl)  [unwired: 9 in, 1 out]
            n1235 = call "PCI1240电动缸读取位置.vi"("AxisHandle IN"=w1936) -> ("位置"=→"电动缸位置(mm)":dbl)  [unwired: 9 in, 1 out]
          }
          frame #2 {
            w1986 = 0  # nRetSizeWords
            w1987 = 2048  # nReadSizeWords
            # "hDevice"
            n1236 = Initialize Array(u16 0, 2048 ("dimension size")) -> (w1977:u16[])
            n1237 = dll-call lib="PCI8622_32.dll" fn="PCI8622_ReadDeviceProAD_Npt" label="ReadDeviceProAD_Npt"("hDevice"=w1970, "ADBuffer[]"=w1977, "nReadSizeWords"=w1987, "nRetSizeWords"=w1986) -> ("ADBuffer[]"=w1980:u16[])  [unwired: 7 in, 2 out]
            n1238 = Divide(x=w1980, y=65536.01) -> (x/y=w1981:dbl[])
            n1239 = Multiply(x=w1981, y=20) -> (x*y=w1984:dbl[])
            n1240 = Subtract(x=w1984, y=10) -> (x-y=w1976:dbl[])
            n1241 = Decimate 1D Array ("抽取一维数组")(w1976) -> (w1964:dbl[], w1965:dbl[], w1963:dbl[])  [unwired: 5 out]
            n1242 = Add Array Elements(numeric array=w1964) -> (sum=w1973:dbl)
            n1243 = Add Array Elements(numeric array=w1963) -> (sum=w1974:dbl)
            n1244 = Array Size(array=w1964) -> (size(s)=w1972:i32)
            n1245 = Add Array Elements(numeric array=w1965) -> (sum=w1969:dbl)
            n1246 = Array Size(array=w1963) -> (size(s)=w1975:i32)
            n1247 = Array Size(array=w1965) -> (size(s)=w1971:i32)
            n1248 = Divide(x=w1973, y=w1972) -> (x/y=w1962:dbl)
            n1249 = Divide(x=w1974, y=w1975) -> (x/y=w1954:dbl)
            n1250 = Divide(x=w1969, y=w1971) -> (x/y=w1959:dbl)
            n1251 = Subtract(x=w1954, y=2.371) -> (x-y=w1952:dbl)
            n1252 = Multiply(x=w1962, y=2.0) -> (x*y=w1957:dbl)
            n1253 = Multiply(x=w1959, y=200.0) -> (x*y=w1958:dbl)
            n1254 = Subtract(x=w1957, y=-1.0) -> (x-y=w1955:dbl)
            n1255 = Multiply(x=w1952, y=0.75) -> (x*y=w1950:dbl)
            n1256 = local read "间隙位移比例偏移"() -> (w1991:dbl)
            n1257 = local read "间隙位移零点偏移"() -> (w1990:dbl)
            n1258 = local read "齿条扭矩零点偏移"() -> (w1992:dbl)
            n1259 = local read "齿条扭矩比例偏移"() -> (w1993:dbl)
            n1260 = local read "齿条推拉力比例偏移"() -> (w1989:dbl)
            n1261 = local read "齿条推拉力零点偏移"() -> (w1988:dbl)
            n1262 = call "传感器校订.vi"("零点"=w1992, "比例"=w1993, "传感器"=w1955) -> ("示值"=→"齿条扭矩(Nm)":dbl)  [unwired: 8 in]
            n1263 = call "传感器校订.vi"("零点"=w1990, "比例"=w1991, "传感器"=w1950) -> ("示值"=→"间隙位移(mm)":dbl)  [unwired: 8 in]
            n1264 = call "传感器校订.vi"("零点"=w1988, "比例"=w1989, "传感器"=w1958) -> ("示值"=→"齿条推拉力(N)":dbl)  [unwired: 8 in]
          }
        }
        n1265 = Wait Until Next ms Multiple(millisecond multiple=u32 50 ("毫秒倍数")) -> ()  [unwired: 1 out]
      }
    }
    frame #2 {
      n1266 = dll-call lib="PCI8622_32.dll" fn="PCI8622_StopDeviceProAD" label="StopDeviceProAD"("hDevice"=w1994) -> ("hDevice"=w1995:i32)  [unwired: 4 in, 2 out]
      n1267 = dll-call lib="PCI8622_32.dll" fn="PCI8622_ReleaseDeviceProAD" label="ReleaseDeviceProAD"("hDevice"=w1995) -> ()  [unwired: 5 in, 2 out]
      n1268 = dll-call lib="PCI8622_32.dll" fn="PCI8622_ReleaseDevice" label="ReleaseDevice"("hDevice"=w1994) -> ()  [unwired: 5 in, 2 out]
    }
  }
